vi "CRYO_MASTER_FULL_IP_old.vi"() -> ()   [LabVIEW 2017]
uses:
  USBData.lvclass
  LSI218Data.lvclass
  LSI336Data.lvclass
  <vilib>/DAQmx/create/channels.llb/DAQmx Create Channel (DO-Digital Output).vi
  <vilib>/Analysis/NI_AALBase.lvlib
  6240AData.lvclass
  <vilib>/DAQmx/create/channels.llb/DAQmx Create Channel (AO-Voltage-Basic).vi
  <vilib>/express/express arith-compare/Formula/XNode/ExpressFormulaBlockNode.xnode
  DMMsData.lvclass
panel:
  out "Graph 12":T1(graph) caption="XY Graph"
  out "Graph 11":T1(graph) caption="XY Graph"
  out "Graph 10":T1(graph) caption="XY Graph"
  in  "Automatic \nScreenshots?":bool=TRUE
  in  "Frontpanel screenshots":bool
  in  "Screenshots interval":i64=3605
  in  "Record interval":i64=10
  out "Cycle #":u32=4959
  in  "Measurement Interval (s)":dbl=1.0
  in  "Stop Button":bool
  in  "?":T2(tab)=enum."DIAGRAM"
  out "RUN Identifier":string="20201002_111738_PreCooling"
  in  "Base Path (screenshots)":path=path "C:/LabVIEW/DATA/Google/TUCAN Experiments/KEK_cryotests_2019-2020/data/screenshots"
  out "error out (USB6210/6218 AOUT)":errorcluster
  in  "AOUT 1 Label":string="KIKUSUI_I"
  in  "AOUT 0 Label":string="KIKUSUI_V"
  in  "DOUT Labels":string[](array[string])=["D_V1_NO", "D_V2_NC", "D_CV1"]
  in  "AOUT for Current CTRL":tag="Dev1/ao1"
  in  "AOUT For Voltage CTRL":tag="Dev1/ao0"
  out "AO task out":refnum<k21>="20201002_111738_PreCooling_AO"
  in  "Analog Out ON?":bool=TRUE
  in  "InstName (USB6218)":string="USB6218"
  in  "USB6218 Config":T3(array[cluster])=[{"Label"="F_1", "FileFormat"="%5.5f", "Active?"=TRUE, "Physical CH"="Dev1/ai0", " terminal\n type"=10083, "ConversionType"={"Type"=enum."SimpleProp", "ConversionParameters"=[0.0, 5.0, 0.0, 500.0]}, "VoltageLimits"=[0.0, 5.0]}, {"Label"="F_2", "FileFormat"="%5.5f", "Active?"=TRUE, "Physical CH"="Dev1/ai1", " terminal\n type"=10083, "ConversionType"={"Type"=enum."SimpleProp", "ConversionParameters"=[0.0, 5.0, 0.0, 200.0]}, "VoltageLimits"=[0.0, 5.0]}, {"Label"="F_3", "FileFormat"="%5.5f", "Active?"=TRUE, "Physical CH"="Dev1/ai2", " terminal\n type"=10083, "ConversionType"={"Type"=enum."SimpleProp", "ConversionParameters"=[0.0, 5.0, 0.0, 200.0]}, "VoltageLimits"=[0.0, 5.0]}, {"Label"="F_4", "FileFormat"="%5.5f", "Active?"=TRUE, "Physical CH"="Dev1/ai3", " terminal\n type"=10083, "ConversionType"={"Type"=enum."SimpleProp", "ConversionParameters"=[0.0, 5.0, 0.0, 500.0]}, "VoltageLimits"=[0.0, 5.0]}, {"Label"="F_5", "FileFormat"="%5.5f", "Active?"=TRUE, "Physical CH"="Dev1/ai4", " terminal\n type"=10083, "ConversionType"={"Type"=enum."SimpleProp", "ConversionParameters"=[0.0, 5.0, 0.0, 500.0]}, "VoltageLimits"=[0.0, 5.0]}, {"Label"="I_CV", "FileFormat"="%3.5f", "Active?"=TRUE, "Physical CH"="Dev1/ai5", " terminal\n type"=10083, "ConversionType"={"Type"=enum."Raw", "ConversionParameters"=[0.0, 0.0, 0.0, 0.0]}, "VoltageLimits"=[0.0, 10.0]}, {"Label"="CV1_answer", "FileFormat"="%3.5f", "Active?"=TRUE, "Physical CH"="Dev1/ai6", " terminal\n type"=10083, "ConversionType"={"Type"=enum."SimpleProp", "ConversionParameters"=[1.0, 5.0, 0.0, 100.0]}, "VoltageLimits"=[0.0, 5.0]}] {"terminal\n type" items=["Default"=-1, "RSE"=10083, "NRSE"=10078, "Differential"=10106, "Pseudodifferential"=12529]}
  out "error out (USB6218)":errorcluster
  out "error out (USB6210/6218 DOUT)":errorcluster
  out "DOUT task out":refnum<k21>="20201002_111738_DO"
  in  "DOUT Physical CH":tag[](array[tag])=["Dev1/port1/line0", "Dev1/port1/line1", "Dev1/port1/line2"]
  in  "Digital Out ON?":bool=TRUE
  in  "USB6210 Config":T3(array[cluster])=[{"Label"="P_ins", "FileFormat"="%5.5e", "Active?"=TRUE, "Physical CH"="Dev2/ai0", " terminal\n type"=10083, "ConversionType"={"Type"=enum."CC-10_LOG", "ConversionParameters"=[0.5, 9.0, 0.0, 1.0]}, "VoltageLimits"=[0.0, 10.0]}, {"Label"="P_4Kres", "FileFormat"="%5.5e", "Active?"=TRUE, "Physical CH"="Dev2/ai1", " terminal\n type"=10083, "ConversionType"={"Type"=enum."SimpleProp", "ConversionParameters"=[1.0, 5.0, 0.0, 200000.0]}, "VoltageLimits"=[0.0, 5.0]}, {"Label"="P_3HeIN", "FileFormat"="%5.5e", "Active?"=TRUE, "Physical CH"="Dev2/ai2", " terminal\n type"=10083, "ConversionType"={"Type"=enum."SimpleProp", "ConversionParameters"=[1.0, 5.0, 0.0, 200000.0]}, "VoltageLimits"=[0.0, 5.0]}, {"Label"="P_SldRTN", "FileFormat"="%5.5e", "Active?"=TRUE, "Physical CH"="Dev2/ai3", " terminal\n type"=10083, "ConversionType"={"Type"=enum."SimpleProp", "ConversionParameters"=[1.0, 5.0, 0.0, 200000.0]}, "VoltageLimits"=[0.0, 5.0]}, {"Label"="P_3Hepot", "FileFormat"="%5.5e", "Active?"=TRUE, "Physical CH"="Dev2/ai4", " terminal\n type"=10083, "ConversionType"={"Type"=enum."SimpleProp", "ConversionParameters"=[0.0, 10.0, 0.0, 133320.0]}, "VoltageLimits"=[0.0, 10.0]}, {"Label"="P_1Kpot", "FileFormat"="%5.5e", "Active?"=TRUE, "Physical CH"="Dev2/ai5", " terminal\n type"=10083, "ConversionType"={"Type"=enum."SimpleProp", "ConversionParameters"=[0.0, 10.0, 0.0, 133320.0]}, "VoltageLimits"=[0.0, 10.0]}, {"Label"="P_Dewar", "FileFormat"="%5.5e", "Active?"=TRUE, "Physical CH"="Dev2/ai6", " terminal\n type"=10083, "ConversionType"={"Type"=enum."SimpleProp", "ConversionParameters"=[1.0, 5.0, 0.0, 200000.0]}, "VoltageLimits"=[0.0, 5.0]}, {"Label"="DP_HEX4", "FileFormat"="%5.5e", "Active?"=TRUE, "Physical CH"="Dev2/ai7", " terminal\n type"=10083, "ConversionType"={"Type"=enum."SimpleProp", "ConversionParameters"=[1.0, 5.0, 0.0, 1000.0]}, "VoltageLimits"=[0.0, 5.0]}, {"Label"="DP_HEX5", "FileFormat"="%5.5e", "Active?"=TRUE, "Physical CH"="Dev2/ai8", " terminal\n type"=10083, "ConversionType"={"Type"=enum."SimpleProp", "ConversionParameters"=[1.0, 5.0, 0.0, 20000.0]}, "VoltageLimits"=[0.0, 5.0]}, {"Label"="L1", "FileFormat"="%5.5f", "Active?"=TRUE, "Physical CH"="Dev2/ai9", " terminal\n type"=10083, "ConversionType"={"Type"=enum."SimpleProp", "ConversionParameters"=[0.0, 10.0, 0.0, 100.0]}, "VoltageLimits"=[0.0, 10.0]}, {"Label"="L2-1", "FileFormat"="%5.5f", "Active?"=TRUE, "Physical CH"="Dev2/ai10", " terminal\n type"=10083, "ConversionType"={"Type"=enum."SimpleProp", "ConversionParameters"=[0.0, 10.0, 0.0, 100.0]}, "VoltageLimits"=[0.0, 10.0]}, {"Label"="L2-2", "FileFormat"="%5.5f", "Active?"=TRUE, "Physical CH"="Dev2/ai11", " terminal\n type"=10083, "ConversionType"={"Type"=enum."SimpleProp", "ConversionParameters"=[0.0, 10.0, 0.0, 100.0]}, "VoltageLimits"=[0.0, 10.0]}, {"Label"="L3", "FileFormat"="%5.5f", "Active?"=TRUE, "Physical CH"="Dev2/ai12", " terminal\n type"=10083, "ConversionType"={"Type"=enum."SimpleProp", "ConversionParameters"=[0.0, 10.0, 0.0, 100.0]}, "VoltageLimits"=[0.0, 10.0]}, {"Label"="P_HEX7OUT", "FileFormat"="%5.5e", "Active?"=TRUE, "Physical CH"="Dev2/ai13", " terminal\n type"=10083, "ConversionType"={"Type"=enum."SimpleProp", "ConversionParameters"=[1.0, 5.0, 0.0, 200000.0]}, "VoltageLimits"=[0.0, 5.0]}, {"Label"="P_IPHe", "FileFormat"="%5.5e", "Active?"=TRUE, "Physical CH"="Dev2/ai14", " terminal\n type"=10083, "ConversionType"={"Type"=enum."CC-10_LOG", "ConversionParameters"=[0.5, 9.0, 0.0, 1.0]}, "VoltageLimits"=[0.0, 10.0]}] {"terminal\n type" items=["Default"=-1, "RSE"=10083, "NRSE"=10078, "Differential"=10106, "Pseudodifferential"=12529]}
  in  "RUN label":string="PreCooling"
  in  "Base Path":path=path "C:/LabVIEW/DATA/Precooling/ScreenShot"
  in  "InstName (USB6210)":string="USB6210"
  out "error out (USB6210)":errorcluster
  out "File Refn USB AO":refnum<file>
  out "File Refn USB DO":refnum<file>
  out "error out (LSI336)":errorcluster
  in  "InstName (LSI336)":string="LSI336"
  in  "FileFormat (336)":string="%4.4f"
  in  "LSI336Settings(X,Y)":T4(array[cluster])=[{"LSIName"="LSi336X", "Labels"=["T1K3-1", "T1K3-2", "T3He5", "T3He8"], "SensorLocations"=[enum."T1K3-1", enum."T1K3-2", enum."T3He5", enum."T3He8"], "Active?"=TRUE, "VISA res. name"="GPIB0::6::INSTR"}, {"LSIName"="LSi336Y", "Labels"=["T3He6-1", "T3He6-2", "T3He7-1", "T3He7-2"], "SensorLocations"=[enum."T3He6-1", enum."T3He6-2", enum."T3He7-1", enum."T3He7-2"], "Active?"=TRUE, "VISA res. name"="GPIB0::2::INSTR"}]
  in  "FileFormat (218)":string="%4.4f"
  in  "InstName (LSI218)":string="LSI218"
  in  "LSI218Settings(A-F)":T4(array[cluster])=[{"LSIName"="LSI218A", "Labels"=["T3He10", "T3He1-1", "TTH3", "TTH4", "TTH1", "TTH2", "T4He1", "T1K1"], "SensorLocations"=[enum."T3He10", enum."T3He1-1", enum."TTH3", enum."TTH4", enum."TTH1", enum."TTH2", enum."T4He1", enum."T1K1"], "Active?"=TRUE, "VISA res. name"="GPIB0::7::INSTR"}, {"LSIName"="LSI218B", "Labels"=["N.C.", "N.C.", "N.C.", "N.C.", "T3He2-1", "T3He2-2", "T3He3", "T3He1-4"], "SensorLocations"=[enum."N.C.", enum."N.C.", enum."N.C.", enum."N.C.", enum."T3He2-1", enum."T3He2-2", enum."T3He3", enum."T3He1-4"], "Active?"=TRUE, "VISA res. name"="GPIB0::4::INSTR"}, {"LSIName"="LSI218C", "Labels"=["T4He3-1", "T4He3-2", "T4He3-3", "T4He3-4", "T4He2-1", "T4He2-2", "T4He4", "T4He5"], "SensorLocations"=[enum."T4He3-1", enum."T4He3-2", enum."T4He3-3", enum."T4He3-4", enum."T4He2-1", enum."T4He2-2", enum."T4He4", enum."T4He5"], "Active?"=TRUE, "VISA res. name"="GPIB0::3::INSTR"}, {"LSIName"="LSI218D", "Labels"=["T4He6", "T4He9", "T3He1-2", "T3He1-3", "T4He7", "T4He8", "T4He10", "T1K6"], "SensorLocations"=[enum."T4He6", enum."T4He9", enum."T3He1-2", enum."T3He1-3", enum."T4He7", enum."T4He8", enum."T4He10", enum."T1K6"], "Active?"=TRUE, "VISA res. name"="GPIB0::5::INSTR"}, {"LSIName"="LSI218E", "Labels"=["TIP1", "N.C.", "TIP2", "N.C.", "TIP3", "TIP4", "TIP5", "N.C."], "SensorLocations"=[enum."TIP1", enum."N.C.", enum."TIP2", enum."N.C.", enum."TIP3", enum."TIP4", enum."TIP5", enum."N.C."], "Active?"=TRUE, "VISA res. name"="GPIB0::11::INSTR"}, {"LSIName"="LSI218F", "Labels"=["T1K2", "T1K4", "T1K5", "T3He4", "T3He9", "TIP6", "N.C.", "N.C."], "SensorLocations"=[enum."T1K2", enum."T1K4", enum."T1K5", enum."T3He4", enum."T3He9", enum."TIP6", enum."N.C.", enum."N.C."], "Active?"=TRUE, "VISA res. name"="GPIB0::8::INSTR"}]
  out "error out (LSI218)":errorcluster
  out "RUN Identifier 2":string="20201002_111738_PreCooling" caption="RUN Identifier"
  out "Graph 3":T1(graph) caption="XY Graph"
  out "Graph 1":T1(graph) caption="XY Graph"
  in  "FIle suffix 4":string="Graph4_1KPot_oscillation"
  in  "Take Screenshot! 4":bool
  in  "Take Screenshot! 3":bool
  in  "Take Screenshot! 2":bool
  in  "Take Screenshot! 1":bool
  in  "FIle suffix 3":string="Graph3_1KPot_oscillation"
  in  "FIle suffix 2":string="Graph2_1KPot_oscillation"
  in  "FIle suffix 1":string="Graph1_1KPot_oscillation"
  in  "log/linear 2":bool
  in  "Tab Control 2":T5(tab)
  in  "Plot selecter (USB6210)\n    1      2     3     4":bool[][](array[boolean])=[[TRUE, FALSE, FALSE, FALSE], [TRUE, FALSE, FALSE, FALSE], [TRUE, FALSE, FALSE, FALSE], [TRUE, FALSE, FALSE, FALSE], [TRUE, FALSE, FALSE, FALSE], [TRUE, FALSE, FALSE, FALSE], [TRUE, FALSE, FALSE, FALSE], [FALSE, TRUE, FALSE, FALSE], [FALSE, TRUE, FALSE, FALSE], [FALSE, TRUE, FALSE, FALSE], [FALSE, TRUE, FALSE, FALSE], [FALSE, TRUE, FALSE, FALSE], [FALSE, TRUE, FALSE, FALSE], [TRUE, FALSE, FALSE, FALSE], [FALSE, FALSE, FALSE, FALSE], [FALSE, FALSE, FALSE, FALSE]]
  out "All Labels (USB6210)":string[](array[string])=["P_ins", "P_4Kres", "P_3HeIN", "P_SldRTN", "P_3Hepot", "P_1Kpot", "P_Dewar", "DP_HEX4", "DP_HEX5", "L1", "L2-1", "L2-2", "L3", "P_HEX7OUT"]
  out "Last Data \n(USB6210)":dbl[](array[numeric])=[0.00015623126743967978, 102646.15993978488, 3637.6504873774197, 101891.36809168091, 4295.356268996977, 845.3614360135382, 101097.11052150725, -5.334954304017453, 66.29225516513348, 99.98613335417497, 67.02762914376657, 60.52032349741818, 48.99728244152156, 103856.45826569716] format="%#_6e"
  out "Time of Last Measurement (USB6210)":timestamp=timestamp(3684454864.3849993 s since 1904-01-01)
  out "USB6210 Status":T6(ring)=enum."Ready"
  out "Last Vol\n(USB6210)":dbl[](array[numeric])=[5.596883978015126, 3.0529231987956975, 1.0727530097475484, 3.0378273618336182, 0.32218393856863015, 0.06340844854586995, 3.021942210430145, 0.9786601827839302, 1.0132584510330267, 9.998613335417497, 6.702762914376658, 6.052032349741818, 4.899728244152156, 3.077129165313943] format="%_5f"
  out "Time of Last Measurement (USB6218)":timestamp=timestamp(3684454864.391945 s since 1904-01-01)
  out "USB6218 Status":T6(ring)=enum."Ready"
  out "Last Vol \n(USB6218)":dbl[](array[numeric])=[0.4328486013755781, 0.2856827409675284, 0.008941174623972741, -0.06513496143958923, 0.9306675842076008, -6.309670101250775e-05, -0.00046218726464117564] format="%_5f"
  out "Last Data \n(USB6218)":dbl[](array[numeric])=[43.284860137557814, 11.427309638701136, 0.3576469849589097, -6.513496143958923, 93.06675842076008, -6.309670101250775e-05, -25.011554681616026] format="%#_6e"
  out "All Labels (USB6218)":string[](array[string])=["F_1", "F_2", "F_3", "F_4", "F_5", "I_CV", "CV1_answer"]
  in  "Plot selecter (USB6218)\n    1      2     3     4":bool[][](array[boolean])=[[FALSE, FALSE, TRUE, FALSE], [FALSE, FALSE, TRUE, FALSE], [FALSE, FALSE, TRUE, FALSE], [FALSE, FALSE, TRUE, FALSE], [FALSE, FALSE, TRUE, FALSE], [FALSE, FALSE, TRUE, FALSE], [FALSE, FALSE, FALSE, FALSE], [FALSE, FALSE, TRUE, FALSE], [FALSE, FALSE, TRUE, FALSE], [FALSE, FALSE, FALSE, TRUE], [FALSE, FALSE, FALSE, TRUE], [FALSE, FALSE, FALSE, TRUE], [FALSE, FALSE, FALSE, TRUE], [FALSE, FALSE, FALSE, FALSE], [FALSE, FALSE, FALSE, FALSE], [FALSE, FALSE, FALSE, FALSE]]
  out "Time of Last Measurement (LSI218)":timestamp=timestamp(3684454864.3849993 s since 1904-01-01)
  out "LSI218 Status":T7(ring)=enum."Measuring"
  out "Last Data \nLSI218 (1)":dbl[](array[numeric])=[174.86, 119.03, 131.93, 123.27, 24.68, 25.174, 4.416, 4.607, 30.0, 0.0, 0.0, 0.0, 66.96, 49.172, 4.786, 225.14, 190.27, 196.43, 244.83, 249.59, 17.993, 18.993, 22.964, 24.809]
  out "Labels LSI218 (1)":string[](array[string])=["T3He10", "T3He1-1", "TTH3", "TTH4", "TTH1", "TTH2", "T4He1", "T1K1", "N.C.", "N.C.", "N.C.", "N.C.", "T3He2-1", "T3He2-2", "T3He3", "T3He1-4", "T4He3-1", "T4He3-2", "T4He3-3", "T4He3-4", "T4He2-1", "T4He2-2", "T4He4", "T4He5"]
  in  "Plot selecter LSI218(1)\n    1      2     3     4":bool[][](array[boolean])=[[FALSE, FALSE, FALSE, FALSE], [FALSE, FALSE, FALSE, FALSE], [FALSE, FALSE, FALSE, TRUE], [FALSE, FALSE, FALSE, TRUE], [FALSE, FALSE, FALSE, TRUE], [FALSE, FALSE, FALSE, TRUE], [FALSE, FALSE, FALSE, TRUE], [FALSE, FALSE, FALSE, TRUE], [FALSE, FALSE, FALSE, FALSE], [FALSE, FALSE, FALSE, FALSE], [FALSE, FALSE, FALSE, FALSE], [FALSE, FALSE, FALSE, FALSE], [FALSE, FALSE, FALSE, TRUE], [FALSE, FALSE, FALSE, TRUE], [FALSE, FALSE, FALSE, FALSE], [FALSE, FALSE, FALSE, FALSE], [FALSE, FALSE, FALSE, TRUE], [FALSE, FALSE, FALSE, TRUE], [FALSE, FALSE, FALSE, TRUE], [FALSE, FALSE, FALSE, TRUE], [FALSE, FALSE, FALSE, TRUE], [FALSE, FALSE, FALSE, TRUE], [FALSE, FALSE, FALSE, TRUE], [FALSE, FALSE, FALSE, FALSE]]
  out "Active?\n (1)":bool[](array[boolean])=[TRUE, TRUE, TRUE, TRUE, TRUE, TRUE, TRUE, TRUE, TRUE, TRUE, TRUE, TRUE, TRUE, TRUE, TRUE, TRUE, TRUE, TRUE, TRUE, TRUE, TRUE, TRUE, TRUE, TRUE]
  out "Labels LSI218 (2)":string[](array[string])=["T4He6", "T4He9", "T3He1-2", "T3He1-3", "T4He7", "T4He8", "T4He10", "T1K6", "TIP1", "N.C.", "TIP2", "N.C.", "TIP3", "TIP4", "TIP5", "N.C.", "T1K2", "T1K4", "T1K5", "T3He4", "T3He9", "TIP6", "N.C.", "N.C."]
  out "Active?\n(2)":bool[](array[boolean])=[TRUE, TRUE, TRUE, TRUE, TRUE, TRUE, TRUE, TRUE, TRUE, TRUE, TRUE, TRUE, TRUE, TRUE, TRUE, TRUE, TRUE, TRUE, TRUE, TRUE, TRUE, TRUE, TRUE, TRUE]
  out "Last Data \nLSI218 (2)":dbl[](array[numeric])=[26.249, 111.49, 133.91, 219.75, 133.21, 138.02, 218.7, 58.064, 250.36, 0.0, 110.28, 688.49, 56.993, 6.89, 10.053, 688.58, 1.955, 1.89, 4.175, 2.013, 2.158, 18.589, 0.433, 0.0]
  in  "Plot selecter LSI218(2)\n    1      2     3     4":bool[][](array[boolean])=[[FALSE, FALSE, FALSE, FALSE], [FALSE, FALSE, FALSE, FALSE], [FALSE, FALSE, FALSE, FALSE], [FALSE, FALSE, FALSE, FALSE], [FALSE, FALSE, FALSE, FALSE], [FALSE, FALSE, FALSE, FALSE], [FALSE, FALSE, FALSE, FALSE], [FALSE, FALSE, FALSE, FALSE], [FALSE, FALSE, FALSE, FALSE], [FALSE, FALSE, FALSE, FALSE], [FALSE, FALSE, FALSE, FALSE], [FALSE, FALSE, FALSE, FALSE], [FALSE, FALSE, FALSE, FALSE], [FALSE, FALSE, FALSE, FALSE], [FALSE, FALSE, FALSE, FALSE], [FALSE, FALSE, FALSE, FALSE], [FALSE, FALSE, FALSE, TRUE], [FALSE, FALSE, FALSE, TRUE], [FALSE, FALSE, FALSE, TRUE], [FALSE, FALSE, FALSE, FALSE], [FALSE, FALSE, FALSE, FALSE], [FALSE, FALSE, FALSE, FALSE], [FALSE, FALSE, FALSE, FALSE], [FALSE, FALSE, FALSE, FALSE]]
  in  "Plot selecter LSI336 \n     1      2     3     4":bool[][](array[boolean])=[[FALSE, FALSE, FALSE, TRUE], [FALSE, FALSE, FALSE, TRUE], [FALSE, FALSE, FALSE, TRUE], [FALSE, FALSE, FALSE, TRUE], [FALSE, FALSE, FALSE, TRUE], [FALSE, FALSE, FALSE, TRUE], [FALSE, FALSE, FALSE, TRUE], [FALSE, FALSE, FALSE, TRUE]]
  out "Time of Last Measurement (LSI336)":timestamp=timestamp(3684454864.3849993 s since 1904-01-01)
  out "Last Data \nLSI336":dbl[](array[numeric])=[1.5337, 1.5296, 1.8153, 2.1079, 2.1163, 2.122, 2.1204, 2.1198]
  out "Active?\n(LSI336)":bool[](array[boolean])=[TRUE, TRUE, TRUE, TRUE, TRUE, TRUE, TRUE, TRUE]
  out "Labels LSI336":string[](array[string])=["T1K3-1", "T1K3-2", "T3He5", "T3He8", "T3He6-1", "T3He6-2", "T3He7-1", "T3He7-2"]
  out "LSI336 Status":T7(ring)=enum."Measuring"
  in  "log/linear 1":bool=TRUE
  out "Graph 2":T1(graph) caption="XY Graph"
  out "Graph 4":T1(graph) caption="XY Graph"
  in  "log/linear 4":bool
  in  "log/linear 3":bool
  out "RUN Identifier 3":string="20201002_111738_PreCooling" caption="RUN Identifier"
  out "RUN Identifier 4":string="20201002_111738_PreCooling" caption="RUN Identifier"
  out "Fill (false)":bool=TRUE
  in  "Fill state":bool
  out "state 1 (false)":bool=TRUE
  out "state 1":bool
  out "state 2":bool
  out "state 2 (false)":bool=TRUE
  out "Status V2 CTRL":enum16{"Pressurize", "Release"}(ring)
  out "Status V1 CTRL":enum16{"Pressurize", "Release"}(ring)
  out "Lav (%)":dbl=71.20324134668614 format="%0.2f"
  out "Lstd":dbl=0.006921328322954857 format="%0.2f"
  out "Last N M.A. Levels":dbl[](array[numeric])=[71.21069849829522, 71.21168495646573, 71.21563078793135, 71.20971204069737, 71.19803895584928, 71.19672367846871, 71.19162697956635, 71.19771013641974, 71.20247801612076, 71.19951864246737, 71.19738131717675, 71.2023136066108, 71.20675266705979, 71.20510857047677] format="%_5e"
  out "Lstd history":dbl(graph)=0.007035562623226079
  out "Lav history":dbl(graph)=71.20346447405132
  out "Target Index (L)":i32=12
  in  "Auto Fll\nHe level label":string="L3"
  out "Target Index (P)":i32=6
  in  "Auto Fll\nDewar P. label":string="P_Dewar"
  out "He Level":T8(graph)=[{"TimeArray"=[timestamp(3684373440.273899 s since 1904-01-01), timestamp(3684373441.2730346 s since 1904-01-01), timestamp(3684373442.273437 s since 1904-01-01), timestamp(3684373443.273284 s since 1904-01-01), timestamp(3684373444.272991 s since 1904-01-01), timestamp(3684373445.2752414 s since 1904-01-01), timestamp(3684373446.273977 s since 1904-01-01), timestamp(3684373447.275109 s since 1904-01-01), timestamp(3684373448.275254 s since 1904-01-01), timestamp(3684373449.2756577 s since 1904-01-01), timestamp(3684373450.4052033 s since 1904-01-01), timestamp(3684373451.404408 s since 1904-01-01), timestamp(3684373452.4054728 s since 1904-01-01), timestamp(3684373453.4055552 s since 1904-01-01)], "Filtered X"=[71.22204276382959, 71.21217818635228, 71.21283582343595, 71.19179138917168, 71.17535042443726, 71.20691707682998, 71.19244902782646, 71.21612401658533, 71.1944219432413, 71.1950795822164, 71.18389972666398, 71.2358531743215, 71.21217818503723, 71.18850319588435]}, {"TimeArray"=[timestamp(3684373440.273899 s since 1904-01-01), timestamp(3684373441.2730346 s since 1904-01-01), timestamp(3684373442.273437 s since 1904-01-01), timestamp(3684373443.273284 s since 1904-01-01), timestamp(3684373444.272991 s since 1904-01-01), timestamp(3684373445.2752414 s since 1904-01-01), timestamp(3684373446.273977 s since 1904-01-01), timestamp(3684373447.275109 s since 1904-01-01), timestamp(3684373448.275254 s since 1904-01-01), timestamp(3684373449.2756577 s since 1904-01-01), timestamp(3684373450.4052033 s since 1904-01-01), timestamp(3684373451.404408 s since 1904-01-01), timestamp(3684373452.4054728 s since 1904-01-01), timestamp(3684373453.4055552 s since 1904-01-01)], "Filtered X"=[71.21069849829522, 71.21168495646573, 71.21563078793135, 71.20971204069737, 71.19803895584928, 71.19672367846871, 71.19162697956635, 71.19771013641974, 71.20247801612076, 71.19951864246737, 71.19738131717675, 71.2023136066108, 71.20675266705979, 71.20510857047677]}] caption="XY Graph"
  in  "P_safelimit_high (Pa)":dbl=300000.0 format="%_4e"
  in  "P_safelimit_low (Pa)":dbl=100.0 format="%_4e"
  in  "Auto Fill ON?":bool
  out "Pstd history":dbl(graph)=271.0714505072834
  out "Pav history":dbl(graph)=125228.66056725154
  in  "Mov. Avg Interval":i64=4
  in  "V2 (N.C.)":bool
  in  "V1 (N.O.)":bool=TRUE
  in  "N for sampling":i64=7
  in  "L_low (%)":dbl=60.0 format="%_3f"
  in  "L_high (%)":dbl=80.0 format="%_3g"
  in  "P_2_low (Pa)":dbl=125000.0 format="%_4e"
  in  "P_1_low (Pa)":dbl=135000.0 format="%_4g"
  in  "P_2_high (Pa)":dbl=135000.0 format="%_4e"
  in  "P_1_high (Pa)":dbl=140000.0 format="%_4e"
  out "Dewar Pressure":T8(graph)=[{"TimeArray"=[timestamp(3684373440.273899 s since 1904-01-01), timestamp(3684373441.2730346 s since 1904-01-01), timestamp(3684373442.273437 s since 1904-01-01), timestamp(3684373443.273284 s since 1904-01-01), timestamp(3684373444.272991 s since 1904-01-01), timestamp(3684373445.2752414 s since 1904-01-01), timestamp(3684373446.273977 s since 1904-01-01), timestamp(3684373447.275109 s since 1904-01-01), timestamp(3684373448.275254 s since 1904-01-01), timestamp(3684373449.2756577 s since 1904-01-01), timestamp(3684373450.4052033 s since 1904-01-01), timestamp(3684373451.404408 s since 1904-01-01), timestamp(3684373452.4054728 s since 1904-01-01), timestamp(3684373453.4055552 s since 1904-01-01)], "Filtered X"=[126288.14675345753, 125406.72915551426, 125684.63887820412, 125234.06378922188, 125026.86502899571, 125252.15243360576, 124413.49040192305, 124206.29196931639, 125817.83836590881, 125184.73094394046, 125132.10848420773, 125707.66108196737, 125227.48582278784, 126493.70118827428]}, {"TimeArray"=[timestamp(3684373440.273899 s since 1904-01-01), timestamp(3684373441.2730346 s since 1904-01-01), timestamp(3684373442.273437 s since 1904-01-01), timestamp(3684373443.273284 s since 1904-01-01), timestamp(3684373444.272991 s since 1904-01-01), timestamp(3684373445.2752414 s since 1904-01-01), timestamp(3684373446.273977 s since 1904-01-01), timestamp(3684373447.275109 s since 1904-01-01), timestamp(3684373448.275254 s since 1904-01-01), timestamp(3684373449.2756577 s since 1904-01-01), timestamp(3684373450.4052033 s since 1904-01-01), timestamp(3684373451.404408 s since 1904-01-01), timestamp(3684373452.4054728 s since 1904-01-01), timestamp(3684373453.4055552 s since 1904-01-01)], "Filtered X"=[125428.10696888957, 125511.97316498918, 125422.7625555792, 125653.39464409945, 125338.074212984, 125299.43003250686, 124981.6429134366, 124724.69995846022, 124922.4432926885, 124905.58792027218, 125085.24244084334, 125460.58471900609, 125312.99658322585, 125640.23914430931]}] caption="XY Graph"
  out "Last N M.A. Pressures":dbl[](array[numeric])=[125428.10696888957, 125511.97316498918, 125422.7625555792, 125653.39464409945, 125338.074212984, 125299.43003250686, 124981.6429134366, 124724.69995846022, 124922.4432926885, 124905.58792027218, 125085.24244084334, 125460.58471900609, 125312.99658322585, 125640.23914430931] format="%_5e"
  out "Pav (Pa)":dbl=125263.36989652073 format="%0.4e"
  out "Pstd":dbl=291.18311466125465 format="%0.4e"
  out "File Refn DewarCTRL":refnum<file>
  out "Error Out (Dewar CTRL":errorcluster
  in  "update values":bool
  out "Monitor Current (mA)":dbl=-0.5520142344653531 min=0.0 max=1.9 format="%_4e"
  in  "update current":bool
  out "USB AOUT":dbl[](array[numeric])=[12.0, 4.0, 0.18461538461538463, 0.06969546425555169]
  out "Graph 7":T9(graph) caption="XY Graph"
  in  "upper limit (V)\n (Kikusui)":dbl=12.0 format="%_3f"
  in  "lower limit (V) \n(Kikusui)":dbl format="%_3f"
  in  "lower limit (mA) \n(Kikusui)":dbl=4.0 format="%_3f"
  in  "upper limit (mA)\n (Kikusui)":dbl=40.0 format="%_3f"
  in  "lower limit (mA)":dbl=4.0 format="%_3f"
  in  "SetCurrent 2 (mA)":dbl=4.0 min=4.0 max=500.0 format="%_3f"
  in  "upper limit (mA)":dbl=500.0 format="%_3f"
  out "error out (KIKUSI CTRL)":errorcluster
  out "ActualVoltage (V)":dbl[](array[numeric]) format="%_6g"
  out "ActualCurrent (A)":dbl[](array[numeric])=[0.01, 0.0] format="%_3e"
  in  "SetCurrent 1 (mA)":dbl=4.0 min=4.0 max=500.0 format="%_3g"
  in  "Output\n (ADCMT)":bool[](array[boolean])=[FALSE, FALSE]
  out "error out (ADCMT6420A)":errorcluster
  in  "Voltage limits (V)":dbl[](array[numeric])=[12.0, 12.0] format="%_3f"
  in  "CtrlLabels":string[](array[string])=["CV2", "CV3"]
  in  "VISA":refnum<visa-resource-name>[](array[refnum])=["GPIB0::1::INSTR", "GPIB0::12::INSTR"]
  out "Initialized?":bool
  in  "InstName":string="ADCMT6240"
  out "Graph 6":T8(graph)=[{"TimeArray"=[timestamp(3684448950.65012 s since 1904-01-01), timestamp(3684448954.168732 s since 1904-01-01), timestamp(3684448960.15376 s since 1904-01-01)], "Filtered X"=[0.8, 0.8, 0.01]}, {"TimeArray"=[timestamp(3684448950.65012 s since 1904-01-01), timestamp(3684448954.168732 s since 1904-01-01), timestamp(3684448960.15376 s since 1904-01-01)], "Filtered X"=[0.0, 0.0, 0.0]}, {"TimeArray"=[timestamp(3684448950.65012 s since 1904-01-01), timestamp(3684448954.168732 s since 1904-01-01), timestamp(3684448960.15376 s since 1904-01-01)], "Filtered X"=[0.8, 0.8, 0.01]}, {"TimeArray"=[timestamp(3684448950.65012 s since 1904-01-01), timestamp(3684448954.168732 s since 1904-01-01), timestamp(3684448960.15376 s since 1904-01-01)], "Filtered X"=[0.0, 0.0, 0.0]}] caption="XY Graph"
  in  "Initialize":bool
  in  "CONTROL KIKUSUI?":bool=TRUE
  in  "OUTPUT\n(Kikusui)":bool
  in  "Set Voltage (V)\n (Kikusui)":dbl=12.0 min=0.0 max=12.0 format="%_3g"
  in  "Set Current (mA)\n (Kikusui)":dbl=4.0 min=4.0 max=40.0 format="%_3g"
  out "RUN Identifier 5":string="20201002_111738_PreCooling" caption="RUN Identifier"
  in  "Measure DMMs?":bool
  out "DMMsLabels":string[](array[string])=["V_H2", "V_H4", "I_H2", "I_H4"]
  out "Active?":bool[](array[boolean])=[TRUE, FALSE, TRUE, FALSE]
  out "DMM LastMeasurements":dbl[](array[numeric])=[2.6334599999999997e-05, 0.0, 0.0, 0.0]
  out "Graph DMMs 2":T1(graph) caption="XY Graph"
  out "DMMFileName":string="20201001_162428_PreCooling_DMMs_20201001_162516.csv"
  out "error out (DMMs)":errorcluster
  out "cycle # (DMMs)":i32=10009
  in  "DMMsConfig":T10(array[cluster])=[{"Label"="V_H2", "Active?"=TRUE, "VISA resource name"="GPIB0::22::INSTR", "Device"=enum."Agilent34401A", "Measurement"=enum."DC Volts", "FileFormat"="%4.6e"}, {"Label"="V_H4", "Active?"=FALSE, "VISA resource name"="USB0::0x1334::0x0204::262800451::INSTR", "Device"=enum."ADCMT7351", "Measurement"=enum."DC Volts", "FileFormat"="%4.6e"}, {"Label"="I_H2", "Active?"=TRUE, "VISA resource name"="USB0::0x1334::0x0204::262800066::INSTR", "Device"=enum."ADCMT7351", "Measurement"=enum."DC Currents", "FileFormat"="%4.4e"}, {"Label"="I_H4", "Active?"=FALSE, "VISA resource name"="GPIB0::23::INSTR", "Device"=enum."HP3478A", "Measurement"=enum."DC Currents", "FileFormat"="%4.4e"}]
  in  "Measurement Interval DMMs (ms)":i64=500
  in  "InstName DMMs":string="DMMs"
  in  "Initialize (DMMs)":bool
  out "Graph DMMs 1":T1(graph) caption="XY Graph"
  out "error out (DMM graphs)":errorcluster
  in  "Sample #":i32=5
  in  "IPHe pressure":string="P_IPHe"
  out "P (IPHe)":dbl=102813.89149070326 format="%_4e"
  out "P_IPHe":dbl=102813.89149070326 format="%_4e"
  out "P_HEX7OUT":dbl=102813.89149070326 format="%_4e"
  out "P (HEX7 out)":dbl=102813.89149070326 format="%_4e"
  out "DP HEX5":dbl=83.0651823977413 format="%_4e"
  out "DP_HEX5":dbl=83.0651823977413 format="%_4e"
  in  "Diff pressure HEX5":string="DP_HEX5"
  out "3He pot level":dbl=100.01835834612064 format="%_4f"
  in  "3He pot":string="L1"
  out "He level (3He)":dbl(slide)=100.01835834612064 scale=0.0..100.0
  out "He level (1K) b":dbl(slide)=60.44995659847142 scale=0.0..100.0
  out "He level (1K)":dbl(slide)=66.98422510636897 scale=0.0..100.0
  out "He level (4K)":dbl(slide)=48.990048499529806 scale=0.0..100.0
  out "1K pot(b1)":dbl=60.44995659847142 format="%_4f"
  in  "1K pot (b)":string="L2-2"
  in  "1K pot level":string="L2-1"
  out "L(1K) (a1)":dbl=66.98422510636897 format="%_4f"
  in  "SensorLocation 2":T11(ring)=enum."T3He5"
  out "Temperature 2":dbl=1.7995
  out "DP HEX4":dbl=-5.3760643808830615 format="%_4e"
  in  "Diff pressure HEX4":string="DP_HEX4"
  out "V2":bool
  out "V1":bool=TRUE
  out "F5 (3He pump ex.)":dbl=93.69145685771404 format="%_4f"
  out "F4 (3He in to HEX7)":dbl=-6.1879951345084425 format="%_3f"
  out "F3 (4He rtn flw via HEX7)":dbl=0.443132092574638 format="%_4f"
  out "F1 (1K pump exhaust) flow":dbl=43.19279928269202 format="%_4f"
  out "P (Dewar)":dbl=101207.2871705193 format="%_4e"
  out "P (1K pot)":dbl=854.1288946139209 format="%_4e"
  out "P (3He pot)":dbl=4268.177149245784 format="%_4e"
  out "P (shield return)":dbl=102073.89943522238 format="%_4e"
  out "P (3He IN)":dbl=3879.377992445654 format="%_4e"
  out "P (4K reservoir)":dbl=102544.20548859666 format="%_4e"
  out "P (insulation)":dbl=0.00015646802075869302 format="%_4e"
  in  "3He pump exhaust flow":string="F_5"
  out "F_5":dbl=93.69145685771404 format="%_4f"
  in  "3He incoming flow into HEX7":string="F_4"
  out "F_4":dbl=-6.1879951345084425 format="%_4f"
  out "F_3":dbl=0.443132092574638 format="%_4f"
  in  "4He return flow from HEX7":string="F_3"
  out "F_2":dbl=11.32341237657438 format="%_4f"
  in  "Shield flow":string="F_2"
  out "P_SldRTN":dbl=102073.89943522238 format="%_4e"
  in  "3He pot pressure":string="P_3Hepot"
  out "P_3Hepot":dbl=4268.177149245784 format="%_4e"
  in  "Shield return press.":string="P_SldRTN"
  out "F_1":dbl=43.19279928269202 format="%_4f"
  in  "1K pump exhaust flow":string="F_1"
  out "P_Dewar":dbl=101207.2871705193 format="%_4e"
  in  "Dewar pressure":string="P_Dewar"
  out "P_1Kpot":dbl=854.1288946139209 format="%_4e"
  in  "1Kpot pressure":string="P_1Kpot"
  out "P_3HeIN":dbl=3879.377992445654 format="%_4e"
  in  "3He inlet pressure":string="P_3HeIN"
  in  "4K reservoir pressure":string="P_4Kres"
  out "P_4Kres":dbl=102544.20548859666 format="%_4e"
  out "P_ins":dbl=0.00015646802075869302 format="%_4e"
  in  "Insulation vacuum":string="P_ins"
  out "T3He7-1/6-2 (3He pot) 2":dbl=2.1199 format="%_4f"
  out "T3He7-1/7-2 (HEX1)":dbl=2.1206 format="%_4f"
  out "T3He6-1/6-2 (3He pot) 2":dbl=2.1224 format="%_4f"
  out "T3He6-1/6-2 (HEX1)":dbl=2.1167 format="%_4f"
  out "T1K3-1/3-2 (1K pot) 2":dbl=1.53 format="%_4f"
  out "T1K3-1/3-2 (1K pot)":dbl=1.5341 format="%_4f"
  out "T4He1 (4K reservoir )":dbl=4.418 format="%_4f"
  out "Temperature 1":dbl=25.175
  in  "SensorLocation 1":T11(ring)=enum."TTH2"
  out "TIP7":dbl format="%_4g"
  out "T3He6-2":dbl=2.1224 format="%_4g"
  out "T3He7-2":dbl=2.1199 format="%_4g"
  out "T3He6-1":dbl=2.1167 format="%_4g"
  out "T3He4":dbl=2.021 format="%_4g"
  out "T3He7-1":dbl=2.1206 format="%_4g"
  out "T3He8":dbl=2.1078 format="%_4g"
  out "T3He5":dbl=1.7995 format="%_4g"
  out "T1K3-2":dbl=1.53 format="%_4g"
  out "T1K3-1":dbl=1.5341 format="%_4g"
  out "TIP6":dbl=18.591 format="%_4g"
  out "T3He9":dbl=2.146 format="%_4g"
  out "T1K5":dbl=4.181 format="%_4g"
  out "T1K4":dbl=1.897 format="%_4g"
  out "T1K2":dbl=1.952 format="%_4g"
  out "TIP5":dbl=10.064 format="%_4g"
  out "TIP4":dbl=6.894 format="%_4g"
  out "TIP3":dbl=56.992 format="%_4g"
  out "TIP2":dbl=110.28 format="%_4g"
  out "TIP1":dbl=250.37 format="%_4g"
  out "T1K6":dbl=58.037 format="%_4g"
  out "T4He10":dbl=218.68 format="%_4g"
  out "T4He8":dbl=138.02 format="%_4g"
  out "T4He7":dbl=133.22 format="%_4g"
  out "T3He1-3":dbl=219.72 format="%_4g"
  out "T3He1-2":dbl=133.83 format="%_4g"
  out "T4He9":dbl=111.48 format="%_4g"
  out "T4He6":dbl=26.241 format="%_4g"
  out "T4He5":dbl=24.814 format="%_4g"
  out "T4He4":dbl=22.962 format="%_4g"
  out "T4He2-2":dbl=19.013 format="%_4g"
  out "T4He2-1":dbl=17.972 format="%_4g"
  out "T4He3-4":dbl=249.58 format="%_4g"
  out "T4He3-3":dbl=244.82 format="%_4g"
  out "T4He3-2":dbl=196.4 format="%_4g"
  out "T4He3-1":dbl=190.21 format="%_4g"
  out "T3He1-4":dbl=225.11 format="%_4g"
  out "T3He3":dbl=4.771 format="%_4g"
  out "T3He2-2":dbl=49.183 format="%_4g"
  out "T3He2-1":dbl=66.962 format="%_4g"
  out "T1K1":dbl=4.591 format="%_4g"
  out "T4He1":dbl=4.418 format="%_4g"
  out "TTH1":dbl=24.68 format="%_4g"
  out "TTH2":dbl=25.175 format="%_4g"
  out "TTH4":dbl=123.27 format="%_4g"
  out "TTH3":dbl=131.91 format="%_4g"
  out "T3He1-1":dbl=118.93 format="%_4g"
  out "T3He10":dbl=174.85 format="%_4g"
  out "F2 (shield flow)":dbl=11.32341237657438 format="%_4f"
  out "DP_HEX4":dbl=-5.3760643808830615 format="%_4e"
  in  "4K reservoir level":string="L3"
  out "L3":dbl=48.990048499529806 format="%_4f"
  out "RUN Identifier 6":string="20201002_111738_PreCooling" caption="RUN Identifier"
  in  "HEX7 out pressure":string="P_HEX7OUT"
  out "Series 1":string[](array[string])=["P_ins", "P_4Kres", "P_3HeIN", "P_SldRTN", "P_3Hepot", "P_1Kpot", "P_Dewar", "P_HEX7OUT"]
  out "Series 2":string[](array[string])=["DP_HEX4", "DP_HEX5", "L1", "L2-1", "L2-2", "L3"]
  out "Series 3":string[](array[string])=["F_1", "F_2", "F_3", "F_4", "F_5", "I_CV"]
  out "Series 4":string[](array[string])=["TTH3", "TTH4", "TTH1", "TTH2", "T4He1", "T1K1", "T3He2-1", "T3He2-2", "T4He3-1", "T4He3-2", "T4He3-3", "T4He3-4", "T4He2-1", "T4He2-2", "T4He4", "T1K2", "T1K4", "T1K5", "T1K3-1", "T1K3-2", "T3He5", "T3He8", "T3He6-1", "T3He6-2", "T3He7-1", "T3He7-2"]
  out "Plot errors":errorcluster
  out "LastMeasurementConfig (218)":T12(array[cluster])=[{"LSIName"="LSI218A", "Active?"=TRUE, "LastData"=[174.86, 119.03, 131.93, 123.27, 24.68, 25.174, 4.416, 4.607], "Labels"=["T3He10", "T3He1-1", "TTH3", "TTH4", "TTH1", "TTH2", "T4He1", "T1K1"]}, {"LSIName"="LSI218B", "Active?"=TRUE, "LastData"=[30.0, 0.0, 0.0, 0.0, 66.96, 49.172, 4.786, 225.14], "Labels"=["N.C.", "N.C.", "N.C.", "N.C.", "T3He2-1", "T3He2-2", "T3He3", "T3He1-4"]}, {"LSIName"="LSI218C", "Active?"=TRUE, "LastData"=[190.27, 196.43, 244.83, 249.59, 17.993, 18.993, 22.964, 24.809], "Labels"=["T4He3-1", "T4He3-2", "T4He3-3", "T4He3-4", "T4He2-1", "T4He2-2", "T4He4", "T4He5"]}, {"LSIName"="LSI218D", "Active?"=TRUE, "LastData"=[26.249, 111.49, 133.91, 219.75, 133.21, 138.02, 218.7, 58.064], "Labels"=["T4He6", "T4He9", "T3He1-2", "T3He1-3", "T4He7", "T4He8", "T4He10", "T1K6"]}, {"LSIName"="LSI218E", "Active?"=TRUE, "LastData"=[250.36, 0.0, 110.28, 688.49, 56.993, 6.89, 10.053, 688.58], "Labels"=["TIP1", "N.C.", "TIP2", "N.C.", "TIP3", "TIP4", "TIP5", "N.C."]}, {"LSIName"="LSI218F", "Active?"=TRUE, "LastData"=[1.955, 1.89, 4.175, 2.013, 2.158, 18.589, 0.433, 0.0], "Labels"=["T1K2", "T1K4", "T1K5", "T3He4", "T3He9", "TIP6", "N.C.", "N.C."]}]
  out "DataArrayConv (USB6210)":dbl[][](array[numeric])
  out "LastMeasurementConfig (336)":T12(array[cluster])=[{"LSIName"="LSi336X", "Active?"=TRUE, "LastData"=[1.5337, 1.5296, 1.8153, 2.1079], "Labels"=["T1K3-1", "T1K3-2", "T3He5", "T3He8"]}, {"LSIName"="LSi336Y", "Active?"=TRUE, "LastData"=[2.1163, 2.122, 2.1204, 2.1198], "Labels"=["T3He6-1", "T3He6-2", "T3He7-1", "T3He7-2"]}]
  out "DataArrayConv (USB6218)":dbl[][](array[numeric])
  out "TimeArray (USB6218)":timestamp[](array[timestamp])
  out "Data Array sizes (6210)":i32[](array[numeric])=[4959, 14]
  out "DataArraySize (6218)":i32[](array[numeric])=[4959, 7]
  out "TimeArray size (6218)":i32=4959
  out "TimeArray (LSI336)":timestamp[](array[timestamp])
  out "TimeArray Size (336)":i32=4959
  out "DataArray (336)":dbl[][](array[numeric])
  out "DataArray size (336)":i32[](array[numeric])=[4959, 8]
  out "LastData (LSI218)":dbl[](array[numeric])=[174.86, 119.03, 131.93, 123.27, 24.68, 25.174, 4.416, 4.607, 30.0, 0.0, 0.0, 0.0, 66.96, 49.172, 4.786, 225.14, 190.27, 196.43, 244.83, 249.59, 17.993, 18.993, 22.964, 24.809, 26.249, 111.49, 133.91, 219.75, 133.21, 138.02, 218.7, 58.064, 250.36, 0.0, 110.28, 688.49, 56.993, 6.89, 10.053, 688.58, 1.955, 1.89, 4.175, 2.013, 2.158, 18.589, 0.433, 0.0]
  out "TempSensorsLocations":T13(array[ring])=[enum."T3He10", enum."T3He1-1", enum."TTH3", enum."TTH4", enum."TTH1", enum."TTH2", enum."T4He1", enum."T1K1", enum."N.C.", enum."N.C.", enum."N.C.", enum."N.C.", enum."T3He2-1", enum."T3He2-2", enum."T3He3", enum."T3He1-4", enum."T4He3-1", enum."T4He3-2", enum."T4He3-3", enum."T4He3-4", enum."T4He2-1", enum."T4He2-2", enum."T4He4", enum."T4He5", enum."T4He6", enum."T4He9", enum."T3He1-2", enum."T3He1-3", enum."T4He7", enum."T4He8", enum."T4He10", enum."T1K6", enum."TIP1", enum."N.C.", enum."TIP2", enum."N.C.", enum."TIP3", enum."TIP4", enum."TIP5", enum."N.C.", enum."T1K2", enum."T1K4", enum."T1K5", enum."T3He4", enum."T3He9", enum."TIP6", enum."N.C.", enum."N.C.", enum."T1K3-1", enum."T1K3-2", enum."T3He5", enum."T3He8", enum."T3He6-1", enum."T3He6-2", enum."T3He7-1", enum."T3He7-2"]
  out "AllTemperatures":dbl[](array[numeric])=[174.85, 118.93, 131.91, 123.27, 24.68, 25.175, 4.418, 4.591, 30.0, 0.0, 0.0, 0.0, 66.962, 49.183, 4.771, 225.11, 190.21, 196.4, 244.82, 249.58, 17.972, 19.013, 22.962, 24.814, 26.241, 111.48, 133.83, 219.72, 133.22, 138.02, 218.68, 58.037, 250.37, 0.0, 110.28, 688.49, 56.992, 6.894, 10.064, 688.58, 1.952, 1.897, 4.181, 2.021, 2.146, 18.591, 0.433, 0.0, 1.5341, 1.53, 1.7995, 2.1078, 2.1167, 2.1224, 2.1206, 2.1199]
  out "error out (frontpanel screenshots)":errorcluster
  out "error out (graph operations)":errorcluster
  out "error out (monthly folder creation)":errorcluster={"status"=TRUE, "code"=10, "source"="Create Folder in CRYO_MASTER_FULL.vi<APPEND>\nC:\\LabVIEW\\DATA\\Google\\TUCAN Experiments\\KEK_cryotests_2019-2020\\data\\screenshots\\202010"}
  out "RUN Identifier 7":string="20201002_111738_PreCooling" caption="RUN Identifier"
  out "error out (notifier)":errorcluster
  # "GLOBAL STATUS/CONTROL"
  # "Global Settings"
  # "USB6210 Analog inputs Settings"
  # "USB6218 Analog inputs Settings"
  # "USB6218 Digital Output Settings"
  # "USB6218 Analog Output Settings"
  # "LSI218 Settings"
  # "LSI336 Settings"
  # "Graph screenshots"
  # "Configuration"
  # "Activated only when *FIll state* = TRUE"
  # "Activated only when *FIll state* = TRUE"
  # "Vavle Status"
  # "OPEN"
  # "CLOSED"
  # "ADCMT6240A Control/Status"
  # "ADCMT6240A Initialization"
  # "Set Currents (mA)"
  # "KIKUSUI PWR400H CTRL via USB6218"
  # "DMM configurations"
  # "DMM measurements"
  # "CAUTION: ADCMT 7351 does not have 4-wire resistance measurement function. \n 4-Wire Resistance --> 2-Wire Resistance wih Low Power for this device"
  # "Representative temperatures"
  # "Pressures / Flows"
  # "Labels"
  # "Values"
  # "Helium Levels"
types:
  T1 = cluster{"TimeArray":timestamp[], "DataArray":dbl[]}[]
  T2 = enum32{"NI USB CONFIG", "LSI CONFIG", "MEASUREMENT", "HE AUTO FILL", "VALVE/HEATER CTRL", "DMMs", "DIAGRAM", "(Plc. hld.)"}
  T3 = cluster{"Label":string, "FileFormat":string, "Active?":bool, "Physical CH":tag, " terminal\n type":i32, "ConversionType":cluster{"Type":enum16{"Raw", "SimpleProp", "CC-10_COMBINED", "CC-10_LOG", "LeakDet_EXP", "LeakDet_Mantissa", "Baratron"}, "ConversionParameters":dbl[]}, "VoltageLimits":dbl[]}[]
  T4 = cluster{"LSIName":string, "Labels":string[], "SensorLocations":enum16{"N.C.", "T3He1-1", "T3He1-2", "T3He1-3", "T3He1-4", "T3He2-1", "T3He2-2", "T3He3", "T3He4", "T3He5", "T3He6-1", "T3He6-2", "T3He7-1", "T3He7-2", "T3He8", "T3He9", "T3He10", "T4He1", "T4He2-1", "T4He2-2", "T4He3-1", "T4He3-2", "T4He3-3", "T4He3-4", "T4He4", "T4He5", "T4He6", "T4He7", "T4He8", "T4He9", "T4He10", "T1K1", "T1K2", "T1K3-1", "T1K3-2", "T1K4", "T1K5", "T1K6", "TIP1", "TIP2", "TIP3", "TIP4", "TIP5", "TIP6", "TIP7", "TTH1", "TTH2", "TTH3", "TTH4"}[], "Active?":bool, "VISA res. name":refnum<visa-resource-name>}[]
  T5 = enum32{"USB6210", "USB6218", "Temeprature (1)", "Temperature (2)", "Temperature (3)"}
  T6 = enum16{"Intialized", "Ready", "Measuring", "Terminated"}
  T7 = enum16{"Initialized", "Ready", "Measuring", "Terminated"}
  T8 = cluster{"TimeArray":timestamp[], "Filtered X":dbl[]}[]
  T9 = cluster{"TimeArray (USB6218)":timestamp[], "DataArrayConv (USB6218)":dbl[]}[]
  T10 = cluster{"Label":string, "Active?":bool, "VISA resource name":refnum<visa-resource-name>, "Device":enum16{"Agilent34401A", "ADCMT7351", "HP3478A"}, "Measurement":enum16{"DC Volts", "DC Currents", "2-Wire Resistance", "4-Wire Resistance"}, "FileFormat":string}[]
  T11 = enum16{"N.C.", "T3He1-1", "T3He1-2", "T3He1-3", "T3He1-4", "T3He2-1", "T3He2-2", "T3He3", "T3He4", "T3He5", "T3He6-1", "T3He6-2", "T3He7-1", "T3He7-2", "T3He8", "T3He9", "T3He10", "T4He1", "T4He2-1", "T4He2-2", "T4He3-1", "T4He3-2", "T4He3-3", "T4He3-4", "T4He4", "T4He5", "T4He6", "T4He7", "T4He8", "T4He9", "T4He10", "T1K1", "T1K2", "T1K3-1", "T1K3-2", "T1K4", "T1K5", "T1K6", "TIP1", "TIP2", "TIP3", "TIP4", "TIP5", "TIP6", "TIP7", "TTH1", "TTH2", "TTH3", "TTH4"}
  T12 = cluster{"LSIName":string, "Active?":bool, "LastData":dbl[], "Labels":string[]}[]
  T13 = enum16{"N.C.", "T3He1-1", "T3He1-2", "T3He1-3", "T3He1-4", "T3He2-1", "T3He2-2", "T3He3", "T3He4", "T3He5", "T3He6-1", "T3He6-2", "T3He7-1", "T3He7-2", "T3He8", "T3He9", "T3He10", "T4He1", "T4He2-1", "T4He2-2", "T4He3-1", "T4He3-2", "T4He3-3", "T4He3-4", "T4He4", "T4He5", "T4He6", "T4He7", "T4He8", "T4He9", "T4He10", "T1K1", "T1K2", "T1K3-1", "T1K3-2", "T1K4", "T1K5", "T1K6", "TIP1", "TIP2", "TIP3", "TIP4", "TIP5", "TIP6", "TIP7", "TTH1", "TTH2", "TTH3", "TTH4"}[]
  T14 = typedef "imagedata.ctl" = cluster{"image type":i32, "image depth":i32, "image":u8[], "mask":u8[], "colors":u32[], "Rectangle":cluster{"left":i16, "top":i16, "right":i16, "bottom":i16}}
  T15 = cluster{"appended array":timestamp[], "ActualCurrentArray":dbl[]}
  T16 = cluster{"appended array":timestamp[], "SetCurrentArray":dbl[]}
  T17 = cluster{"appended array":timestamp[], "SetCurrentArray":dbl[]}[]
  T18 = cluster{"TimeArray (USB6218)":timestamp[], "DataArrayConv (USB6218)":dbl[]}
  T19 = enum16{"open", "replace", "create", "open or create", "replace or create", "replace or create with confirmation"}
  T20 = cluster{"TimeArray":timestamp[], "DataArrayConv":dbl[]}[]
  T21 = cluster{"IndexArray":i64[], "TimeArray":timestamp[], "DataArrayRaw":dbl[][], "DataArrayConv":dbl[][], "LDArray":dbl[]}
  T22 = cluster{"InstName":string, "Active?":bool, "Status":enum16{"Intialized", "Ready", "Measuring", "Terminated"}, "Labels":string[], "LabelLD":string, "FileFormat":string[], "FileFormatLD":string, "ReadLeakDet?":bool}
  T23 = cluster{"TimeArray":timestamp[], "DataArrayConv":dbl[]}
  T24 = cluster{"TimeArray":timestamp[], "M.A. Array":dbl[]}
  T25 = cluster{"TimeArray":timestamp[], "M.A. Array":dbl[]}[]
  T26 = cluster{"TimeArray":timestamp[], "DataArray":dbl[]}
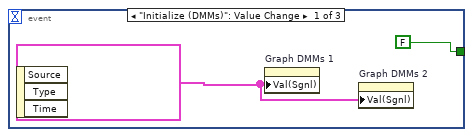
[diagram p2: hidden frame]
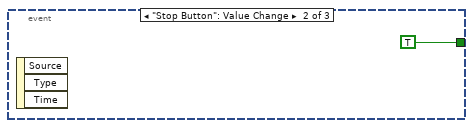
[diagram p3: hidden frame]
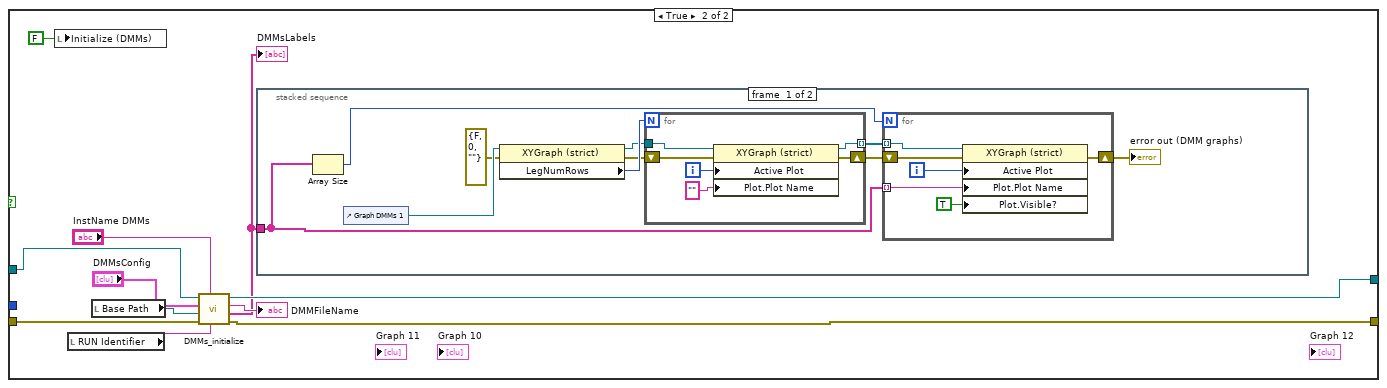
[diagram p5: hidden frame]
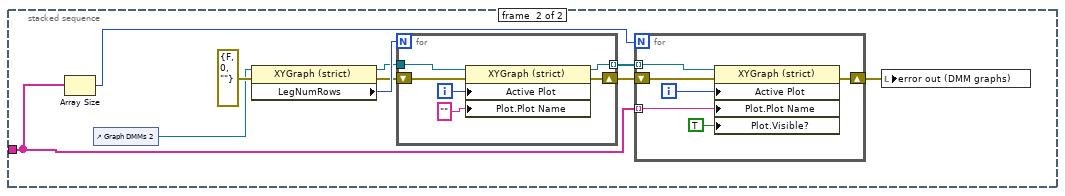
[diagram p6: hidden frame]
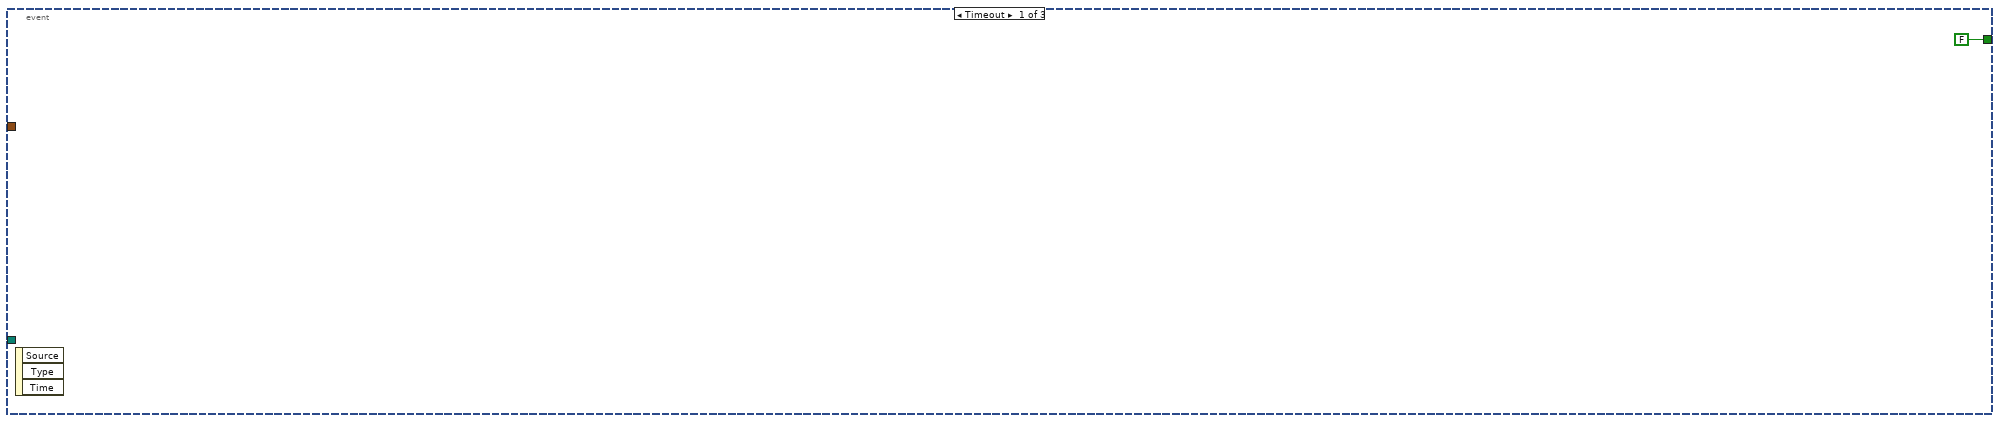
[diagram p7: hidden frame]
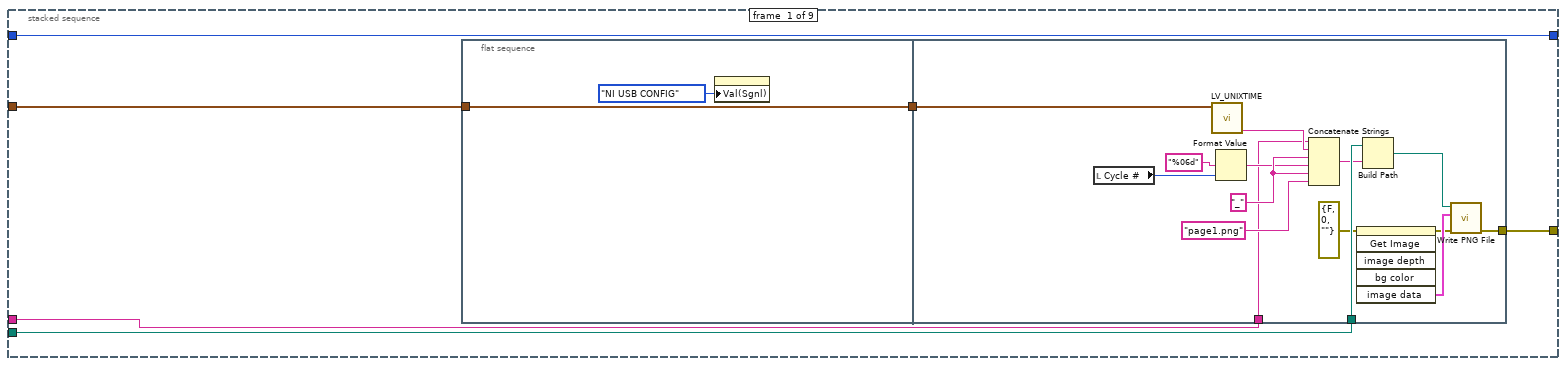
[diagram p8: hidden frame]
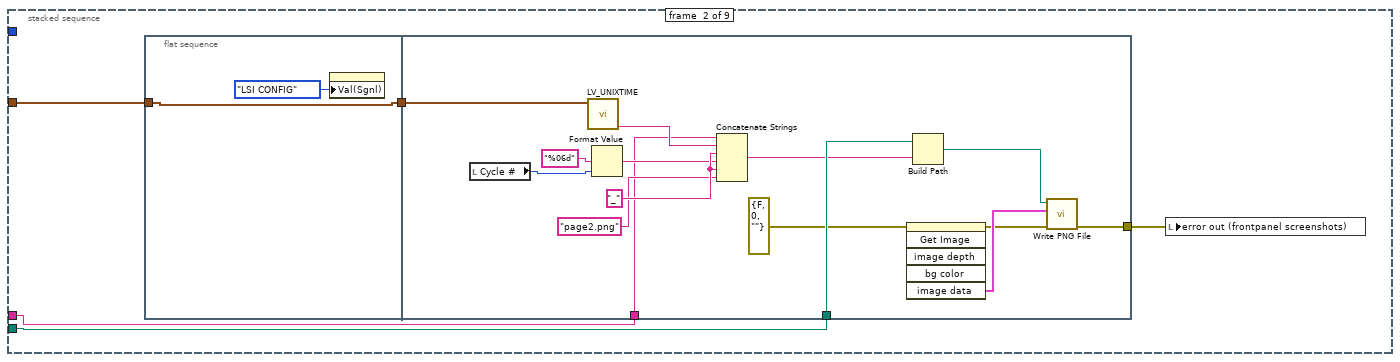
[diagram p9: hidden frame]
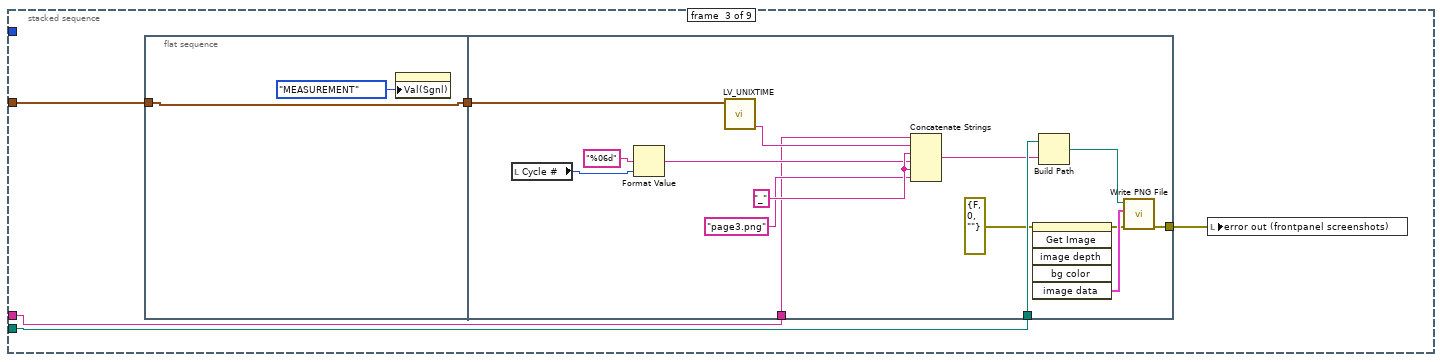
[diagram p10: hidden frame]
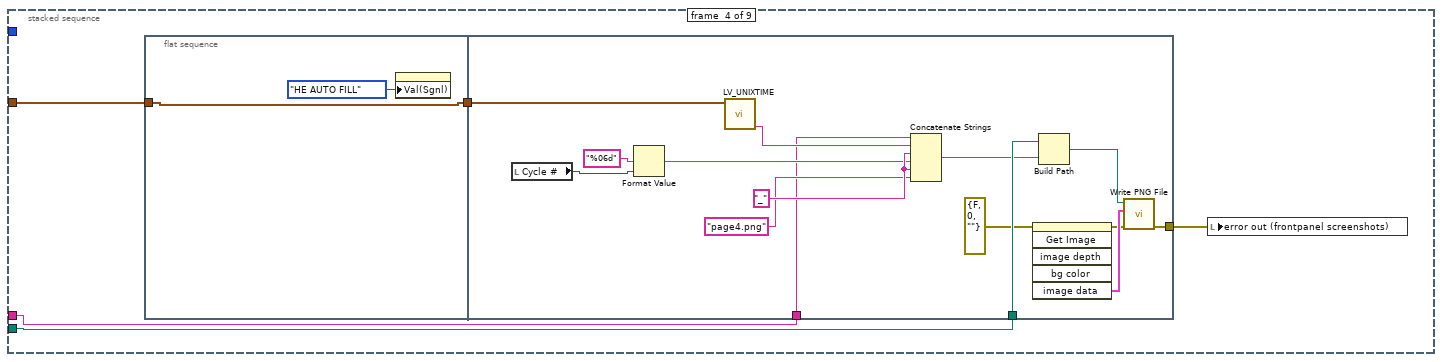
[diagram p11: hidden frame]
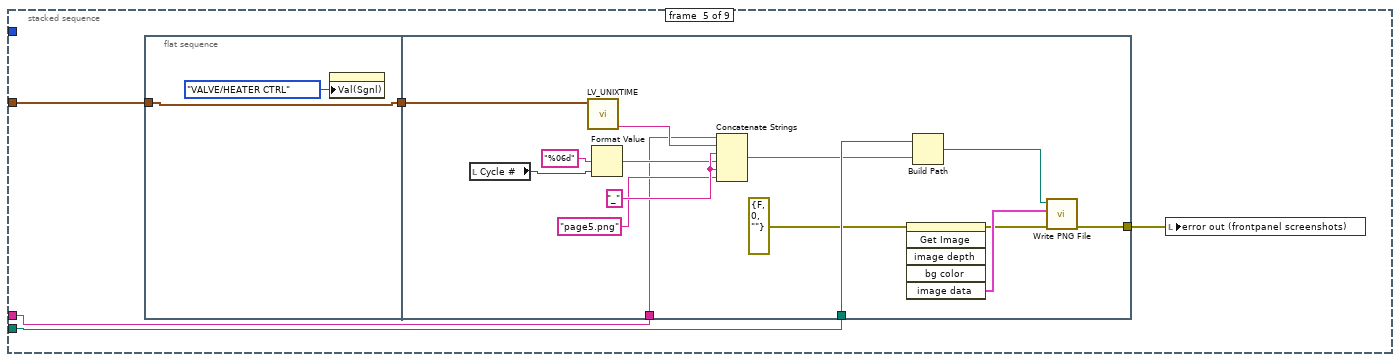
[diagram p12: hidden frame]
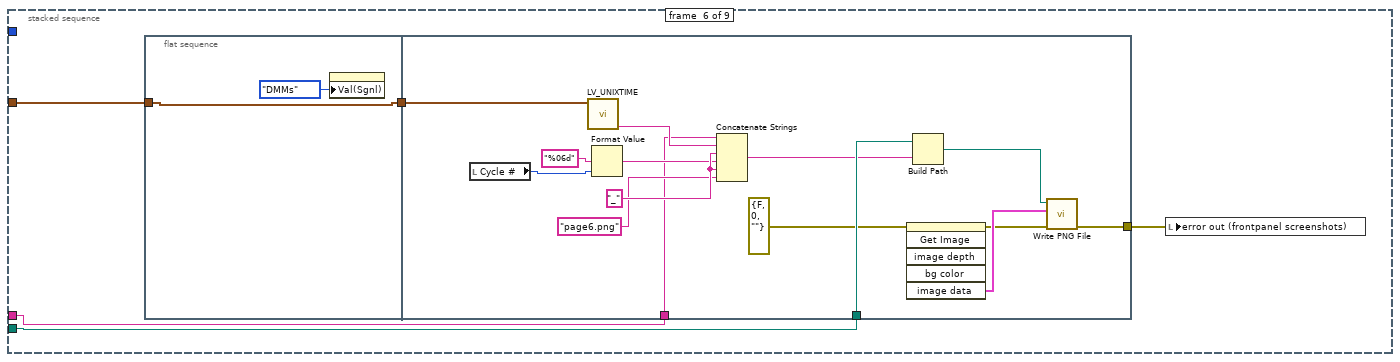
[diagram p13: hidden frame]
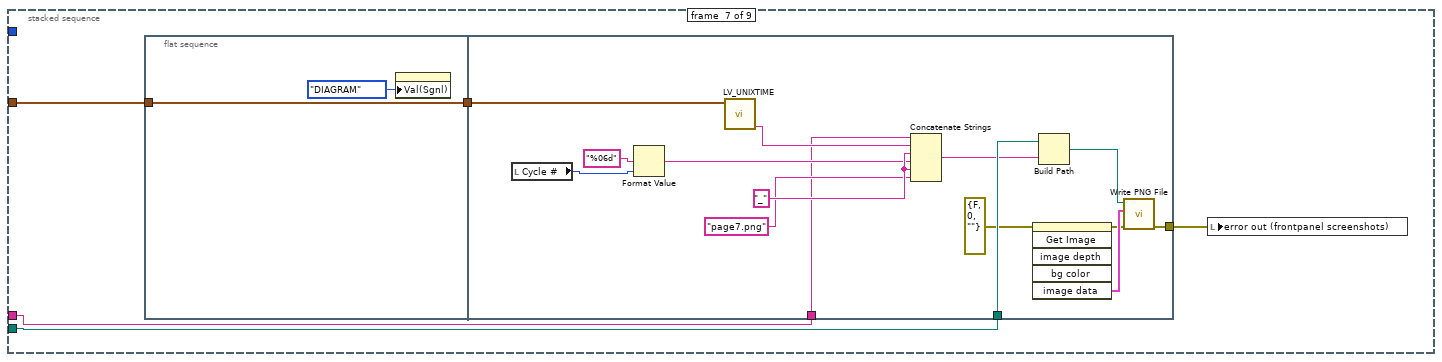
[diagram p14: hidden frame]
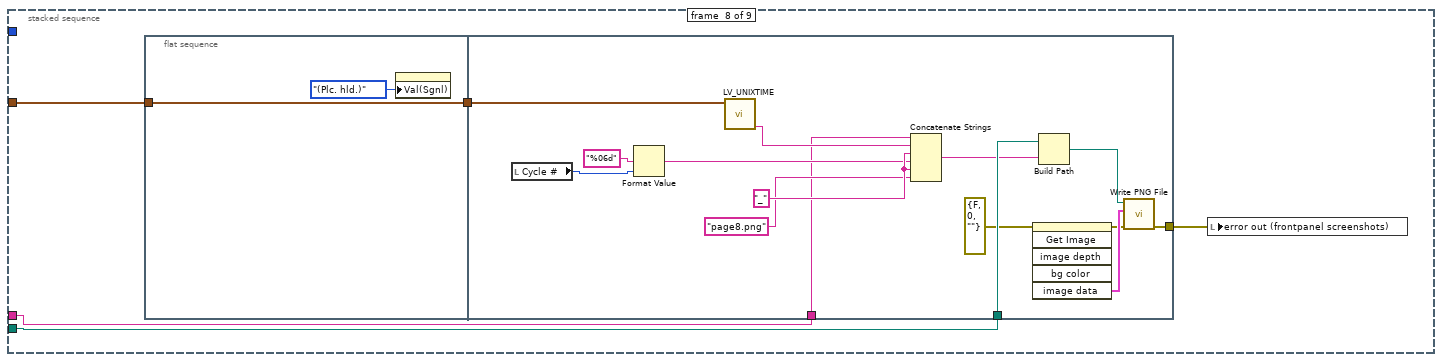
[diagram p15: hidden frame]
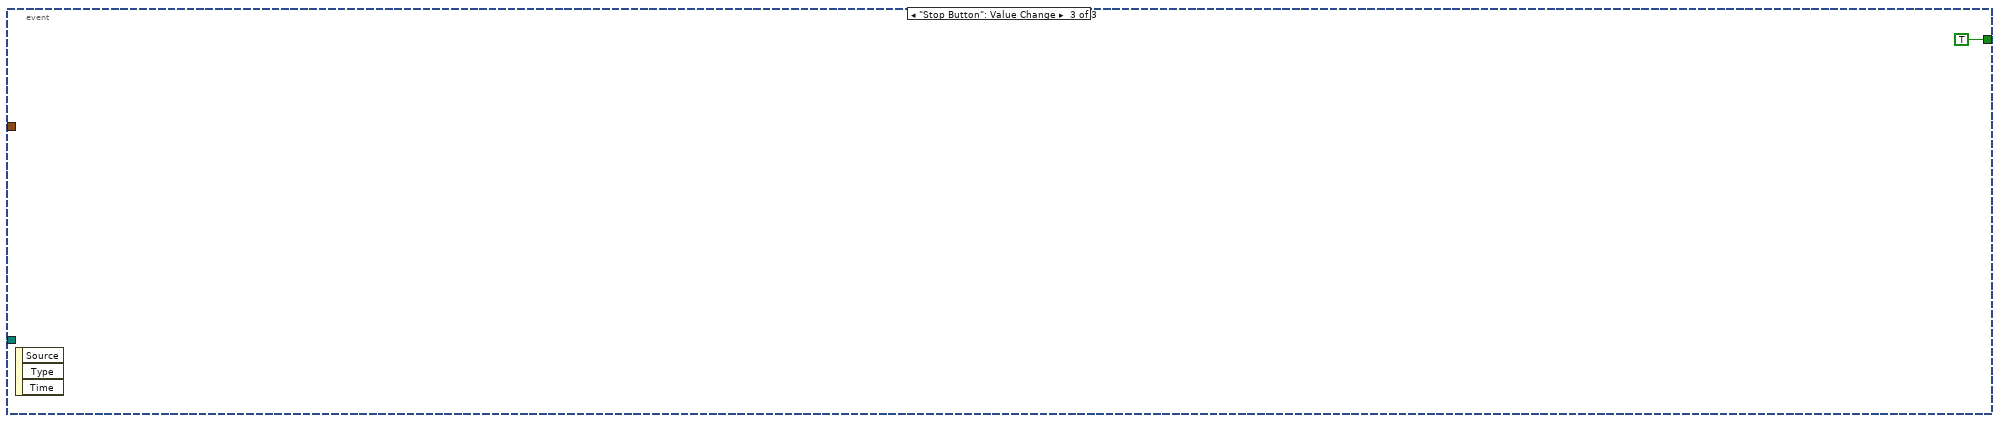
[diagram p16: hidden frame]
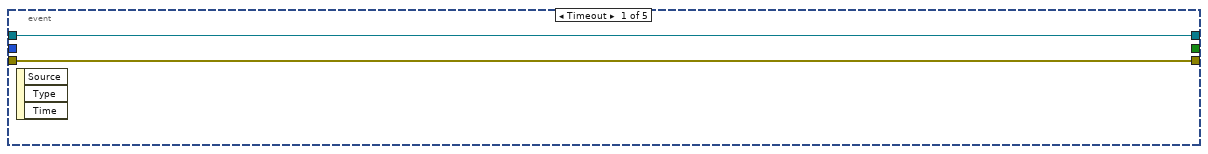
[diagram p18: hidden frame]
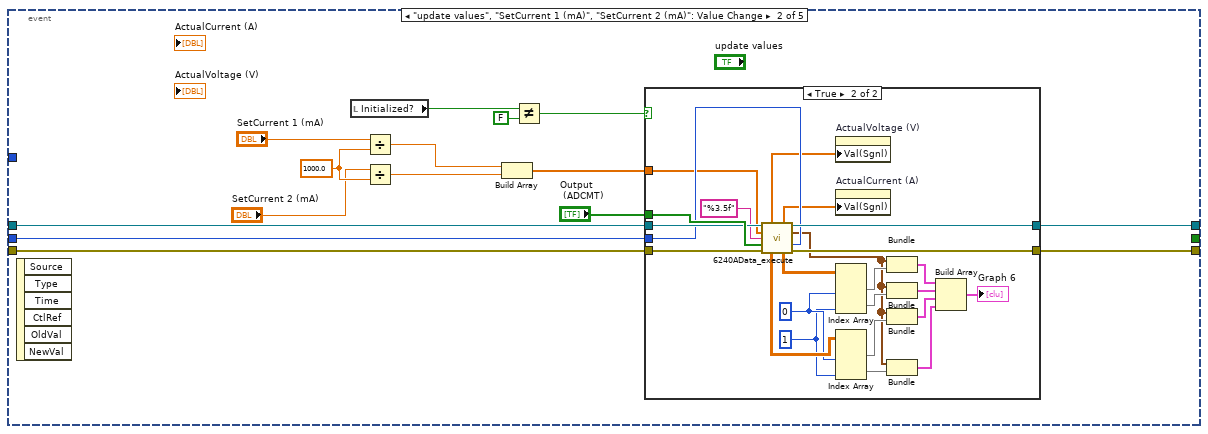
[diagram p19: hidden frame]
diagram:
  w9 = TRUE ("create if not found? (T)")
  w15 = errorcluster {"status"=FALSE, "code"=0, "source"=""} ("error in (no error)")
  n1 = while {
    stop <- w44 stop-if-true
    n2 = event shown="[5] \"Plot selecter LSI218(1)     1      2     3     4\", \"Plot selecter LSI218(2)     1      2     3     4\", \"Plot selecter (USB6210)     1      2     3     4\", \"Plot selecter LSI336       1      2     3     4\", \"Plot selecter (USB6218)     1      2     3     4\": Value Change" {
      selector: _ -> [_ _ _ _ _ _ _ _ _ _ _]
      dyn-events: _ -> [_ _ _ _ _ _ _ _ _ _ _]
      timeout: _ -> [_ _ _ _ _ _ _ _ _ _ _]
      tunnel: [_ _ _ _ _ _ _ _ _ _ TRUE] -> w44
      tunnel: [errorcluster {"status"=FALSE, "code"=0, "source"=""} ("error out") w48 _ _ _ _ w178 w195 w212 w229 errorcluster {"status"=FALSE, "code"=0, "source"=""} ("error out")] -> w40
      event Timeout {
        n3 = event-data() -> ()  [unwired: 1 in, 3 out]
      }
      event "log/linear 1": Value Change {
        n4 = event-data() -> ()  [unwired: 1 in, 6 out]
        n5 = flat-sequence {
          tunnel: [w49] -> w48
          frame #0 {
            n6 = control-ref of="Graph 1"() -> (w50:refnum<vi>)
            n7 = Boolean To (0,1)(Boolean="log/linear 1") -> (0, 1=w54:i16)
            n8 = property class="XYGraph (strict)"(reference=w50, error in=errorcluster {"status"=FALSE, "code"=0, "source"=""} ("error in (no error)"), "YScale.Mapping Mode"=w54) -> (error out=w52:errorcluster)  [unwired: 1 out]
            n9 = control-ref of="error out (USB6210)"() -> (w53:refnum<vi>)
            n10 = property class="Clust (strict)"(reference=w53, "Val(Sgnl)"=w52) -> (error out=w49:errorcluster)  [unwired: 1 in, 1 out]
          }
        }
      }
      event "log/linear 2": Value Change {
        n11 = event-data() -> ()  [unwired: 1 in, 6 out]
        n12 = flat-sequence {
          frame #0 {
            n13 = control-ref of="Graph 2"() -> (w58:refnum<vi>)
            n14 = Boolean To (0,1)(Boolean="log/linear 2") -> (0, 1=w60:i16)
            n15 = property class="XYGraph (strict)"(reference=w58, error in=errorcluster {"status"=FALSE, "code"=0, "source"=""} ("error in (no error)"), "YScale.Mapping Mode"=w60) -> (error out=w59:errorcluster)  [unwired: 1 out]
            n16 = control-ref of="error out (USB6210)"() -> (w57:refnum<vi>)
            n17 = property class="Clust (strict)"(reference=w57, "Value"=w59) -> ()  [unwired: 1 in, 2 out]
          }
        }
      }
      event "log/linear 3": Value Change {
        n18 = event-data() -> ()  [unwired: 1 in, 6 out]
        n19 = flat-sequence {
          frame #0 {
            n20 = control-ref of="Graph 3"() -> (w62:refnum<vi>)
            n21 = Boolean To (0,1)(Boolean="log/linear 3") -> (0, 1=w66:i16)
            n22 = property class="XYGraph (strict)"(reference=w62, error in=errorcluster {"status"=FALSE, "code"=0, "source"=""} ("error in (no error)"), "YScale.Mapping Mode"=w66) -> (error out=w65:errorcluster)  [unwired: 1 out]
            n23 = control-ref of="error out (USB6210)"() -> (w64:refnum<vi>)
            n24 = property class="Clust (strict)"(reference=w64, "Value"=w65) -> ()  [unwired: 1 in, 2 out]
          }
        }
      }
      event "log/linear 4": Value Change {
        n25 = event-data() -> ()  [unwired: 1 in, 6 out]
        n26 = flat-sequence {
          frame #0 {
            n27 = control-ref of="Graph 4"() -> (w68:refnum<vi>)
            n28 = Boolean To (0,1)(Boolean="log/linear 4") -> (0, 1=w72:i16)
            n29 = property class="XYGraph (strict)"(reference=w68, error in=errorcluster {"status"=FALSE, "code"=0, "source"=""} ("error in (no error)"), "YScale.Mapping Mode"=w72) -> (error out=w71:errorcluster)  [unwired: 1 out]
            n30 = control-ref of="error out (USB6210)"() -> (w70:refnum<vi>)
            n31 = property class="Clust (strict)"(reference=w70, "Value"=w71) -> ()  [unwired: 1 in, 2 out]
          }
        }
      }
      event "Plot selecter LSI218(1)\n    1      2     3     4", "Plot selecter LSI218(2)\n    1      2     3     4", "Plot selecter (USB6210)\n    1      2     3     4", "Plot selecter LSI336 \n     1      2     3     4", "Plot selecter (USB6218)\n    1      2     3     4": Value Change {
        n32 = event-data() -> ()  [unwired: 1 in, 6 out]
        n33 = local read "All Labels (USB6210)"() -> (w90:string[])
        n34 = local read "All Labels (USB6218)"() -> (w79:string[])
        n35 = local read "Labels LSI218 (1)"() -> (w92:string[])
        n36 = local read "Labels LSI218 (2)"() -> (w93:string[])
        n37 = local read "Labels LSI336"() -> (w85:string[])
        n38 = call "BuildPlotLegends.vi"("Plot selecter \n    1      2     3     4"="Plot selecter (USB6210)\n    1      2     3     4", "AllLabels"=w90) -> ("Series 4"=w102:string[], "Series 3"=w100:string[], "Series 2"=w98:string[], "Series 1"=w96:string[])  [unwired: 6 in]
        n39 = call "BuildPlotLegends_LSI218.vi"("Plot selecter (2)\n    1      2     3     5"="Plot selecter LSI218(2)\n    1      2     3     4", "Plot selecter (1)\n    1      2     3     4"="Plot selecter LSI218(1)\n    1      2     3     4", "Labels (2)"=w93, "Labels (1)"=w92) -> ("Series 4"=w103:string[], "Series 3"=w101:string[], "Series 2"=w99:string[], "Series 1"=w97:string[])  [unwired: 4 in]
        n40 = call "BuildPlotLegends.vi"("Plot selecter \n    1      2     3     4"="Plot selecter LSI336 \n     1      2     3     4", "AllLabels"=w85) -> ("Series 4"=w80:string[], "Series 3"=w81:string[], "Series 2"=w82:string[], "Series 1"=w83:string[])  [unwired: 6 in]
        n41 = call "BuildPlotLegends.vi"("Plot selecter \n    1      2     3     4"="Plot selecter (USB6218)\n    1      2     3     4", "AllLabels"=w79) -> ("Series 4"=w75:string[], "Series 3"=w74:string[], "Series 2"=w76:string[], "Series 1"=w77:string[])  [unwired: 6 in]
        n42 = Build Array (concatenate)(w98, w99, w82, w76) -> (w87:string[])
        "Series 2" <- w87
        n43 = Build Array (concatenate)(w100, w101, w81, w74) -> (w88:string[])
        "Series 3" <- w88
        n44 = Build Array (concatenate)(w102, w103, w80, w75) -> (w89:string[])
        "Series 4" <- w89
        n45 = Build Array (concatenate)(w96, w97, w83, w77) -> (w86:string[])
        "Series 1" <- w86
        n46 = stacked-sequence {
          tunnel: [w113 _ _ _] -> w107
          tunnel: [_ w131 _ _] -> w108
          tunnel: [_ _ w148 _] -> w106
          tunnel: [_ _ _ w165] -> w105
          tunnel: w86 -> [w111 _ _ _]
          tunnel: w87 -> [_ w129 _ _]
          tunnel: w88 -> [_ _ w146 _]
          tunnel: w89 -> [_ _ _ w163]
          frame #0 {
            n47 = Array Size(array=w111) -> (size(s)=w115:i32)
            n48 = control-ref of="Graph 1"() -> (w109:refnum<vi>)
            n49 = property class="XYGraph (strict)"(reference=w109) -> ("LegNumRows"=w110:u32)  [unwired: 1 in, 2 out]
            n50 = for {
              N: w110 -> [_]
              tunnel: w109 -> [w124]
              shift-right: [w122] -> w114
              shift-left: errorcluster {"status"=FALSE, "code"=0, "source"=""} ("error in (no error)") -> [w123]
              i -> [w126]
              n51 = property class="XYGraph (strict)"(reference=w124, error in=w123, "Active Plot"=w126, "Plot.Plot Name"="") -> (error out=w122:errorcluster)  [unwired: 1 out]
            }
            n52 = for {
              N: w115 -> [_]
              tunnel: w109 -> [w120]
              shift-right: [w118] -> w113
              shift-left: w114 -> [w119]
              tunnel: w111 -> [w117] mode=indexing
              i -> [w121]
              n53 = property class="XYGraph (strict)"(reference=w120, error in=w119, "Active Plot"=w121, "Plot.Plot Name"=w117, "Plot.Visible?"=TRUE ("Plot.Visible")) -> (error out=w118:errorcluster)  [unwired: 1 out]
            }
          }
          frame #1 {
            n54 = Array Size(array=w129) -> (size(s)=w133:i32)
            n55 = control-ref of="Graph 2"() -> (w128:refnum<vi>)
            n56 = property class="XYGraph (strict)"(reference=w128) -> ("LegNumRows"=w127:u32)  [unwired: 1 in, 2 out]
            n57 = for {
              N: w127 -> [_]
              shift-right: [w140] -> w132
              shift-left: errorcluster {"status"=FALSE, "code"=0, "source"=""} ("error in (no error)") -> [w141]
              tunnel: w128 -> [w139]
              i -> [w143]
              n58 = property class="XYGraph (strict)"(reference=w139, error in=w141, "Active Plot"=w143, "Plot.Plot Name"="") -> (error out=w140:errorcluster)  [unwired: 1 out]
            }
            n59 = for {
              N: w133 -> [_]
              shift-right: [w136] -> w131
              shift-left: w132 -> [w137]
              tunnel: w129 -> [w135] mode=indexing
              tunnel: w128 -> [w134]
              i -> [w138]
              n60 = property class="XYGraph (strict)"(reference=w134, error in=w137, "Active Plot"=w138, "Plot.Plot Name"=w135) -> (error out=w136:errorcluster)  [unwired: 1 out]
            }
          }
          frame #2 {
            n61 = Array Size(array=w146) -> (size(s)=w150:i32)
            n62 = control-ref of="Graph 3"() -> (w144:refnum<vi>)
            n63 = property class="XYGraph (strict)"(reference=w144) -> ("LegNumRows"=w145:u32)  [unwired: 1 in, 2 out]
            n64 = for {
              N: w145 -> [_]
              tunnel: w144 -> [w158]
              shift-right: [w156] -> w149
              shift-left: errorcluster {"status"=FALSE, "code"=0, "source"=""} ("error in (no error)") -> [w157]
              i -> [w160]
              n65 = property class="XYGraph (strict)"(reference=w158, error in=w157, "Active Plot"=w160, "Plot.Plot Name"="") -> (error out=w156:errorcluster)  [unwired: 1 out]
            }
            n66 = for {
              N: w150 -> [_]
              tunnel: w144 -> [w154]
              shift-right: [w152] -> w148
              shift-left: w149 -> [w153]
              tunnel: w146 -> [w151] mode=indexing
              i -> [w155]
              n67 = property class="XYGraph (strict)"(reference=w154, error in=w153, "Active Plot"=w155, "Plot.Plot Name"=w151) -> (error out=w152:errorcluster)  [unwired: 1 out]
            }
          }
          frame #3 {
            n68 = Array Size(array=w163) -> (size(s)=w167:i32)
            n69 = control-ref of="Graph 4"() -> (w161:refnum<vi>)
            n70 = property class="XYGraph (strict)"(reference=w161) -> ("LegNumRows"=w162:u32)  [unwired: 1 in, 2 out]
            n71 = for {
              N: w162 -> [_]
              tunnel: w161 -> [w175]
              shift-right: [w173] -> w166
              shift-left: errorcluster {"status"=FALSE, "code"=0, "source"=""} ("error in (no error)") -> [w174]
              i -> [w177]
              n72 = property class="XYGraph (strict)"(reference=w175, error in=w174, "Active Plot"=w177, "Plot.Plot Name"="") -> (error out=w173:errorcluster)  [unwired: 1 out]
            }
            n73 = for {
              N: w167 -> [_]
              tunnel: w161 -> [w171]
              shift-right: [w169] -> w165
              shift-left: w166 -> [w170]
              tunnel: w163 -> [w168] mode=indexing
              i -> [w172]
              n74 = property class="XYGraph (strict)"(reference=w171, error in=w170, "Active Plot"=w172, "Plot.Plot Name"=w168) -> (error out=w169:errorcluster)  [unwired: 1 out]
            }
          }
        }
        n75 = Merge Errors(w107, w108, w106, w105) -> (→"Plot errors":errorcluster)
      }
      event "Take Screenshot! 1": Value Change {
        n76 = event-data() -> ()  [unwired: 1 in, 6 out]
        n77 = flat-sequence {
          tunnel: [w179] -> w178
          frame #0 {
            n78 = flat-sequence {
              tunnel: [w180] -> w179
              frame #0 {
                w189 = "_" ("string")
                n79 = local read "RUN Identifier"() -> (w191:string)
                n80 = Get Date/Time In Seconds() -> (seconds since 1Jan1904=w186:timestamp)
                n81 = call "LV_UNIXTIME.vi"("current time"=w186) -> ("date/time string"=w190:string)  [unwired: 9 in, 1 out]
                n82 = control-ref of="Graph 1"() -> (w185:refnum<vi>)
                n83 = Concatenate Strings(w191, w189, w190, w189, "FIle suffix 1", ".png" ("string")) -> (w193:string)
                n84 = local read "Base Path"() -> (w192:path)
                n85 = invoke class="XYGraph (strict)" method="Get Image"(reference=w185, error in=errorcluster {"status"=FALSE, "code"=0, "source"=""} ("error in (no error)")) -> (error out=w181:errorcluster, "image data"=w184:T14)  [unwired: 4 in, 4 out]
                n86 = Build Path(base path=w192, name or relative path=w193) -> (appended path=w183:path)
                n87 = call <vilib>:"Write PNG File.vi"("error in (no error)"=w181, "image data"=w184, "path to PNG file"=w183) -> ("error out"=w180:errorcluster)  [unwired: 7 in, 1 out]
              }
              frame #1 {
                n88 = local write "Take Screenshot! 1"(FALSE ("Take Screenshot! 1")) -> ()
              }
            }
          }
        }
      }
      event "Take Screenshot! 2": Value Change {
        n89 = event-data() -> ()  [unwired: 1 in, 6 out]
        n90 = flat-sequence {
          tunnel: [w196] -> w195
          frame #0 {
            n91 = flat-sequence {
              tunnel: [w202] -> w196
              frame #0 {
                w206 = "_" ("string")
                n92 = local read "RUN Identifier"() -> (w208:string)
                n93 = Get Date/Time In Seconds() -> (seconds since 1Jan1904=w203:timestamp)
                n94 = call "LV_UNIXTIME.vi"("current time"=w203) -> ("date/time string"=w207:string)  [unwired: 9 in, 1 out]
                n95 = control-ref of="Graph 2"() -> (w197:refnum<vi>)
                n96 = Concatenate Strings(w208, w206, w207, w206, "FIle suffix 2", ".png" ("string")) -> (w210:string)
                n97 = local read "Base Path"() -> (w209:path)
                n98 = invoke class="XYGraph (strict)" method="Get Image"(reference=w197, error in=errorcluster {"status"=FALSE, "code"=0, "source"=""} ("error in (no error)")) -> (error out=w201:errorcluster, "image data"=w199:T14)  [unwired: 4 in, 4 out]
                n99 = Build Path(base path=w209, name or relative path=w210) -> (appended path=w198:path)
                n100 = call <vilib>:"Write PNG File.vi"("error in (no error)"=w201, "image data"=w199, "path to PNG file"=w198) -> ("error out"=w202:errorcluster)  [unwired: 7 in, 1 out]
              }
              frame #1 {
                n101 = local write "Take Screenshot! 2"(FALSE ("Take Screenshot! 1")) -> ()
              }
            }
          }
        }
      }
      event "Take Screenshot! 3": Value Change {
        n102 = event-data() -> ()  [unwired: 1 in, 6 out]
        n103 = flat-sequence {
          tunnel: [w213] -> w212
          frame #0 {
            n104 = flat-sequence {
              tunnel: [w215] -> w213
              frame #0 {
                w223 = "_" ("string")
                n105 = local read "RUN Identifier"() -> (w225:string)
                n106 = Get Date/Time In Seconds() -> (seconds since 1Jan1904=w221:timestamp)
                n107 = call "LV_UNIXTIME.vi"("current time"=w221) -> ("date/time string"=w224:string)  [unwired: 9 in, 1 out]
                n108 = control-ref of="Graph 3"() -> (w218:refnum<vi>)
                n109 = Concatenate Strings(w225, w223, w224, w223, "FIle suffix 3", ".png" ("string")) -> (w227:string)
                n110 = local read "Base Path"() -> (w226:path)
                n111 = invoke class="XYGraph (strict)" method="Get Image"(reference=w218, error in=errorcluster {"status"=FALSE, "code"=0, "source"=""} ("error in (no error)")) -> (error out=w216:errorcluster, "image data"=w214:T14)  [unwired: 4 in, 4 out]
                n112 = Build Path(base path=w226, name or relative path=w227) -> (appended path=w219:path)
                n113 = call <vilib>:"Write PNG File.vi"("error in (no error)"=w216, "image data"=w214, "path to PNG file"=w219) -> ("error out"=w215:errorcluster)  [unwired: 7 in, 1 out]
              }
              frame #1 {
                n114 = local write "Take Screenshot! 3"(FALSE ("Take Screenshot! 1")) -> ()
              }
            }
          }
        }
      }
      event "Take Screenshot! 4": Value Change {
        n115 = event-data() -> ()  [unwired: 1 in, 6 out]
        n116 = flat-sequence {
          tunnel: [w230] -> w229
          frame #0 {
            n117 = flat-sequence {
              tunnel: [w233] -> w230
              frame #0 {
                w240 = "_" ("string")
                n118 = local read "RUN Identifier"() -> (w242:string)
                n119 = Get Date/Time In Seconds() -> (seconds since 1Jan1904=w238:timestamp)
                n120 = call "LV_UNIXTIME.vi"("current time"=w238) -> ("date/time string"=w241:string)  [unwired: 9 in, 1 out]
                n121 = control-ref of="Graph 4"() -> (w234:refnum<vi>)
                n122 = Concatenate Strings(w242, w240, w241, w240, "FIle suffix 4", ".png" ("string")) -> (w244:string)
                n123 = local read "Base Path"() -> (w243:path)
                n124 = invoke class="XYGraph (strict)" method="Get Image"(reference=w234, error in=errorcluster {"status"=FALSE, "code"=0, "source"=""} ("error in (no error)")) -> (error out=w231:errorcluster, "image data"=w235:T14)  [unwired: 4 in, 4 out]
                n125 = Build Path(base path=w243, name or relative path=w244) -> (appended path=w236:path)
                n126 = call <vilib>:"Write PNG File.vi"("error in (no error)"=w231, "image data"=w235, "path to PNG file"=w236) -> ("error out"=w233:errorcluster)  [unwired: 7 in, 1 out]
              }
              frame #1 {
                n127 = local write "Take Screenshot! 4"(FALSE ("Take Screenshot! 1")) -> ()
              }
            }
          }
        }
      }
      event "Stop Button": Value Change {
        n128 = event-data() -> ()  [unwired: 1 in, 6 out]
      }
    }
    "error out (graph operations)" <- w40
    n129 = local write "Take Screenshot! 4"(FALSE ("Take Screenshot! 1")) -> ()
    n130 = local write "Take Screenshot! 1"(FALSE ("Take Screenshot! 1")) -> ()
    n131 = local write "Take Screenshot! 2"(FALSE ("Take Screenshot! 1")) -> ()
    n132 = local write "Take Screenshot! 3"(FALSE ("Take Screenshot! 1")) -> ()
    n133 = Wait (ms)(milliseconds to wait=u32 1000) -> ()  [unwired: 1 out]
  }
  n134 = while {
    shift-right: [w256] -> _
    shift-left: refnum<class "6240AData.lvclass"> refnum ("6240AData.lvclass") -> [w254]
    shift-right: [w252] -> _
    shift-left: errorcluster {"status"=FALSE, "code"=0, "source"=""} ("error in (no error)") -> [w253]
    i -> [w248]
    stop <- w255 stop-if-true
    n135 = Wait (ms)(milliseconds to wait=u32 231) -> ()  [unwired: 1 out]
    n136 = Equal?(x=w248, y=0) -> (x = y?=w250:bool)
    n137 = case shown="True" w250 {
      frame False {
      }
      frame True {
        n138 = property on="Initialized?" class="Bool (strict)"("Val(Sgnl)"=FALSE ("Value (Signaling)")) -> ()  [unwired: 2 in, 2 out]
      }
    }
    n139 = event shown="[3] \"Initialize\": Value Change" {
      selector: _ -> [_ _ _ _ _]
      dyn-events: _ -> [_ _ _ _ _]
      timeout: _ -> [_ _ _ _ _]
      tunnel: [w259 w274 _ w323 w344] -> w256
      tunnel: [_ _ _ _ TRUE ("Value (Signaling)")] -> w255
      tunnel: w254 -> [w259 w273 _ w307 w342]
      tunnel: w253 -> [w258 w272 _ w306 w340]
      tunnel: [w258 w271 _ w321 w343] -> w252
      tunnel: w248 -> [_ w270 _ _ _]
      tunnel: w248 -> [_ _ _ w315 _]
      event Timeout {
        n140 = event-data() -> ()  [unwired: 1 in, 3 out]
      }
      event "update values", "SetCurrent 1 (mA)", "SetCurrent 2 (mA)": Value Change {
        w263 = 1000.0 ("y")
        n141 = event-data() -> ()  [unwired: 1 in, 6 out]
        n142 = local read "Initialized?"() -> (w269:bool)
        n143 = Divide(x="SetCurrent 1 (mA)", y=w263) -> (x/y=w264:dbl)
        n144 = Divide(x="SetCurrent 2 (mA)", y=w263) -> (x/y=w265:dbl)
        n145 = Build Array(w264, w265) -> (w262:dbl[])
        n146 = Not Equal?(x=w269, y=FALSE) -> (x != y?=w267:bool)
        n147 = case shown="True" w267 {
          tunnel: [w276 w300] -> w274
          tunnel: "Output\n (ADCMT)" -> [_ w299]
          tunnel: w273 -> [w276 w298]
          tunnel: w272 -> [w275 w297]
          tunnel: [w275 w296] -> w271
          tunnel: w270 -> [_ w292]
          tunnel: w262 -> [_ w278]
          frame False {
          }
          frame True {
            w285 = 1 ("index (col)")
            w286 = 0 ("disabled index (col)")
            n148 = call-dynamic "6240AData_execute.vi"("6240AData in"=w298, "SetCurrent (A)"=w278, "FileFormat"="%3.5f", "Output status"=w299, "ExecutionIndex"=w292, "error in (no error)"=w297) -> ("ActualVoltage (V)"=w277:dbl[], "ActualCurrent (A)"=w291:dbl[], "6240AData out"=w300:refnum<class "6240AData.lvclass">, "appended array"=w281:timestamp[], "SetCurrentArray"=w287:dbl[][], "ActualCurrentArray"=w294:dbl[][], "error out"=w296:errorcluster)  [unwired: 3 in]
            n149 = property on="ActualVoltage (V)" class="Arr (strict)"("Val(Sgnl)"=w277) -> ()  [unwired: 2 in, 2 out]
            n150 = property on="ActualCurrent (A)" class="Arr (strict)"("Val(Sgnl)"=w291) -> ()  [unwired: 2 in, 2 out]
            n151 = Index Array(array=w294, index (col) #1=w286, index (col) #2=w285) -> (element #1=w295:dbl[], element #2=w289:dbl[])  [unwired: 2 in]
            n152 = Index Array(array=w287, index (col) #1=w286, index (col) #2=w285) -> (element #1=w283:dbl[], element #2=w280:dbl[])  [unwired: 2 in]
            n153 = Bundle("appended array"=w281, "ActualCurrentArray"=w295) -> (w290:T15)  [unwired: 1 in]
            n154 = Bundle("appended array"=w281, "ActualCurrentArray"=w289) -> (w284:T15)  [unwired: 1 in]
            n155 = Bundle("appended array"=w281, "SetCurrentArray"=w283) -> (w282:T16)  [unwired: 1 in]
            n156 = Bundle("appended array"=w281, "SetCurrentArray"=w280) -> (w279:T16)  [unwired: 1 in]
            n157 = Build Array(w290, w284, w282, w279) -> (→"Graph 6":T17)
          }
        }
      }
      event "upper limit (mA)", "lower limit (mA)": Value Change {
        n158 = event-data() -> ()  [unwired: 1 in, 6 out]
        n159 = property on="SetCurrent 1 (mA)" class="DigNum (strict)"("Maximum"="upper limit (mA)", "Minimum"="lower limit (mA)") -> ()  [unwired: 2 in, 2 out]
        n160 = property on="SetCurrent 2 (mA)" class="DigNum (strict)"("Maximum"="upper limit (mA)", "Minimum"="lower limit (mA)") -> ()  [unwired: 2 in, 2 out]
      }
      event "Initialize": Value Change {
        w317 = FALSE
        n161 = event-data() -> ()  [unwired: 1 in, 6 out]
        n162 = local read "Initialized?"() -> (w305:bool)
        n163 = case shown="True" w305 {
          tunnel: w307 -> [w333 w337]
          tunnel: w306 -> [w332 w336]
          tunnel: [w333 w335] -> w304
          tunnel: [w332 w334] -> w303
          frame False {
          }
          frame True {
            n164 = call-dynamic "6240AData_terrminate.vi"("error in (no error)"=w336, "6240AData in"=w337) -> ("error out"=w334:errorcluster, "6240AData out"=w335:refnum<class "6240AData.lvclass">)  [unwired: 8 in]
          }
        }
        n165 = property on="Initialized?" class="Bool (strict)"("Val(Sgnl)"=TRUE ("Value (Signaling)")) -> ()  [unwired: 2 in, 2 out]
        n166 = local read "SetCurrent 2 (mA)"() -> (w310:dbl)
        n167 = local read "SetCurrent 1 (mA)"() -> (w313:dbl)
        n168 = local read "RUN Identifier"() -> (w325:string)
        n169 = local read "Base Path"() -> (w326:path)
        n170 = Divide(x=w313, y=1000.0) -> (x/y=w312:dbl)
        n171 = Divide(x=w310, y=1000.0) -> (x/y=w309:dbl)
        n172 = Get Date/Time In Seconds() -> ()  [unwired: 1 out]
        n173 = call-dynamic "6240AData_initialize.vi"("6240AData in"=w304, "RunIdentifier"=w325, "InstName"="InstName", "base path"=w326, "VISA"="VISA", "error in (no error)"=w303, "CtrlLabels"="CtrlLabels", "Voltage limits (V)"="Voltage limits (V)") -> ("6240AData out"=w324:refnum<class "6240AData.lvclass">, "error out"=w322:errorcluster)  [unwired: 6 in]
        n174 = Build Array(w312, w309) -> (w308:dbl[])
        n175 = Build Array(w317, w317) -> (w316:bool[])
        n176 = call-dynamic "6240AData_execute.vi"("6240AData in"=w324, "SetCurrent (A)"=w308, "FileFormat"="%3.5f", "Output status"=w316, "ExecutionIndex"=w315, "error in (no error)"=w322) -> ("ActualVoltage (V)"=w319:dbl[], "ActualCurrent (A)"=w318:dbl[], "6240AData out"=w323:refnum<class "6240AData.lvclass">, "error out"=w321:errorcluster)  [unwired: 3 in, 3 out]
        n177 = property on="ActualVoltage (V)" class="Arr (strict)"("Val(Sgnl)"=w319) -> ()  [unwired: 2 in, 2 out]
        n178 = property on="ActualCurrent (A)" class="Arr (strict)"("Val(Sgnl)"=w318) -> ()  [unwired: 2 in, 2 out]
      }
      event "Stop Button": Value Change {
        n179 = event-data() -> ()  [unwired: 1 in, 6 out]
        n180 = local read "Initialized?"() -> (w338:bool)
        n181 = case shown="False" w338 {
          tunnel: w342 -> [w347 w359]
          tunnel: [w347 w358] -> w341
          tunnel: w340 -> [w346 w357]
          tunnel: [w346 w356] -> w339
          frame False {
          }
          frame True {
            w363 = FALSE
            n182 = local read "SetCurrent 2 (mA)"() -> (w349:dbl)
            n183 = local read "SetCurrent 1 (mA)"() -> (w353:dbl)
            n184 = Divide(x=w353, y=1000.0) -> (x/y=w351:dbl)
            n185 = Divide(x=w349, y=1000.0) -> (x/y=w348:dbl)
            n186 = Build Array(w351, w348) -> (w355:dbl[])
            n187 = Build Array(w363, w363) -> (w354:bool[])
            n188 = property on="Output\n (ADCMT)" class="Arr (strict)"("Val(Sgnl)"=w354) -> ()  [unwired: 2 in, 2 out]
            n189 = call-dynamic "6240AData_execute.vi"("6240AData in"=w359, "SetCurrent (A)"=w355, "FileFormat"="%3.5f", "Output status"=w354, "error in (no error)"=w357) -> ("ActualVoltage (V)"=w360:dbl[], "ActualCurrent (A)"=w361:dbl[], "6240AData out"=w358:refnum<class "6240AData.lvclass">, "error out"=w356:errorcluster)  [unwired: 4 in, 3 out]
            n190 = property on="ActualVoltage (V)" class="Arr (strict)"("Val(Sgnl)"=w360) -> ()  [unwired: 2 in, 2 out]
            n191 = property on="ActualCurrent (A)" class="Arr (strict)"("Val(Sgnl)"=w361) -> ()  [unwired: 2 in, 2 out]
          }
        }
        n192 = call-dynamic "6240AData_terrminate.vi"("error in (no error)"=w339, "6240AData in"=w341) -> ("error out"=w343:errorcluster, "6240AData out"=w344:refnum<class "6240AData.lvclass">)  [unwired: 8 in]
      }
    }
    "error out (ADCMT6420A)" <- w252
  }
  n193 = while {
    shift-right: [w365] -> _
    shift-left: dbl[] [] -> [w371]
    shift-right: [w368] -> _
    shift-left: timestamp[] [] -> [w370]
    i -> [w369]
    stop <- w372 stop-if-true
    n194 = Wait (ms)(milliseconds to wait=u32 225) -> ()  [unwired: 1 out]
    n195 = event shown="[4] \"update current\", \"Set Voltage (V)  (Kikusui)\", \"Set Current (mA)  (Kikusui)\": Value Change" {
      selector: _ -> [_ _ _ _ _ _ _]
      dyn-events: _ -> [_ _ _ _ _ _ _]
      timeout: _ -> [_ _ _ _ _ _ _]
      tunnel: [_ TRUE _ _ _ _ _] -> w372
      tunnel: w369 -> [_ _ _ _ w451 _ _]
      tunnel: [_ _ _ _ w450 w523 _] -> w365
      tunnel: w371 -> [_ _ _ _ w447 w523 _]
      tunnel: [w374 w384 _ _ w449 w522 w528] -> w368
      tunnel: w370 -> [w374 w384 _ _ w448 w522 w528]
      tunnel: w369 -> [_ _ w390 w413 _ _ w529]
      tunnel: [_ _ _ _ w437 _ _] -> w364
      event Timeout {
        n196 = event-data() -> ()  [unwired: 1 in, 3 out]
      }
      event "Stop Button": Value Change {
        w375 = FALSE
        n197 = event-data() -> ()  [unwired: 1 in, 3 out]
        n198 = local read "error out (USB6210/6218 DOUT)"() -> (w383:errorcluster)
        n199 = local read "error out (USB6210/6218 AOUT)"() -> (w380:errorcluster)
        n200 = property on="OUTPUT\n(Kikusui)" class="Bool (strict)"("Value"=w375) -> ()  [unwired: 2 in, 2 out]
        n201 = property on="V2 (N.C.)" class="Bool (strict)"("Val(Sgnl)"=w375) -> ()  [unwired: 2 in, 2 out]
        n202 = local read "DOUT task out"() -> (w379:refnum<k21>)
        n203 = local read "AO task out"() -> (w386:refnum<k21>)
        n204 = Build Array(w375, w375, w375) -> (w382:bool[])
        n205 = Not(x=w375) -> (.not. x?=w376:bool)
        n206 = property on="V1 (N.O.)" class="Bool (strict)"("Val(Sgnl)"=w376) -> ()  [unwired: 2 in, 2 out]
        n207 = call <vilib>:"DAQmx Clear Task.vi"("task in"=w386, "error in"=w380) -> ("error out"=w385:errorcluster)  [unwired: 13 in]
        n208 = local write "error out (USB6210/6218 AOUT)"(w385) -> ()
        n209 = call <vilib>:"DAQmx Write (Digital 1D Bool NChan 1Samp 1Line).vi"("task/channels in"=w379, "data"=w382, "timeout"=10.0, "error in"=w383) -> ("task out"=w378:refnum<k21>, "error out"=w377:errorcluster)  [unwired: 9 in, 1 out]
        n210 = call <vilib>:"DAQmx Clear Task.vi"("task in"=w378, "error in"=w377) -> ("error out"=w387:errorcluster)  [unwired: 13 in]
        n211 = local write "error out (USB6210/6218 DOUT)"(w387) -> ()
      }
      event "V1 (N.O.)": Value Change {
        n212 = event-data() -> ()  [unwired: 1 in, 3 out]
        n213 = local read "Cycle #"() -> (w393:u32)
        n214 = Greater?(x=w393, y=u32 0) -> (0:w391:bool)
        n215 = case shown="True" w391 {
          tunnel: "V1 (N.O.)" -> [_ w406]
          tunnel: w390 -> [_ w401]
          frame False {
          }
          frame True {
            n216 = Not(x=w406) -> (.not. x?=w408:bool)
            n217 = local read "error out (USB6210/6218 DOUT)"() -> (w407:errorcluster)
            n218 = property on="V2 (N.C.)" class="Bool (strict)"() -> ("Value"=w405:bool)  [unwired: 2 in, 2 out]
            n219 = property on="OUTPUT\n(Kikusui)" class="Bool (strict)"() -> ("Value"=w404:bool)  [unwired: 2 in, 2 out]
            n220 = local read "DOUT task out"() -> (w411:refnum<k21>)
            n221 = Build Array(w408, w405, w404) -> (w397:bool[])
            n222 = local read "File Refn USB DO"() -> (w402:refnum<file>)
            n223 = Boolean To (0,1)(Boolean=w397) -> (0, 1=w396:i16[])
            n224 = Initialize Array("%d" ("element"), 3 ("dimension size")) -> (w400:string[])
            n225 = call <vilib>:"DAQmx Write (Digital 1D Bool NChan 1Samp 1Line).vi"("task/channels in"=w411, "data"=w397, "timeout"=10.0, "error in"=w407) -> ("task out"=w409:refnum<k21>, "error out"=w395:errorcluster)  [unwired: 9 in, 1 out]
            n226 = local write "DOUT task out"(w409) -> ()
            n227 = Get Date/Time In Seconds() -> (seconds since 1Jan1904=w403:timestamp)
            n228 = call "FileWrite.vi"("DataArray"=w396, "Time Stamp"=w403, "Error In"=w395, "FileFormat"=w400, "Index"=w401, "refnum in"=w402) -> ("Error Out"=w394:errorcluster)  [unwired: 4 in, 1 out]
            n229 = local write "error out (USB6210/6218 DOUT)"(w394) -> ()
          }
        }
        "V1" <- "V1 (N.O.)"
      }
      event "V2 (N.C.)": Value Change {
        n230 = event-data() -> ()  [unwired: 1 in, 3 out]
        n231 = local read "Cycle #"() -> (w416:u32)
        n232 = Greater?(x=w416, y=u32 0) -> (0:w414:bool)
        n233 = case shown="True" w414 {
          tunnel: "V2 (N.C.)" -> [_ w430]
          tunnel: w413 -> [_ w422]
          frame False {
          }
          frame True {
            n234 = property on="V1 (N.O.)" class="Bool (strict)"() -> ("Value"=w429:bool)  [unwired: 2 in, 2 out]
            n235 = Not(x=w429) -> (.not. x?=w428:bool)
            n236 = local read "error out (USB6210/6218 DOUT)"() -> (w433:errorcluster)
            n237 = property on="OUTPUT\n(Kikusui)" class="Bool (strict)"() -> ("Value"=w427:bool)  [unwired: 2 in, 2 out]
            n238 = local read "DOUT task out"() -> (w434:refnum<k21>)
            n239 = Build Array(w428, w430, w427) -> (w425:bool[])
            n240 = local read "File Refn USB DO"() -> (w426:refnum<file>)
            n241 = Boolean To (0,1)(Boolean=w425) -> (0, 1=w424:i16[])
            n242 = Initialize Array("%d" ("element"), 3 ("dimension size")) -> (w419:string[])
            n243 = call <vilib>:"DAQmx Write (Digital 1D Bool NChan 1Samp 1Line).vi"("task/channels in"=w434, "data"=w425, "timeout"=10.0, "error in"=w433) -> ("task out"=w431:refnum<k21>, "error out"=w418:errorcluster)  [unwired: 9 in, 1 out]
            n244 = local write "DOUT task out"(w431) -> ()
            n245 = Get Date/Time In Seconds() -> (seconds since 1Jan1904=w423:timestamp)
            n246 = call "FileWrite.vi"("DataArray"=w424, "Time Stamp"=w423, "Error In"=w418, "FileFormat"=w419, "Index"=w422, "refnum in"=w426) -> ("Error Out"=w417:errorcluster)  [unwired: 4 in, 1 out]
            n247 = local write "error out (USB6210/6218 DOUT)"(w417) -> ()
          }
        }
        "V2" <- "V2 (N.C.)"
      }
      event "update current", "Set Voltage (V)\n (Kikusui)", "Set Current (mA)\n (Kikusui)": Value Change {
        n248 = event-data() -> ()  [unwired: 1 in, 3 out]
        n249 = case shown="True" "CONTROL KIKUSUI?" {
          tunnel: w451 -> [_ w492]
          tunnel: [w461 w485] -> w450
          tunnel: [w464 w484] -> w449
          tunnel: w448 -> [w466 w487]
          tunnel: w447 -> [w462 w486]
          tunnel: "Set Voltage (V)\n (Kikusui)" -> [_ w477]
          tunnel: "Set Current (mA)\n (Kikusui)" -> [_ w476]
          frame False {
            w463 = 0.0 ("element")
            n250 = Get Date/Time In Seconds() -> (seconds since 1Jan1904=w465:timestamp)
            n251 = local read "AO task out"() -> (w471:refnum<k21>)
            n252 = Build Array (concatenate)(w462, w463) -> (w461:dbl[])
            n253 = Build Array (concatenate)(w466, w465) -> (w464:timestamp[])
            n254 = Build Array(w463, w463) -> (w469:dbl[])
            n255 = call <vilib>:"DAQmx Write (Analog 1D DBL NChan 1Samp).vi"("task/channels in"=w471, "data"=w469, "timeout"=100.0, "error in"=errorcluster {"status"=FALSE, "code"=0, "source"=""}) -> ("task out"=w472:refnum<k21>, "error out"=w467:errorcluster)  [unwired: 9 in, 1 out]
            n256 = local write "AO task out"(w472) -> ()
            n257 = local write "error out (KIKUSI CTRL)"(w467) -> ()
          }
          frame True {
            w474 = 2 ("index")
            (unwired) 2.0 ("y")
            n258 = xnode "Formula"("X1"=w476) -> ("Result"=w481:dbl)  [unwired: 1 in, 1 out]
            n259 = Divide(x=w477, y=650.0) -> (x/y=w499:dbl)
            n260 = Multiply(x=10.0 ("y"), y=w499) -> (x*y=w479:dbl)
            n261 = In Range and Coerce(upper limit=0.4, x=w481, lower limit=0.0 ("y")) -> (coerced(x)=w478:dbl, In Range?=w480:bool)
            n262 = case shown="False" w480 {
              tunnel: w479 -> [w508 w513]
              tunnel: w478 -> [_ w512]
              tunnel: [w506 w511] -> w475
              tunnel: w477 -> [_ w510]
              tunnel: w476 -> [_ w509]
              tunnel: w477 -> [w505 _]
              tunnel: w476 -> [w504 _]
              frame False {
                n263 = Build Array(w505, w504, w508, 0.0 ("element")) -> (w506:dbl[])
              }
              frame True {
                n264 = Build Array(w510, w509, w513, w512) -> (w511:dbl[])
              }
            }
            "USB AOUT" <- w475
            n265 = local read "File Refn USB AO"() -> (w493:refnum<file>)
            n266 = Get Date/Time In Seconds() -> (seconds since 1Jan1904=w488:timestamp)
            n267 = Initialize Array("%.3f", 4 ("dimension size")) -> (w494:string[])
            n268 = local read "AO task out"() -> (w501:refnum<k21>)
            n269 = call "FileWrite.vi"("DataArray"=w475, "Time Stamp"=w488, "Error In"=errorcluster {"status"=FALSE, "code"=0, "source"=""} ("error in"), "FileFormat"=w494, "Index"=w492, "refnum in"=w493) -> ("Error Out"=w490:errorcluster, "Byte Stream File Refnum"=w489:refnum<file>)  [unwired: 4 in]
            n270 = Build Array (concatenate)(w487, w488) -> (w484:timestamp[])
            n271 = local write "File Refn USB AO"(w489) -> ()
            n272 = Array Subset(array=w475, index=w474, length=w474) -> (w473:dbl[])
            n273 = call <vilib>:"DAQmx Write (Analog 1D DBL NChan 1Samp).vi"("task/channels in"=w501, "data"=w473, "timeout"=100.0, "error in"=w490) -> ("task out"=w502:refnum<k21>, "error out"=→"error out (KIKUSI CTRL)":errorcluster)  [unwired: 9 in, 1 out]
            n274 = local write "AO task out"(w502) -> ()
            n275 = Build Array (concatenate)(w486, w476) -> (w485:dbl[])
          }
        }
        n276 = local read "All Labels (USB6218)"() -> (w443:string[])
        n277 = local read "DataArrayConv (USB6218)"() -> (w442:dbl[][])
        n278 = local read "Last Data \n(USB6218)"() -> (w439:dbl[])
        n279 = local read "TimeArray (USB6218)"() -> (w440:timestamp[])
        n280 = Search 1D Array(1D array=w443, element="I_CV") -> (index of element=w444:i32)  [unwired: 1 in]
        n281 = Index Array(array=w442, index (row)=w444) -> (element=w441:dbl[])  [unwired: 1 in]
        n282 = Index Array(array=w439, index=w444) -> (element=w436:dbl)
        n283 = Bundle("TimeArray (USB6218)"=w440, "DataArrayConv (USB6218)"=w441) -> (w437:T18)  [unwired: 1 in]
        n284 = xnode "Formula"("X1"=w436) -> ("Result"=→"Monitor Current (mA)":dbl)  [unwired: 1 in, 1 out]
      }
      event "upper limit (mA)\n (Kikusui)", "upper limit (V)\n (Kikusui)", "lower limit (mA) \n(Kikusui)", "lower limit (V) \n(Kikusui)": Value Change {
        n285 = event-data() -> ()  [unwired: 1 in, 6 out]
        n286 = property on="Set Current (mA)\n (Kikusui)" class="DigNum (strict)"("Maximum"="upper limit (mA)\n (Kikusui)", "Minimum"="lower limit (mA) \n(Kikusui)") -> ()  [unwired: 2 in, 2 out]
        n287 = property on="Set Voltage (V)\n (Kikusui)" class="DigNum (strict)"("Maximum"="upper limit (V)\n (Kikusui)", "Minimum"="lower limit (V) \n(Kikusui)") -> ()  [unwired: 2 in, 2 out]
      }
      event "OUTPUT\n(Kikusui)": Value Change {
        n288 = event-data() -> ()  [unwired: 1 in, 6 out]
        n289 = local read "Cycle #"() -> (w532:u32)
        n290 = Greater?(x=w532, y=u32 0) -> (0:w530:bool)
        n291 = case shown="True" w530 {
          tunnel: w529 -> [_ w536]
          frame False {
          }
          frame True {
            n292 = property on="V1 (N.O.)" class="Bool (strict)"() -> ("Value"=w547:bool)  [unwired: 2 in, 2 out]
            n293 = Not(x=w547) -> (.not. x?=w546:bool)
            n294 = local read "error out (USB6210/6218 DOUT)"() -> (w550:errorcluster)
            n295 = property on="V2 (N.C.)" class="Bool (strict)"() -> ("Value"=w545:bool)  [unwired: 2 in, 2 out]
            n296 = local read "DOUT task out"() -> (w551:refnum<k21>)
            n297 = Build Array(w546, w545, "OUTPUT\n(Kikusui)") -> (w534:bool[])
            n298 = local read "File Refn USB DO"() -> (w537:refnum<file>)
            n299 = Boolean To (0,1)(Boolean=w534) -> (0, 1=w533:i16[])
            n300 = Initialize Array("%d" ("element"), 3 ("dimension size")) -> (w539:string[])
            n301 = call <vilib>:"DAQmx Write (Digital 1D Bool NChan 1Samp 1Line).vi"("task/channels in"=w551, "data"=w534, "timeout"=10.0, "error in"=w550) -> ("task out"=w548:refnum<k21>, "error out"=w541:errorcluster)  [unwired: 9 in, 1 out]
            n302 = local write "DOUT task out"(w548) -> ()
            n303 = Get Date/Time In Seconds() -> (seconds since 1Jan1904=w538:timestamp)
            n304 = call "FileWrite.vi"("DataArray"=w533, "Time Stamp"=w538, "Error In"=w541, "FileFormat"=w539, "Index"=w536, "refnum in"=w537) -> ("Error Out"=w540:errorcluster, "Byte Stream File Refnum"=w535:refnum<file>)  [unwired: 4 in]
            n305 = local write "File Refn USB DO"(w535) -> ()
            n306 = local write "error out (USB6210/6218 DOUT)"(w540) -> ()
          }
        }
      }
    }
    n307 = Bundle(w368, w365) -> (w367:cluster{timestamp[], dbl[]})  [unwired: 1 in]
    n308 = Build Array(w367, w364) -> (→"Graph 7":T9)
  }
  n309 = while {
    stop <- w560 stop-if-true
    n310 = Get Date/Time In Seconds() -> (seconds since 1Jan1904=w559:timestamp)
    n311 = Format Date/Time String(time format string (%c)="%Y%m", seconds (now)=w559) -> (date/time string=w556:string)  [unwired: 1 in]
    n312 = Build Path(base path="Base Path (screenshots)", name or relative path=w556) -> (appended path=w555:path)
    n313 = Create Folder(path (use dialog)=w555, error in=errorcluster {"status"=FALSE, "code"=0, "source"=""}) -> (created path=w552:path, error out=→"error out (monthly folder creation)":errorcluster)  [unwired: 1 in, 1 out]
    n314 = event shown="[1] \"Frontpanel screenshots\": Value Change" {
      selector: _ -> [_ _ _]
      dyn-events: _ -> [_ _ _]
      timeout: _ -> [_ _ _]
      tunnel: [FALSE _ TRUE] -> w560
      tunnel: w552 -> [_ w568 _]
      tunnel: w559 -> [_ w567 _]
      event Timeout {
        n315 = event-data() -> ()  [unwired: 1 in, 3 out]
      }
      event "Frontpanel screenshots": Value Change {
        n316 = event-data() -> ()  [unwired: 1 in, 3 out]
        n317 = property class="TabCtl (strict)"() -> ("Value"=w565:T2)  [unwired: 2 in, 2 out]
        n318 = stacked-sequence {
          tunnel: w568 -> [w574 w596 w618 w640 w662 w684 w706 w728 _]
          tunnel: w567 -> [w573 w595 w617 w639 w661 w683 w705 w727 _]
          tunnel: [w571 _ _ _ _ _ _ _ _] -> w566
          tunnel: w565 -> [w570 _ _ _ _ _ _ _ _]
          tunnel: [w570 _ _ _ _ _ _ _ _] -> w564
          tunnel: "cryostatus_" ("string") -> [w569 w592 w614 w636 w658 w680 w702 w724 _]
          frame #0 {
            n319 = flat-sequence {
              tunnel: w573 -> [w576]
              tunnel: [w576] -> w572
              tunnel: w574 -> [w591]
              tunnel: w572 -> [w579]
              tunnel: [w578] -> w571
              tunnel: w569 -> [w577]
              frame #0 {
                n320 = property class="TabCtl (strict)"("Val(Sgnl)"=T2."NI USB CONFIG" ("Value (Signaling)")) -> ()  [unwired: 2 in, 2 out]
              }
              frame #1 {
                w589 = "_" ("string")
                n321 = local read "Cycle #"() -> (w587:u32)
                n322 = call "LV_UNIXTIME.vi"("current time"=w579) -> ("date/time string"=w590:string)  [unwired: 9 in, 1 out]
                n323 = Format Value(format string="%06d", value (0)=w587) -> (output string=w586:string)  [unwired: 1 in]
                n324 = Concatenate Strings(w577, w590, w589, w586, w589, "page1.png" ("string")) -> (w584:string)
                n325 = invoke class="TabCtl (strict)" method="Get Image"(error in=errorcluster {"status"=FALSE, "code"=0, "source"=""} ("error in (no error)")) -> (error out=w580:errorcluster, "image data"=w582:T14)  [unwired: 5 in, 4 out]
                n326 = Build Path(base path=w591, name or relative path=w584) -> (appended path=w583:path)
                n327 = call <vilib>:"Write PNG File.vi"("error in (no error)"=w580, "image data"=w582, "path to PNG file"=w583) -> ("error out"=w578:errorcluster)  [unwired: 7 in, 1 out]
              }
            }
          }
          frame #1 {
            n328 = flat-sequence {
              tunnel: w595 -> [w598]
              tunnel: [w598] -> w594
              tunnel: w596 -> [w613]
              tunnel: w594 -> [w601]
              tunnel: [w600] -> w593
              tunnel: w592 -> [w599]
              frame #0 {
                n329 = property class="TabCtl (strict)"("Val(Sgnl)"=T2."LSI CONFIG" ("Value (Signaling)")) -> ()  [unwired: 2 in, 2 out]
              }
              frame #1 {
                w611 = "_" ("string")
                n330 = local read "Cycle #"() -> (w609:u32)
                n331 = call "LV_UNIXTIME.vi"("current time"=w601) -> ("date/time string"=w612:string)  [unwired: 9 in, 1 out]
                n332 = Format Value(format string="%06d", value (0)=w609) -> (output string=w608:string)  [unwired: 1 in]
                n333 = Concatenate Strings(w599, w612, w611, w608, w611, "page2.png" ("string")) -> (w606:string)
                n334 = invoke class="TabCtl (strict)" method="Get Image"(error in=errorcluster {"status"=FALSE, "code"=0, "source"=""} ("error in (no error)")) -> (error out=w602:errorcluster, "image data"=w604:T14)  [unwired: 5 in, 4 out]
                n335 = Build Path(base path=w613, name or relative path=w606) -> (appended path=w605:path)
                n336 = call <vilib>:"Write PNG File.vi"("error in (no error)"=w602, "image data"=w604, "path to PNG file"=w605) -> ("error out"=w600:errorcluster)  [unwired: 7 in, 1 out]
              }
            }
            n337 = local write "error out (frontpanel screenshots)"(w593) -> ()
          }
          frame #2 {
            n338 = flat-sequence {
              tunnel: w617 -> [w620]
              tunnel: [w620] -> w616
              tunnel: w618 -> [w635]
              tunnel: w616 -> [w623]
              tunnel: [w622] -> w615
              tunnel: w614 -> [w621]
              frame #0 {
                n339 = property class="TabCtl (strict)"("Val(Sgnl)"=T2."MEASUREMENT" ("Value (Signaling)")) -> ()  [unwired: 2 in, 2 out]
              }
              frame #1 {
                w633 = "_" ("string")
                n340 = local read "Cycle #"() -> (w631:u32)
                n341 = Format Value(format string="%06d", value (0)=w631) -> (output string=w630:string)  [unwired: 1 in]
                n342 = call "LV_UNIXTIME.vi"("current time"=w623) -> ("date/time string"=w634:string)  [unwired: 9 in, 1 out]
                n343 = Concatenate Strings(w621, w634, w633, w630, w633, "page3.png" ("string")) -> (w628:string)
                n344 = invoke class="TabCtl (strict)" method="Get Image"(error in=errorcluster {"status"=FALSE, "code"=0, "source"=""} ("error in (no error)")) -> (error out=w624:errorcluster, "image data"=w626:T14)  [unwired: 5 in, 4 out]
                n345 = Build Path(base path=w635, name or relative path=w628) -> (appended path=w627:path)
                n346 = call <vilib>:"Write PNG File.vi"("error in (no error)"=w624, "image data"=w626, "path to PNG file"=w627) -> ("error out"=w622:errorcluster)  [unwired: 7 in, 1 out]
              }
            }
            n347 = local write "error out (frontpanel screenshots)"(w615) -> ()
          }
          frame #3 {
            n348 = flat-sequence {
              tunnel: w639 -> [w642]
              tunnel: [w642] -> w638
              tunnel: w640 -> [w657]
              tunnel: w638 -> [w645]
              tunnel: [w644] -> w637
              tunnel: w636 -> [w643]
              frame #0 {
                n349 = property class="TabCtl (strict)"("Val(Sgnl)"=T2."HE AUTO FILL" ("Value (Signaling)")) -> ()  [unwired: 2 in, 2 out]
              }
              frame #1 {
                w655 = "_" ("string")
                n350 = local read "Cycle #"() -> (w653:u32)
                n351 = Format Value(format string="%06d", value (0)=w653) -> (output string=w652:string)  [unwired: 1 in]
                n352 = call "LV_UNIXTIME.vi"("current time"=w645) -> ("date/time string"=w656:string)  [unwired: 9 in, 1 out]
                n353 = Concatenate Strings(w643, w656, w655, w652, w655, "page4.png" ("string")) -> (w650:string)
                n354 = invoke class="TabCtl (strict)" method="Get Image"(error in=errorcluster {"status"=FALSE, "code"=0, "source"=""} ("error in (no error)")) -> (error out=w646:errorcluster, "image data"=w648:T14)  [unwired: 5 in, 4 out]
                n355 = Build Path(base path=w657, name or relative path=w650) -> (appended path=w649:path)
                n356 = call <vilib>:"Write PNG File.vi"("error in (no error)"=w646, "image data"=w648, "path to PNG file"=w649) -> ("error out"=w644:errorcluster)  [unwired: 7 in, 1 out]
              }
            }
            n357 = local write "error out (frontpanel screenshots)"(w637) -> ()
          }
          frame #4 {
            n358 = flat-sequence {
              tunnel: w661 -> [w664]
              tunnel: [w664] -> w660
              tunnel: w662 -> [w679]
              tunnel: w660 -> [w667]
              tunnel: [w666] -> w659
              tunnel: w658 -> [w665]
              frame #0 {
                n359 = property class="TabCtl (strict)"("Val(Sgnl)"=T2."VALVE/HEATER CTRL" ("Value (Signaling)")) -> ()  [unwired: 2 in, 2 out]
              }
              frame #1 {
                w677 = "_" ("string")
                n360 = local read "Cycle #"() -> (w675:u32)
                n361 = call "LV_UNIXTIME.vi"("current time"=w667) -> ("date/time string"=w678:string)  [unwired: 9 in, 1 out]
                n362 = Format Value(format string="%06d", value (0)=w675) -> (output string=w674:string)  [unwired: 1 in]
                n363 = Concatenate Strings(w665, w678, w677, w674, w677, "page5.png" ("string")) -> (w672:string)
                n364 = invoke class="TabCtl (strict)" method="Get Image"(error in=errorcluster {"status"=FALSE, "code"=0, "source"=""} ("error in (no error)")) -> (error out=w668:errorcluster, "image data"=w670:T14)  [unwired: 5 in, 4 out]
                n365 = Build Path(base path=w679, name or relative path=w672) -> (appended path=w671:path)
                n366 = call <vilib>:"Write PNG File.vi"("error in (no error)"=w668, "image data"=w670, "path to PNG file"=w671) -> ("error out"=w666:errorcluster)  [unwired: 7 in, 1 out]
              }
            }
            n367 = local write "error out (frontpanel screenshots)"(w659) -> ()
          }
          frame #5 {
            n368 = flat-sequence {
              tunnel: w683 -> [w686]
              tunnel: [w686] -> w682
              tunnel: w684 -> [w701]
              tunnel: w682 -> [w689]
              tunnel: [w688] -> w681
              tunnel: w680 -> [w687]
              frame #0 {
                n369 = property class="TabCtl (strict)"("Val(Sgnl)"=T2."DMMs" ("Value (Signaling)")) -> ()  [unwired: 2 in, 2 out]
              }
              frame #1 {
                w699 = "_" ("string")
                n370 = local read "Cycle #"() -> (w697:u32)
                n371 = call "LV_UNIXTIME.vi"("current time"=w689) -> ("date/time string"=w700:string)  [unwired: 9 in, 1 out]
                n372 = Format Value(format string="%06d", value (0)=w697) -> (output string=w696:string)  [unwired: 1 in]
                n373 = Concatenate Strings(w687, w700, w699, w696, w699, "page6.png" ("string")) -> (w694:string)
                n374 = invoke class="TabCtl (strict)" method="Get Image"(error in=errorcluster {"status"=FALSE, "code"=0, "source"=""} ("error in (no error)")) -> (error out=w690:errorcluster, "image data"=w692:T14)  [unwired: 5 in, 4 out]
                n375 = Build Path(base path=w701, name or relative path=w694) -> (appended path=w693:path)
                n376 = call <vilib>:"Write PNG File.vi"("error in (no error)"=w690, "image data"=w692, "path to PNG file"=w693) -> ("error out"=w688:errorcluster)  [unwired: 7 in, 1 out]
              }
            }
            n377 = local write "error out (frontpanel screenshots)"(w681) -> ()
          }
          frame #6 {
            n378 = flat-sequence {
              tunnel: w705 -> [w708]
              tunnel: [w708] -> w704
              tunnel: w706 -> [w723]
              tunnel: w704 -> [w711]
              tunnel: [w710] -> w703
              tunnel: w702 -> [w709]
              frame #0 {
                n379 = property class="TabCtl (strict)"("Val(Sgnl)"=T2."DIAGRAM" ("Value (Signaling)")) -> ()  [unwired: 2 in, 2 out]
              }
              frame #1 {
                w721 = "_" ("string")
                n380 = local read "Cycle #"() -> (w719:u32)
                n381 = Format Value(format string="%06d", value (0)=w719) -> (output string=w718:string)  [unwired: 1 in]
                n382 = call "LV_UNIXTIME.vi"("current time"=w711) -> ("date/time string"=w722:string)  [unwired: 9 in, 1 out]
                n383 = Concatenate Strings(w709, w722, w721, w718, w721, "page7.png" ("string")) -> (w716:string)
                n384 = invoke class="TabCtl (strict)" method="Get Image"(error in=errorcluster {"status"=FALSE, "code"=0, "source"=""} ("error in (no error)")) -> (error out=w712:errorcluster, "image data"=w714:T14)  [unwired: 5 in, 4 out]
                n385 = Build Path(base path=w723, name or relative path=w716) -> (appended path=w715:path)
                n386 = call <vilib>:"Write PNG File.vi"("error in (no error)"=w712, "image data"=w714, "path to PNG file"=w715) -> ("error out"=w710:errorcluster)  [unwired: 7 in, 1 out]
              }
            }
            n387 = local write "error out (frontpanel screenshots)"(w703) -> ()
          }
          frame #7 {
            n388 = flat-sequence {
              tunnel: w727 -> [w730]
              tunnel: [w730] -> w726
              tunnel: w728 -> [w745]
              tunnel: w726 -> [w733]
              tunnel: [w732] -> w725
              tunnel: w724 -> [w731]
              frame #0 {
                n389 = property class="TabCtl (strict)"("Val(Sgnl)"=T2."(Plc. hld.)" ("Value (Signaling)")) -> ()  [unwired: 2 in, 2 out]
              }
              frame #1 {
                w743 = "_" ("string")
                n390 = local read "Cycle #"() -> (w741:u32)
                n391 = Format Value(format string="%06d", value (0)=w741) -> (output string=w740:string)  [unwired: 1 in]
                n392 = call "LV_UNIXTIME.vi"("current time"=w733) -> ("date/time string"=w744:string)  [unwired: 9 in, 1 out]
                n393 = Concatenate Strings(w731, w744, w743, w740, w743, "page8.png" ("string")) -> (w738:string)
                n394 = invoke class="TabCtl (strict)" method="Get Image"(error in=errorcluster {"status"=FALSE, "code"=0, "source"=""} ("error in (no error)")) -> (error out=w734:errorcluster, "image data"=w736:T14)  [unwired: 5 in, 4 out]
                n395 = Build Path(base path=w745, name or relative path=w738) -> (appended path=w737:path)
                n396 = call <vilib>:"Write PNG File.vi"("error in (no error)"=w734, "image data"=w736, "path to PNG file"=w737) -> ("error out"=w732:errorcluster)  [unwired: 7 in, 1 out]
              }
            }
            n397 = local write "error out (frontpanel screenshots)"(w725) -> ()
          }
          frame #8 {
            n398 = local write "Frontpanel screenshots"(FALSE ("Frontpanel screenshots")) -> ()
          }
        }
        "error out (frontpanel screenshots)" <- w566
        n399 = property class="TabCtl (strict)"("Val(Sgnl)"=w564) -> ()  [unwired: 2 in, 2 out]
      }
      event "Stop Button": Value Change {
        n400 = event-data() -> ()  [unwired: 1 in, 3 out]
      }
    }
    n401 = Wait (ms)(milliseconds to wait=u32 123) -> ()  [unwired: 1 out]
  }
  n402 = while {
    stop <- w748 stop-if-true
    n403 = Wait (ms)(milliseconds to wait=u32 101) -> ()  [unwired: 1 out]
    n404 = event shown="[2] Timeout" {
      selector: _ -> [_ _ _]
      dyn-events: _ -> [_ _ _]
      timeout: _ -> [_ _ _]
      tunnel: [FALSE TRUE FALSE] -> w748
      event "Initialize (DMMs)": Value Change {
        w751 = T1 [] ("Value (Signaling)")
        n405 = event-data() -> ()  [unwired: 1 in, 3 out]
        n406 = property on="Graph DMMs 1" class="XYGraph (strict)"("Val(Sgnl)"=w751) -> ()  [unwired: 2 in, 2 out]
        n407 = property on="Graph DMMs 2" class="XYGraph (strict)"("Val(Sgnl)"=w751) -> ()  [unwired: 2 in, 2 out]
      }
      event "Stop Button": Value Change {
        n408 = event-data() -> ()  [unwired: 1 in, 3 out]
      }
      event Timeout {
        n409 = event-data() -> ()  [unwired: 1 in, 3 out]
      }
    }
  }
  n410 = Obtain Notifier(name (unnamed)="stop notifier", notification data type=w9, create if not found? (T)=w9, error in (no error)=errorcluster {"status"=FALSE, "code"=0, "source"=""}) -> (notifier out=w3:refnum<notifier>, error out=w2:errorcluster)  [unwired: 1 out]
  n411 = while {
    shift-right: [w852] -> w36
    shift-left: refnum<class "USBData.lvclass"> refnum ("USBData.lvclass") -> [w855]
    shift-right: [w848] -> w35
    shift-left: errorcluster {"status"=FALSE, "code"=0, "source"=""} ("error in (no error)") -> [w854]
    tunnel: "RUN label" -> [w760]
    tunnel: "Base Path" -> [w792]
    shift-right: [w830] -> w29
    shift-left: errorcluster {"status"=FALSE, "code"=0, "source"=""} ("error in (no error)") -> [w846]
    shift-right: [w831] -> w30
    shift-left: refnum<class "LSI218Data.lvclass"> refnum ("LSI218Data.lvclass") -> [w845]
    shift-right: [w818] -> w26
    shift-left: refnum<class "LSI336Data.lvclass"> refnum ("LSI336Data.lvclass") -> [w827]
    shift-right: [w817] -> w25
    shift-left: w15 -> [w826]
    shift-right: [w806] -> _
    shift-left: errorcluster {"status"=FALSE, "code"=0, "source"=""} ("error in") -> [w807]
    shift-right: [w796] -> w19
    shift-left: refnum<class "USBData.lvclass"> refnum ("USBData.lvclass") -> [w804]
    shift-right: [w795] -> w18
    shift-left: errorcluster {"status"=FALSE, "code"=0, "source"=""} ("error in (no error)") -> [w803]
    shift-right: [w791] -> _
    shift-left: w15 -> [w790]
    tunnel: w3 -> [w758]
    tunnel: w2 -> [w757]
    tunnel: [w755] -> w5
    tunnel: [w754] -> w4
    i -> [w767]
    stop <- "Stop Button" stop-if-true
    w813 = u32 24 ("Number of Rows")
    w823 = T20 [] ("appended array")
    w840 = T20 [] ("appended array")
    n412 = local read "LSI218Settings(A-F)"() -> (w782:T4)
    n413 = control-ref of="Plot selecter LSI218(2)\n    1      2     3     4"() -> (w811:refnum<vi>)
    n414 = control-ref of="Plot selecter LSI218(1)\n    1      2     3     4"() -> (w812:refnum<vi>)
    n415 = control-ref of="Plot selecter LSI336 \n     1      2     3     4"() -> (w810:refnum<vi>)
    n416 = property on="Property Node" class="Arr (strict)"(reference=w811, "Number of Rows"=w813) -> ()  [unwired: 1 in, 2 out]
    n417 = property on="Property Node" class="Arr (strict)"(reference=w812, "Number of Rows"=w813) -> ()  [unwired: 1 in, 2 out]
    n418 = local read "LSI336Settings(X,Y)"() -> (w780:T4)
    n419 = Array Size(array=w782) -> (size(s)=w781:i32)
    n420 = property on="Property Node" class="Arr (strict)"(reference=w810, "Number of Rows"=u32 8) -> ()  [unwired: 1 in, 2 out]
    n421 = Multiply(x="Measurement Interval (s)", y=u32 1000) -> (x*y=w849:dbl)
    n422 = Wait (ms)(milliseconds to wait=w849) -> ()  [unwired: 1 out]
    n423 = for {
      N: w781 -> [_]
      tunnel: w782 -> [w866] mode=indexing
      tunnel: [w865] -> w778 mode=concatenating
      n424 = Unbundle By Name(w866) -> ("SensorLocations"=w865:T13)
    }
    n425 = for {
      tunnel: w780 -> [w864] mode=indexing
      tunnel: [w863] -> w779 mode=concatenating
      n426 = Unbundle By Name(w864) -> ("SensorLocations"=w863:T13)
    }
    n427 = Quotient & Remainder(x=w767, y="Screenshots interval") -> (x-y*floor(x/y)=w765:i64)  [unwired: 1 out]
    n428 = Equal?(x=w767, y=0) -> (x = y?=w759:bool)
    n429 = case shown="True" w759 {
      tunnel: w855 -> [w1904 w1927]
      tunnel: w854 -> [w1898 w1925]
      tunnel: w767 -> [w1889 _]
      tunnel: [w1896 w1922] -> w848
      tunnel: [w1893 w1921] -> w805
      tunnel: [w1894 w1920] -> w852
      tunnel: [w1884 w1915] -> w853
      tunnel: w792 -> [_ w1914]
      tunnel: [w1883 w1911] -> w787
      frame False {
        n430 = call-dynamic "USBData_measure.vi"("USBData in"=w1904, "DAQ sample #"=i64 5, "DAQ timeout"=100.0 ("DAQ timeout (def: 100)"), "MeasurementIndex"=w1889, "error in (no error)"=w1898, "save every ... measurements"="Record interval") -> ("USBData out"=w1903:refnum<class "USBData.lvclass">, "TimeMeasuremeent"=w1900:timestamp, "Status"=→"USB6210 Status":T6, "LastDataAcquired"=w1885:dbl[], "error out"=w1899:errorcluster)  [unwired: 3 in, 2 out]
        "Time of Last Measurement (USB6210)" <- w1900
        "Last Vol\n(USB6210)" <- w1885
        n431 = call-dynamic "USBData_convert.vi"("Save every ... measurements"="Record interval", "MeasurementIndex"=w1889, "error in (no error)"=w1899, "LastDataAcquired"=w1885, "TimeMeasuremeent"=w1900, "USBData in"=w1903) -> ("error out"=w1897:errorcluster, "LeakDet_FULL"=w1892:dbl, "LastDataConverted"=w1886:dbl[], "USBData out"=w1895:refnum<class "USBData.lvclass">)  [unwired: 2 in]
        n432 = call "USBData_read.vi"("USBData in"=w1895, "error in (no error)"=w1897) -> ("Status"=w1887:T6, "USBData out"=w1894:refnum<class "USBData.lvclass">, "Data"=w1893:T21, "Basic"=w1884:T22, "error out"=w1896:errorcluster)  [unwired: 2 in, 2 out]
        n433 = local write "USB6210 Status"(w1887) -> ()
        n434 = Unbundle By Name(w1884) -> ("ReadLeakDet?"=w1891:bool)
        n435 = Unbundle By Name(w1884) -> ("Labels"=w1883:string[])
        n436 = case shown="False" w1891 {
          tunnel: w1886 -> [w1905 w1908]
          tunnel: w1892 -> [_ w1907]
          tunnel: [w1905 w1906] -> w1890
          frame False {
          }
          frame True {
            n437 = Build Array (concatenate)(w1908, w1907) -> (w1906:dbl[])
          }
        }
        "Last Data \n(USB6210)" <- w1890
      }
      frame True {
        n438 = local read "RUN Identifier"() -> (w1909:string)
        n439 = call-dynamic "USBData_initialize.vi"("USBData in"=w1927, "SeriesSetting"="USB6210 Config", "BasePath"=w1914, "RunIdentifier"=w1909, "FileName"="InstName (USB6210)", "error in (no error)"=w1925) -> ("Status"=w1910:T6, "USBData out"=w1923:refnum<class "USBData.lvclass">, "error out"=w1924:errorcluster)  [unwired: 5 in, 2 out]
        n440 = local write "USB6210 Status"(w1910) -> ()
        n441 = call "USBData_read.vi"("USBData in"=w1923, "error in (no error)"=w1924) -> ("Status"=w1913:T6, "USBData out"=w1920:refnum<class "USBData.lvclass">, "Data"=w1921:T21, "Basic"=w1915:T22, "error out"=w1922:errorcluster)  [unwired: 2 in, 2 out]
        n442 = local write "USB6210 Status"(w1913) -> ()
        n443 = Unbundle By Name(w1915) -> ("ReadLeakDet?"=w1919:bool, "Labels"=w1911:string[])
        n444 = Array Size(array=w1911) -> (size(s)=w1918:i32)
        n445 = case shown="True" w1919 {
          tunnel: w1918 -> [w1928 w1930]
          tunnel: [w1928 w1929] -> w1916
          frame False {
          }
          frame True {
            n446 = Add(x=w1930, y=1) -> (x+y=w1929:i32)
          }
        }
        n447 = Initialize Array(TRUE ("Activate 2"), w1916) -> ()  [unwired: 1 out]
      }
    }
    "error out (USB6210)" <- w848
    n448 = case shown="False" w759 {
      tunnel: [w1437 w1464] -> w795
      tunnel: [w1434 w1463] -> w802
      tunnel: [w1435 w1462] -> w796
      tunnel: [w1426 w1457] -> w801
      tunnel: [w1425 w1455] -> _
      tunnel: w804 -> [w1424 w1453]
      tunnel: w792 -> [_ w1452]
      tunnel: w803 -> [w1423 w1451]
      tunnel: w767 -> [w1422 _]
      frame False {
        n449 = local read "Record interval"() -> (w1421:i64)
        n450 = call-dynamic "USBData_measure.vi"("USBData in"=w1424, "DAQ sample #"=i64 5, "DAQ timeout"=100.0 ("DAQ timeout (def: 100)"), "MeasurementIndex"=w1422, "error in (no error)"=w1423, "save every ... measurements"=w1421) -> ("USBData out"=w1443:refnum<class "USBData.lvclass">, "TimeMeasuremeent"=w1440:timestamp, "Status"=→"USB6218 Status":T6, "LastDataAcquired"=w1427:dbl[], "error out"=w1439:errorcluster)  [unwired: 3 in, 2 out]
        "Time of Last Measurement (USB6218)" <- w1440
        "Last Vol \n(USB6218)" <- w1427
        n451 = call-dynamic "USBData_convert.vi"("Save every ... measurements"=w1421, "MeasurementIndex"=w1422, "error in (no error)"=w1439, "LastDataAcquired"=w1427, "TimeMeasuremeent"=w1440, "USBData in"=w1443) -> ("error out"=w1438:errorcluster, "LeakDet_FULL"=w1433:dbl, "LastDataConverted"=w1428:dbl[], "USBData out"=w1436:refnum<class "USBData.lvclass">)  [unwired: 2 in]
        n452 = call "USBData_read.vi"("USBData in"=w1436, "error in (no error)"=w1438) -> ("Status"=w1429:T6, "USBData out"=w1435:refnum<class "USBData.lvclass">, "Data"=w1434:T21, "Basic"=w1426:T22, "error out"=w1437:errorcluster)  [unwired: 2 in, 2 out]
        n453 = local write "USB6218 Status"(w1429) -> ()
        n454 = Unbundle By Name(w1426) -> ("ReadLeakDet?"=w1432:bool)
        n455 = Unbundle By Name(w1426) -> ("Labels"=w1425:string[])
        n456 = case shown="True" w1432 {
          tunnel: w1428 -> [w1444 w1447]
          tunnel: w1433 -> [_ w1446]
          tunnel: [w1444 w1445] -> w1431
          frame False {
          }
          frame True {
            n457 = Build Array (concatenate)(w1447, w1446) -> (w1445:dbl[])
          }
        }
        "Last Data \n(USB6218)" <- w1431
      }
      frame True {
        n458 = local read "RUN Identifier"() -> (w1448:string)
        n459 = call-dynamic "USBData_initialize.vi"("USBData in"=w1453, "SeriesSetting"="USB6218 Config", "BasePath"=w1452, "RunIdentifier"=w1448, "FileName"="InstName (USB6218)", "error in (no error)"=w1451) -> ("Status"=w1449:T6, "USBData out"=w1465:refnum<class "USBData.lvclass">, "error out"=w1466:errorcluster)  [unwired: 5 in, 2 out]
        n460 = local write "USB6218 Status"(w1449) -> ()
        n461 = call "USBData_read.vi"("USBData in"=w1465, "error in (no error)"=w1466) -> ("Status"=w1456:T6, "USBData out"=w1462:refnum<class "USBData.lvclass">, "Data"=w1463:T21, "Basic"=w1457:T22, "error out"=w1464:errorcluster)  [unwired: 2 in, 2 out]
        n462 = local write "USB6218 Status"(w1456) -> ()
        n463 = Unbundle By Name(w1457) -> ("ReadLeakDet?"=w1461:bool, "Labels"=w1455:string[])
        n464 = Array Size(array=w1455) -> (size(s)=w1460:i32)
        n465 = case shown="True" w1461 {
          tunnel: w1460 -> [w1467 w1469]
          tunnel: [w1467 w1468] -> w1458
          frame False {
          }
          frame True {
            n466 = Add(x=w1469, y=1) -> (x+y=w1468:i32)
          }
        }
        n467 = Initialize Array(TRUE ("Activate 2"), w1458) -> ()  [unwired: 1 out]
      }
    }
    "error out (USB6218)" <- w795
    n468 = case shown="True" w759 {
      tunnel: w760 -> [_ w858]
      frame False {
      }
      frame True {
        n469 = Get Date/Time In Seconds() -> (seconds since 1Jan1904=w861:timestamp)
        n470 = call "LV_UNIXTIME.vi"("current time"=w861) -> ("date/time string"=w860:string)  [unwired: 9 in, 1 out]
        n471 = Concatenate Strings(w860, "_" ("string"), w858) -> (→"RUN Identifier" →"RUN Identifier 2" →"RUN Identifier 3" →"RUN Identifier 4" →"RUN Identifier 5" →"RUN Identifier 6" →"RUN Identifier 7":string)
      }
    }
    n472 = Equal?(x=w765, y=i64 0) -> (x = y?=w762:bool)
    n473 = local read "LastData (LSI218)"() -> (w776:dbl[])
    n474 = local read "Last Data \nLSI336"() -> (w775:dbl[])
    n475 = And(x="Analog Out ON?", y=w759) -> (x .and. y?=w793:bool)
    n476 = case shown="True" w793 {
      tunnel: w792 -> [_ w1238]
      tunnel: [w1221 w1229] -> w791
      tunnel: w790 -> [w1221 w1228]
      frame False {
      }
      frame True {
        w1224 = "_raw" ("string")
        w1245 = 10.0 ("V_lim_max")
        w1244 = 0.0 ("V_lim_min")
        w1243 = -1 items=["Default"=-1, "RSE"=10083, "Differential"=10106, "Pseudodifferential"=12529] ("output terminal configuration")
        w1242 = 10348 items=["Volts"=10348, "From Custom Scale"=10065] ("units")
        n477 = local read "RUN Identifier"() -> (w1222:string)
        n478 = Concatenate Strings(w1222, "_AO" ("string")) -> (w1247:string)
        n479 = Concatenate Strings(w1222, "_", "USB_AOUT.csv" ("string")) -> (w1239:string)
        n480 = Build Path(base path=w1238, name or relative path=w1239) -> (appended path=w1235:path)
        n481 = Concatenate Strings("AOUT 0 Label", w1224) -> (w1226:string)
        n482 = Concatenate Strings("AOUT 1 Label", w1224) -> (w1223:string)
        n483 = Open/Create/Replace File(file path (use dialog)=w1235, operation (0:open)=T19."open or create") -> (refnum out=w1233:refnum<file>)  [unwired: 4 in, 2 out]
        n484 = Build Array("AOUT 0 Label", "AOUT 1 Label", w1226, w1223) -> (w1231:string[])
        n485 = call "FileIntialize.vi"("Error In"=w1228, "Labels"=w1231, "refnum in"=w1233) -> ("Error Out"=w1230:errorcluster, "File Refnum"=→"File Refn USB AO":refnum<file>)  [unwired: 7 in]
        n486 = call <vilib>:"DAQmx Create Task.vi"("new task name"=w1247, "auto cleanup"=FALSE, "error in"=w1230) -> ("task out"=w1246:refnum<k21>, "error out"=w1248:errorcluster)  [unwired: 11 in]
        n487 = call-poly <vilib>:"DAQmx Create Virtual Channel.vi"("task in"=w1246, "maximum value"=w1245, "minimum value"=w1244, "output terminal configuration"=w1243, "physical channels"="AOUT For Voltage CTRL", "units"=w1242, "error in"=w1248) -> ("task out"=w1250:refnum<k21>, "error out"=w1251:errorcluster)  [unwired: 7 in]
        n488 = call-poly <vilib>:"DAQmx Create Virtual Channel.vi"("task in"=w1250, "maximum value"=w1245, "minimum value"=w1244, "physical channels"="AOUT for Current CTRL", "error in"=w1251) -> ("task out"=w1253:refnum<k21>, "error out"=w1252:errorcluster)  [unwired: 9 in]
        n489 = call <vilib>:"DAQmx Start Task.vi"("task/channels in"=w1253, "error in"=w1252) -> ("task out"=→"AO task out":refnum<k21>, "error out"=w1229:errorcluster)  [unwired: 12 in]
      }
    }
    "error out (USB6210/6218 AOUT)" <- w791
    n490 = And(x=w762, y="Automatic \nScreenshots?") -> (x .and. y?=w761:bool)
    n491 = Build Array (concatenate)(w776, w775) -> (w774:dbl[])
    "AllTemperatures" <- w774
    n492 = Build Array (concatenate)(w778, w779) -> (w777:T13)
    "TempSensorsLocations" <- w777
    n493 = case shown="True" w761 {
      frame False {
      }
      frame True {
        n494 = flat-sequence {
          frame #0 {
            n495 = property on="Frontpanel screenshots" class="Bool (strict)"("Val(Sgnl)"=TRUE ("Value (Signaling)")) -> ()  [unwired: 2 in, 2 out]
          }
        }
      }
    }
    n496 = flat-sequence {
      tunnel: w774 -> [w867]
      tunnel: w777 -> [w868]
      tunnel: w769 -> [w1120]
      tunnel: w768 -> [w1119]
      frame #0 {
        n497 = stacked-sequence {
          tunnel: w868 -> [w873 w878 w883 w888 w893 w898 w903 w908 w913 w918 w923 w928 w933 w938 w943 w948 w953 w958 w963 w968 w973 w978 w983 w988 w993 w998 w1003 w1008 w1013 w1018 w1023 w1028 w1033 w1038 w1043 w1048 w1053 w1058 w1063 w1068 w1073 w1078 w1083 w1088 w1093 w1098 w1103 w1108 w1113 w1118]
          tunnel: w867 -> [w871 w876 w881 w886 w891 w896 w901 w906 w911 w916 w921 w926 w931 w936 w941 w946 w951 w956 w961 w966 w971 w976 w981 w986 w991 w996 w1001 w1006 w1011 w1016 w1021 w1026 w1031 w1036 w1041 w1046 w1051 w1056 w1061 w1066 w1071 w1076 w1081 w1086 w1091 w1096 w1101 w1106 w1111 w1116]
          frame #0 {
            n498 = Search 1D Array(1D array=w873, element=T11."T3He1-1" ("SensorLocations")) -> (index of element=w870:i32)  [unwired: 1 in]
            n499 = Index Array(array=w871, index=w870) -> (element=→"T3He1-1":dbl)
          }
          frame #1 {
            n500 = Search 1D Array(1D array=w878, element=T11."T3He1-2" ("SensorLocations")) -> (index of element=w875:i32)  [unwired: 1 in]
            n501 = Index Array(array=w876, index=w875) -> (element=→"T3He1-2":dbl)
          }
          frame #2 {
            n502 = Search 1D Array(1D array=w883, element=T11."T3He1-3" ("SensorLocations")) -> (index of element=w880:i32)  [unwired: 1 in]
            n503 = Index Array(array=w881, index=w880) -> (element=→"T3He1-3":dbl)
          }
          frame #3 {
            n504 = Search 1D Array(1D array=w888, element=T11."T3He1-4" ("SensorLocations")) -> (index of element=w885:i32)  [unwired: 1 in]
            n505 = Index Array(array=w886, index=w885) -> (element=→"T3He1-4":dbl)
          }
          frame #4 {
            n506 = Search 1D Array(1D array=w893, element=T11."T3He2-1" ("SensorLocations")) -> (index of element=w890:i32)  [unwired: 1 in]
            n507 = Index Array(array=w891, index=w890) -> (element=→"T3He2-1":dbl)
          }
          frame #5 {
            n508 = Search 1D Array(1D array=w898, element=T11."T3He2-2" ("SensorLocations")) -> (index of element=w895:i32)  [unwired: 1 in]
            n509 = Index Array(array=w896, index=w895) -> (element=→"T3He2-2":dbl)
          }
          frame #6 {
            n510 = Search 1D Array(1D array=w903, element=T11."T3He3" ("SensorLocations")) -> (index of element=w900:i32)  [unwired: 1 in]
            n511 = Index Array(array=w901, index=w900) -> (element=→"T3He3":dbl)
          }
          frame #7 {
            n512 = Search 1D Array(1D array=w908, element=T11."T3He4" ("SensorLocations")) -> (index of element=w905:i32)  [unwired: 1 in]
            n513 = Index Array(array=w906, index=w905) -> (element=→"T3He4":dbl)
          }
          frame #8 {
            n514 = Search 1D Array(1D array=w913, element=T11."T3He5" ("SensorLocations")) -> (index of element=w910:i32)  [unwired: 1 in]
            n515 = Index Array(array=w911, index=w910) -> (element=→"T3He5":dbl)
          }
          frame #9 {
            n516 = Search 1D Array(1D array=w918, element=T11."T3He6-1" ("SensorLocations")) -> (index of element=w915:i32)  [unwired: 1 in]
            n517 = Index Array(array=w916, index=w915) -> (element=→"T3He6-1" →"T3He6-1/6-2 (HEX1)":dbl)
          }
          frame #10 {
            n518 = Search 1D Array(1D array=w923, element=T11."T3He6-2" ("SensorLocations")) -> (index of element=w920:i32)  [unwired: 1 in]
            n519 = Index Array(array=w921, index=w920) -> (element=→"T3He6-2" →"T3He6-1/6-2 (3He pot) 2":dbl)
          }
          frame #11 {
            n520 = Search 1D Array(1D array=w928, element=T11."T3He7-1" ("SensorLocations")) -> (index of element=w925:i32)  [unwired: 1 in]
            n521 = Index Array(array=w926, index=w925) -> (element=→"T3He7-1" →"T3He7-1/7-2 (HEX1)":dbl)
          }
          frame #12 {
            n522 = Search 1D Array(1D array=w933, element=T11."T3He7-2" ("SensorLocations")) -> (index of element=w930:i32)  [unwired: 1 in]
            n523 = Index Array(array=w931, index=w930) -> (element=→"T3He7-2" →"T3He7-1/6-2 (3He pot) 2":dbl)
          }
          frame #13 {
            n524 = Search 1D Array(1D array=w938, element=T11."T3He8" ("SensorLocations")) -> (index of element=w935:i32)  [unwired: 1 in]
            n525 = Index Array(array=w936, index=w935) -> (element=→"T3He8":dbl)
          }
          frame #14 {
            n526 = Search 1D Array(1D array=w943, element=T11."T3He9" ("SensorLocations")) -> (index of element=w940:i32)  [unwired: 1 in]
            n527 = Index Array(array=w941, index=w940) -> (element=→"T3He9":dbl)
          }
          frame #15 {
            n528 = Search 1D Array(1D array=w948, element=T11."T3He10" ("SensorLocations")) -> (index of element=w945:i32)  [unwired: 1 in]
            n529 = Index Array(array=w946, index=w945) -> (element=→"T3He10":dbl)
          }
          frame #16 {
            n530 = Search 1D Array(1D array=w953, element=T11."T4He1" ("SensorLocations")) -> (index of element=w950:i32)  [unwired: 1 in]
            n531 = Index Array(array=w951, index=w950) -> (element=→"T4He1" →"T4He1 (4K reservoir )":dbl)
          }
          frame #17 {
            n532 = Search 1D Array(1D array=w958, element=T11."T4He2-1" ("SensorLocations")) -> (index of element=w955:i32)  [unwired: 1 in]
            n533 = Index Array(array=w956, index=w955) -> (element=→"T4He2-1":dbl)
          }
          frame #18 {
            n534 = Search 1D Array(1D array=w963, element=T11."T4He2-2" ("SensorLocations")) -> (index of element=w960:i32)  [unwired: 1 in]
            n535 = Index Array(array=w961, index=w960) -> (element=→"T4He2-2":dbl)
          }
          frame #19 {
            n536 = Search 1D Array(1D array=w968, element=T11."T4He3-1" ("SensorLocations")) -> (index of element=w965:i32)  [unwired: 1 in]
            n537 = Index Array(array=w966, index=w965) -> (element=→"T4He3-1":dbl)
          }
          frame #20 {
            n538 = Search 1D Array(1D array=w973, element=T11."T4He3-2" ("SensorLocations")) -> (index of element=w970:i32)  [unwired: 1 in]
            n539 = Index Array(array=w971, index=w970) -> (element=→"T4He3-2":dbl)
          }
          frame #21 {
            n540 = Search 1D Array(1D array=w978, element=T11."T4He3-3" ("SensorLocations")) -> (index of element=w975:i32)  [unwired: 1 in]
            n541 = Index Array(array=w976, index=w975) -> (element=→"T4He3-3":dbl)
          }
          frame #22 {
            n542 = Search 1D Array(1D array=w983, element=T11."T4He3-4" ("SensorLocations")) -> (index of element=w980:i32)  [unwired: 1 in]
            n543 = Index Array(array=w981, index=w980) -> (element=→"T4He3-4":dbl)
          }
          frame #23 {
            n544 = Search 1D Array(1D array=w988, element=T11."T4He4" ("SensorLocations")) -> (index of element=w985:i32)  [unwired: 1 in]
            n545 = Index Array(array=w986, index=w985) -> (element=→"T4He4":dbl)
          }
          frame #24 {
            n546 = Search 1D Array(1D array=w993, element=T11."T4He5" ("SensorLocations")) -> (index of element=w990:i32)  [unwired: 1 in]
            n547 = Index Array(array=w991, index=w990) -> (element=→"T4He5":dbl)
          }
          frame #25 {
            n548 = Search 1D Array(1D array=w998, element=T11."T4He6" ("SensorLocations")) -> (index of element=w995:i32)  [unwired: 1 in]
            n549 = Index Array(array=w996, index=w995) -> (element=→"T4He6":dbl)
          }
          frame #26 {
            n550 = Search 1D Array(1D array=w1003, element=T11."T4He7" ("SensorLocations")) -> (index of element=w1000:i32)  [unwired: 1 in]
            n551 = Index Array(array=w1001, index=w1000) -> (element=→"T4He7":dbl)
          }
          frame #27 {
            n552 = Search 1D Array(1D array=w1008, element=T11."T4He8" ("SensorLocations")) -> (index of element=w1005:i32)  [unwired: 1 in]
            n553 = Index Array(array=w1006, index=w1005) -> (element=→"T4He8":dbl)
          }
          frame #28 {
            n554 = Search 1D Array(1D array=w1013, element=T11."T4He9" ("SensorLocations")) -> (index of element=w1010:i32)  [unwired: 1 in]
            n555 = Index Array(array=w1011, index=w1010) -> (element=→"T4He9":dbl)
          }
          frame #29 {
            n556 = Search 1D Array(1D array=w1018, element=T11."T4He10" ("SensorLocations")) -> (index of element=w1015:i32)  [unwired: 1 in]
            n557 = Index Array(array=w1016, index=w1015) -> (element=→"T4He10":dbl)
          }
          frame #30 {
            n558 = Search 1D Array(1D array=w1023, element=T11."T1K1" ("SensorLocations")) -> (index of element=w1020:i32)  [unwired: 1 in]
            n559 = Index Array(array=w1021, index=w1020) -> (element=→"T1K1":dbl)
          }
          frame #31 {
            n560 = Search 1D Array(1D array=w1028, element=T11."T1K2" ("SensorLocations")) -> (index of element=w1025:i32)  [unwired: 1 in]
            n561 = Index Array(array=w1026, index=w1025) -> (element=→"T1K2":dbl)
          }
          frame #32 {
            n562 = Search 1D Array(1D array=w1033, element=T11."T1K3-1" ("SensorLocations")) -> (index of element=w1030:i32)  [unwired: 1 in]
            n563 = Index Array(array=w1031, index=w1030) -> (element=→"T1K3-1" →"T1K3-1/3-2 (1K pot)":dbl)
          }
          frame #33 {
            n564 = Search 1D Array(1D array=w1038, element=T11."T1K3-2" ("SensorLocations")) -> (index of element=w1035:i32)  [unwired: 1 in]
            n565 = Index Array(array=w1036, index=w1035) -> (element=→"T1K3-2" →"T1K3-1/3-2 (1K pot) 2":dbl)
          }
          frame #34 {
            n566 = Search 1D Array(1D array=w1043, element=T11."T1K4" ("SensorLocations")) -> (index of element=w1040:i32)  [unwired: 1 in]
            n567 = Index Array(array=w1041, index=w1040) -> (element=→"T1K4":dbl)
          }
          frame #35 {
            n568 = Search 1D Array(1D array=w1048, element=T11."T1K5" ("SensorLocations")) -> (index of element=w1045:i32)  [unwired: 1 in]
            n569 = Index Array(array=w1046, index=w1045) -> (element=→"T1K5":dbl)
          }
          frame #36 {
            n570 = Search 1D Array(1D array=w1053, element=T11."T1K6" ("SensorLocations")) -> (index of element=w1050:i32)  [unwired: 1 in]
            n571 = Index Array(array=w1051, index=w1050) -> (element=→"T1K6":dbl)
          }
          frame #37 {
            n572 = Search 1D Array(1D array=w1058, element=T11."TIP1" ("SensorLocations")) -> (index of element=w1055:i32)  [unwired: 1 in]
            n573 = Index Array(array=w1056, index=w1055) -> (element=→"TIP1":dbl)
          }
          frame #38 {
            n574 = Search 1D Array(1D array=w1063, element=T11."TIP2" ("SensorLocations")) -> (index of element=w1060:i32)  [unwired: 1 in]
            n575 = Index Array(array=w1061, index=w1060) -> (element=→"TIP2":dbl)
          }
          frame #39 {
            n576 = Search 1D Array(1D array=w1068, element=T11."TIP3" ("SensorLocations")) -> (index of element=w1065:i32)  [unwired: 1 in]
            n577 = Index Array(array=w1066, index=w1065) -> (element=→"TIP3":dbl)
          }
          frame #40 {
            n578 = Search 1D Array(1D array=w1073, element=T11."TIP4" ("SensorLocations")) -> (index of element=w1070:i32)  [unwired: 1 in]
            n579 = Index Array(array=w1071, index=w1070) -> (element=→"TIP4":dbl)
          }
          frame #41 {
            n580 = Search 1D Array(1D array=w1078, element=T11."TIP5" ("SensorLocations")) -> (index of element=w1075:i32)  [unwired: 1 in]
            n581 = Index Array(array=w1076, index=w1075) -> (element=→"TIP5":dbl)
          }
          frame #42 {
            n582 = Search 1D Array(1D array=w1083, element=T11."TIP6" ("SensorLocations")) -> (index of element=w1080:i32)  [unwired: 1 in]
            n583 = Index Array(array=w1081, index=w1080) -> (element=→"TIP6":dbl)
          }
          frame #43 {
            n584 = Search 1D Array(1D array=w1088, element=T11."TIP7" ("SensorLocations")) -> (index of element=w1085:i32)  [unwired: 1 in]
            n585 = Index Array(array=w1086, index=w1085) -> (element=→"TIP7":dbl)
          }
          frame #44 {
            n586 = Search 1D Array(1D array=w1093, element=T11."TTH1" ("SensorLocations")) -> (index of element=w1090:i32)  [unwired: 1 in]
            n587 = Index Array(array=w1091, index=w1090) -> (element=→"TTH1":dbl)
          }
          frame #45 {
            n588 = Search 1D Array(1D array=w1098, element=T11."TTH2" ("SensorLocations")) -> (index of element=w1095:i32)  [unwired: 1 in]
            n589 = Index Array(array=w1096, index=w1095) -> (element=→"TTH2":dbl)
          }
          frame #46 {
            n590 = Search 1D Array(1D array=w1103, element=T11."TTH3" ("SensorLocations")) -> (index of element=w1100:i32)  [unwired: 1 in]
            n591 = Index Array(array=w1101, index=w1100) -> (element=→"TTH3":dbl)
          }
          frame #47 {
            n592 = Search 1D Array(1D array=w1108, element=T11."TTH4" ("SensorLocations")) -> (index of element=w1105:i32)  [unwired: 1 in]
            n593 = Index Array(array=w1106, index=w1105) -> (element=→"TTH4":dbl)
          }
          frame #48 {
            n594 = Search 1D Array(1D array=w1113, element="SensorLocation 1") -> (index of element=w1110:i32)  [unwired: 1 in]
            n595 = Index Array(array=w1111, index=w1110) -> (element=→"Temperature 1":dbl)
          }
          frame #49 {
            n596 = Search 1D Array(1D array=w1118, element="SensorLocation 2") -> (index of element=w1115:i32)  [unwired: 1 in]
            n597 = Index Array(array=w1116, index=w1115) -> (element=→"Temperature 2":dbl)
          }
        }
      }
      frame #1 {
        n598 = stacked-sequence {
          tunnel: w1120 -> [w1125 w1130 w1135 w1140 w1145 w1150 w1155 w1160 w1165 w1170 w1175 w1180 w1185 w1190 w1195 w1200 w1205 w1210 w1215 w1220]
          tunnel: w1119 -> [w1122 w1128 w1134 w1139 w1144 w1148 w1153 w1158 w1163 w1168 w1173 w1178 w1183 w1187 w1192 w1197 w1202 w1207 w1212 w1217]
          frame #0 {
            n599 = Search 1D Array(1D array=w1125, element="Insulation vacuum") -> (index of element=w1123:i32)  [unwired: 1 in]
            n600 = Index Array(array=w1122, index=w1123) -> (element=→"P_ins" →"P (insulation)":dbl)
          }
          frame #1 {
            n601 = Search 1D Array(1D array=w1130, element="4K reservoir pressure") -> (index of element=w1127:i32)  [unwired: 1 in]
            n602 = Index Array(array=w1128, index=w1127) -> (element=→"P_4Kres" →"P (4K reservoir)":dbl)
          }
          frame #2 {
            n603 = Search 1D Array(1D array=w1135, element="3He inlet pressure") -> (index of element=w1133:i32)  [unwired: 1 in]
            n604 = Index Array(array=w1134, index=w1133) -> (element=→"P_3HeIN" →"P (3He IN)":dbl)
          }
          frame #3 {
            n605 = Search 1D Array(1D array=w1140, element="Shield return press.") -> (index of element=w1138:i32)  [unwired: 1 in]
            n606 = Index Array(array=w1139, index=w1138) -> (element=→"P_SldRTN" →"P (shield return)":dbl)
          }
          frame #4 {
            n607 = Search 1D Array(1D array=w1145, element="3He pot pressure") -> (index of element=w1143:i32)  [unwired: 1 in]
            n608 = Index Array(array=w1144, index=w1143) -> (element=→"P_3Hepot" →"P (3He pot)":dbl)
          }
          frame #5 {
            n609 = Search 1D Array(1D array=w1150, element="1Kpot pressure") -> (index of element=w1147:i32)  [unwired: 1 in]
            n610 = Index Array(array=w1148, index=w1147) -> (element=→"P_1Kpot" →"P (1K pot)":dbl)
          }
          frame #6 {
            n611 = Search 1D Array(1D array=w1155, element="Dewar pressure") -> (index of element=w1152:i32)  [unwired: 1 in]
            n612 = Index Array(array=w1153, index=w1152) -> (element=→"P_Dewar" →"P (Dewar)":dbl)
          }
          frame #7 {
            n613 = Search 1D Array(1D array=w1160, element="HEX7 out pressure") -> (index of element=w1157:i32)  [unwired: 1 in]
            n614 = Index Array(array=w1158, index=w1157) -> (element=→"P_HEX7OUT" →"P (HEX7 out)":dbl)
          }
          frame #8 {
            n615 = Search 1D Array(1D array=w1165, element="IPHe pressure") -> (index of element=w1162:i32)  [unwired: 1 in]
            n616 = Index Array(array=w1163, index=w1162) -> (element=→"P_IPHe" →"P (IPHe)":dbl)
          }
          frame #9 {
            n617 = Search 1D Array(1D array=w1170, element="Diff pressure HEX4") -> (index of element=w1167:i32)  [unwired: 1 in]
            n618 = Index Array(array=w1168, index=w1167) -> (element=→"DP_HEX4" →"DP HEX4":dbl)
          }
          frame #10 {
            n619 = Search 1D Array(1D array=w1175, element="Diff pressure HEX5") -> (index of element=w1172:i32)  [unwired: 1 in]
            n620 = Index Array(array=w1173, index=w1172) -> (element=→"DP_HEX5" →"DP HEX5":dbl)
          }
          frame #11 {
            n621 = Search 1D Array(1D array=w1180, element="1K pump exhaust flow") -> (index of element=w1177:i32)  [unwired: 1 in]
            n622 = Index Array(array=w1178, index=w1177) -> (element=→"F_1" →"F1 (1K pump exhaust) flow":dbl)
          }
          frame #12 {
            n623 = Search 1D Array(1D array=w1185, element="Shield flow") -> (index of element=w1182:i32)  [unwired: 1 in]
            n624 = Index Array(array=w1183, index=w1182) -> (element=→"F_2" →"F2 (shield flow)":dbl)
          }
          frame #13 {
            n625 = Search 1D Array(1D array=w1190, element="4He return flow from HEX7") -> (index of element=w1188:i32)  [unwired: 1 in]
            n626 = Index Array(array=w1187, index=w1188) -> (element=→"F_3" →"F3 (4He rtn flw via HEX7)":dbl)
          }
          frame #14 {
            n627 = Search 1D Array(1D array=w1195, element="3He incoming flow into HEX7") -> (index of element=w1193:i32)  [unwired: 1 in]
            n628 = Index Array(array=w1192, index=w1193) -> (element=→"F_4" →"F4 (3He in to HEX7)":dbl)
          }
          frame #15 {
            n629 = Search 1D Array(1D array=w1200, element="3He pump exhaust flow") -> (index of element=w1198:i32)  [unwired: 1 in]
            n630 = Index Array(array=w1197, index=w1198) -> (element=→"F_5" →"F5 (3He pump ex.)":dbl)
          }
          frame #16 {
            n631 = Search 1D Array(1D array=w1205, element="4K reservoir level") -> (index of element=w1203:i32)  [unwired: 1 in]
            n632 = Index Array(array=w1202, index=w1203) -> (element=→"L3" →"He level (4K)":dbl)
          }
          frame #17 {
            n633 = Search 1D Array(1D array=w1210, element="1K pot level") -> (index of element=w1208:i32)  [unwired: 1 in]
            n634 = Index Array(array=w1207, index=w1208) -> (element=→"L(1K) (a1)" →"He level (1K)":dbl)
          }
          frame #18 {
            n635 = Search 1D Array(1D array=w1215, element="1K pot (b)") -> (index of element=w1213:i32)  [unwired: 1 in]
            n636 = Index Array(array=w1212, index=w1213) -> (element=→"1K pot(b1)" →"He level (1K) b":dbl)
          }
          frame #19 {
            n637 = Search 1D Array(1D array=w1220, element="3He pot") -> (index of element=w1218:i32)  [unwired: 1 in]
            n638 = Index Array(array=w1217, index=w1218) -> (element=→"3He pot level" →"He level (3He)":dbl)
          }
        }
      }
    }
    n639 = case shown="True" w759 {
      tunnel: [w1864 w1879] -> w830
      tunnel: [w1859 w1878] -> w847
      tunnel: [w1862 w1877] -> w831
      tunnel: w767 -> [w1863 _]
      tunnel: w846 -> [w1853 w1872]
      tunnel: w845 -> [w1854 w1871]
      tunnel: w792 -> [_ w1870]
      tunnel: [w1851 timestamp[] [] ("TimeArray")] -> w844
      tunnel: [w1850 dbl[][] [] ("DataArray")] -> w843
      frame False {
        w1857 = 24 ("index")
        n640 = local read "Record interval"() -> (w1848:i64)
        n641 = call-dynamic "LSI218Data_measure.vi"("LSI218Data in"=w1854, "MeasurementIndex"=w1863, "error in (no error)"=w1853, "save every ... measurements"=w1848) -> ("TimeMeasuremeent"=→"Time of Last Measurement (LSI218)":timestamp, "Active?"=w1858:bool[], "LSI218Data out"=w1862:refnum<class "LSI218Data.lvclass">, "LastMeasurementConfig"=→"LastMeasurementConfig (218)":T12, "LastData"=w1852:dbl[], "Status"=w1859:u16, "TimeArray"=w1851:timestamp[], "DataArray"=w1850:dbl[][], "error out"=w1864:errorcluster)  [unwired: 3 in]
        "LastData (LSI218)" <- w1852
        n642 = Split 1D Array(array=w1858, index=w1857) -> (first subarray=→"Active?\n (1)":bool[], second subarray=→"Active?\n(2)":bool[])
        n643 = Split 1D Array(array=w1852, index=w1857) -> (first subarray=→"Last Data \nLSI218 (1)":dbl[], second subarray=→"Last Data \nLSI218 (2)":dbl[])
      }
      frame True {
        n644 = local read "RUN Identifier"() -> (w1866:string)
        n645 = call-dynamic "LSI218Data_initialize.vi"("LSI218Settings(A-F)"="LSI218Settings(A-F)", "FileFormat"="FileFormat (218)", "base path"=w1870, "error in (no error)"=w1872, "InstName"="InstName (LSI218)", "RunIdentifier"=w1866, "LSI218Data in"=w1871) -> ("error out"=w1879:errorcluster, "Status"=w1878:T7, "AllLabels"=w1869:string[], "LSI218Data out"=w1877:refnum<class "LSI218Data.lvclass">)  [unwired: 1 in]
        n646 = Split 1D Array(array=w1869, index=24) -> (first subarray=→"Labels LSI218 (1)":string[], second subarray=→"Labels LSI218 (2)":string[])
      }
    }
    "LSI218 Status" <- w847
    "error out (LSI218)" <- w830
    n647 = case shown="True" w759 {
      tunnel: [w1759 w1771] -> w817
      tunnel: [w1749 w1770] -> w825
      tunnel: [w1758 w1769] -> w818
      tunnel: [w1757 timestamp[] [] ("TimeArray")] -> w786
      tunnel: [w1756 dbl[][] [] ("DataArray")] -> w784
      tunnel: w827 -> [w1755 w1766]
      tunnel: w826 -> [w1754 w1765]
      tunnel: w767 -> [w1750 _]
      tunnel: w792 -> [_ w1761]
      frame False {
        n648 = local read "Record interval"() -> (w1747:i64)
        n649 = call-dynamic "LSI336Data_measure.vi"("LSI336Data in"=w1755, "MeasurementIndex"=w1750, "error in (no error)"=w1754, "save every ... measurements"=w1747) -> ("Active?"=→"Active?\n(LSI336)":bool[], "TimeMeasuremeent"=→"Time of Last Measurement (LSI336)":timestamp, "LSI336Data out"=w1758:refnum<class "LSI336Data.lvclass">, "LastData"=→"Last Data \nLSI336":dbl[], "LastMeasurementConfig"=→"LastMeasurementConfig (336)":T12, "DataArray"=w1756:dbl[][], "Status"=w1749:u16, "TimeArray"=w1757:timestamp[], "error out"=w1759:errorcluster)  [unwired: 3 in]
      }
      frame True {
        n650 = local read "RUN Identifier"() -> (w1760:string)
        n651 = call-dynamic "LSI336Data_initialize.vi"("LSI336Data in"=w1766, "RunIdentifier"=w1760, "InstName"="InstName (LSI336)", "FileFormat"="FileFormat (336)", "LSI336Settings(X, Y)"="LSI336Settings(X,Y)", "error in (no error)"=w1765, "base path"=w1761) -> ("LSI336Data out"=w1769:refnum<class "LSI336Data.lvclass">, "Status"=w1770:T7, "AllLabels"=→"Labels LSI336":string[], "error out"=w1771:errorcluster)  [unwired: 5 in]
      }
    }
    "LSI336 Status" <- w825
    "error out (LSI336)" <- w817
    "TimeArray (LSI336)" <- w786
    "DataArray (336)" <- w784
    n652 = local read "Last Data \n(USB6210)"() -> (w770:dbl[])
    n653 = local read "Last Data \n(USB6218)"() -> (w771:dbl[])
    n654 = local read "All Labels (USB6210)"() -> (w773:string[])
    n655 = local read "All Labels (USB6218)"() -> (w772:string[])
    n656 = flat-sequence {
      tunnel: w853 -> [w1355]
      tunnel: [w1350] -> w841
      tunnel: [w1348] -> w839
      tunnel: [w1347] -> w836
      tunnel: [w1346] -> w834
      tunnel: w805 -> [w1341]
      frame #0 {
        w1349 = T20 [] ("appended array")
        n657 = Unbundle By Name(w1341) -> ("TimeArray"=w1358:timestamp[], "DataArrayConv"=w1353:dbl[][], "LDArray"=w1352:dbl[])
        n658 = Unbundle By Name(w1355) -> ("ReadLeakDet?"=w1354:bool, "LabelLD"=w1357:string, "Labels"=w1351:string[])  [unwired: 1 out]
        n659 = case shown="True" w1354 {
          tunnel: w1357 -> [_ w1366]
          tunnel: w1353 -> [w1360 w1365]
          tunnel: w1352 -> [_ w1364]
          tunnel: [w1360 w1363] -> w1340
          tunnel: w1351 -> [w1359 w1362]
          tunnel: [w1359 w1361] -> w1343
          frame False {
          }
          frame True {
            n660 = Build Array (concatenate)(w1365, w1364) -> (w1363:dbl[][])
            n661 = Build Array (concatenate)(w1362, w1366) -> (w1361:string[])
          }
        }
        "All Labels (USB6210)" <- w1343
        "DataArrayConv (USB6210)" <- w1340
        n662 = control-ref of="Plot selecter (USB6210)\n    1      2     3     4"() -> (w1342:refnum<vi>)
        n663 = local read "Plot selecter (USB6210)\n    1      2     3     4"() -> (w1345:bool[][])
        n664 = Array Size(array=w1343) -> (size(s)=w1356:i32)
        n665 = Array Size(array=w1343) -> (size(s)=w1344:i32)
        n666 = Array Size(array=w1340) -> (size(s)=→"Data Array sizes (6210)":i32[])
        n667 = property on="Property Node" class="Arr (strict)"(reference=w1342, "Number of Rows"=w1344) -> ()  [unwired: 1 in, 2 out]
        n668 = for {
          N: w1356 -> [_]
          tunnel: w1340 -> [w1387]
          tunnel: w1358 -> [w1388]
          shift-right: [w1383] -> w1348
          shift-left: w1349 -> [w1386]
          shift-right: [w1381] -> w1346
          shift-left: w1349 -> [w1384]
          shift-right: [w1382] -> w1350
          shift-left: w1349 -> [w1380]
          shift-right: [w1379] -> w1347
          shift-left: w1349 -> [w1378]
          tunnel: w1345 -> [w1377]
          i -> [w1372]
          n669 = Index Array(array=w1387, index (col)=w1372) -> (element=w1367:dbl[])  [unwired: 1 in]
          n670 = Index Array(array=w1377, index (row) #1=w1372, index (col) #1=0 ("index (row)"), index (row) #2=w1372, index (col) #2=1 ("index (row)"), index (row) #3=w1372, index (col) #3=2 ("index (row)"), index (row) #4=w1372, index (col) #4=3 ("index (row)")) -> (element #1=w1371:bool, element #2=w1370:bool, element #3=w1369:bool, element #4=w1368:bool)
          n671 = Bundle("TimeArray"=w1388, "DataArrayConv"=w1367) -> (w1385:T23)  [unwired: 1 in]
          n672 = stacked-sequence {
            tunnel: w1371 -> [w1392 _ _ _]
            tunnel: w1386 -> [_ w1400 _ _]
            tunnel: w1369 -> [_ _ w1408 _]
            tunnel: w1385 -> [w1389 w1398 w1407 w1413]
            tunnel: w1368 -> [_ _ _ w1416]
            tunnel: w1384 -> [_ _ _ w1415]
            tunnel: [_ _ _ w1414] -> w1381
            tunnel: [_ w1399 _ _] -> w1383
            tunnel: [w1391 _ _ _] -> w1382
            tunnel: w1380 -> [w1390 _ _ _]
            tunnel: [_ _ w1406 _] -> w1379
            tunnel: w1378 -> [_ _ w1405 _]
            tunnel: w1370 -> [_ w1397 _ _]
            frame #0 {
              n673 = case shown="True" w1392 {
                tunnel: [w1393 w1396] -> w1391
                tunnel: w1389 -> [_ w1395]
                tunnel: w1390 -> [w1393 w1394]
                frame False {
                }
                frame True {
                  n674 = Build Array (concatenate)(w1394, w1395) -> (w1396:T20)
                }
              }
            }
            frame #1 {
              n675 = case shown="True" w1397 {
                tunnel: w1400 -> [w1401 w1404]
                tunnel: [w1401 w1403] -> w1399
                tunnel: w1398 -> [_ w1402]
                frame False {
                }
                frame True {
                  n676 = Build Array (concatenate)(w1404, w1402) -> (w1403:T20)
                }
              }
            }
            frame #2 {
              n677 = case shown="True" w1408 {
                tunnel: [w1409 w1412] -> w1406
                tunnel: w1407 -> [_ w1411]
                tunnel: w1405 -> [w1409 w1410]
                frame False {
                }
                frame True {
                  n678 = Build Array (concatenate)(w1410, w1411) -> (w1412:T20)
                }
              }
            }
            frame #3 {
              n679 = case shown="True" w1416 {
                tunnel: [w1417 w1420] -> w1414
                tunnel: w1413 -> [_ w1419]
                tunnel: w1415 -> [w1417 w1418]
                frame False {
                }
                frame True {
                  n680 = Build Array (concatenate)(w1418, w1419) -> (w1420:T20)
                }
              }
            }
          }
        }
      }
    }
    n681 = case shown="True" "Digital Out ON?" {
      tunnel: w759 -> [_ w1478]
      tunnel: w807 -> [w1471 w1477]
      tunnel: [w1471 w1476] -> w806
      tunnel: w805 -> [_ w1475]
      tunnel: w760 -> [_ w1474]
      tunnel: w792 -> [_ w1473]
      tunnel: w787 -> [_ w1472]
      frame False {
      }
      frame True {
        n682 = case shown="False" w1478 {
          tunnel: w1477 -> [w1493 w1653]
          tunnel: [w1493 w1674] -> w1476
          tunnel: w1475 -> [w1494 _]
          tunnel: w1474 -> [_ w1662]
          tunnel: w1473 -> [_ w1645]
          tunnel: w1472 -> [_ _]
          frame False {
            n683 = flat-sequence {
              frame #0 {
              }
            }
            n684 = local read "All Labels (USB6210)"() -> (w1482:string[])
            n685 = Multiply(x="N for sampling", y=i64 2) -> (x*y=w1488:i64)
            n686 = local read "Cycle #"() -> (w1492:u32)
            n687 = Search 1D Array(1D array=w1482, element="Auto Fll\nDewar P. label") -> (index of element=→"Target Index (P)":i32)  [unwired: 1 in]
            n688 = Search 1D Array(1D array=w1482, element="Auto Fll\nHe level label") -> (index of element=→"Target Index (L)":i32)  [unwired: 1 in]
            n689 = Add(x=w1488, y="Mov. Avg Interval") -> (x+y=w1490:i64)
            n690 = Greater?(x=w1492, y=w1490) -> (0:w1486:bool)
            n691 = And(x=w1486, y="Auto Fill ON?") -> (x .and. y?=w1484:bool)
            n692 = case shown="True" w1484 {
              tunnel: w1494 -> [_ w1525]
              tunnel: "Mov. Avg Interval" -> [_ w1509]
              tunnel: w1488 -> [_ w1495]
              tunnel: "N for sampling" -> [_ w1507]
              frame False {
              }
              frame True {
                n693 = local read "Pstd"() -> (→"Pstd history":dbl)
                n694 = local read "Lstd"() -> (→"Lstd history":dbl)
                n695 = local read "Pav (Pa)"() -> (→"Pav history":dbl)
                n696 = local read "Lav (%)"() -> (→"Lav history":dbl)
                n697 = local read "Target Index (P)"() -> (w1526:i32)
                n698 = local read "Target Index (L)"() -> (w1512:i32)
                n699 = Unbundle By Name(w1525) -> ("TimeArray"=w1523:timestamp[], "DataArrayConv"=w1524:dbl[][])
                n700 = Index Array(array=w1524, index (col) #1=w1526, index (col) #2=w1512) -> (element #1=w1511:dbl[], element #2=w1506:dbl[])  [unwired: 2 in]
                n701 = Delete From Array(array=w1511, length=w1495) -> (deleted portion=w1520:dbl[])  [unwired: 1 in, 1 out]
                n702 = Delete From Array(array=w1506, length=w1495) -> (deleted portion=w1505:dbl[])  [unwired: 1 in, 1 out]
                n703 = call "MovingAverage.vi"("Moving Average interval"=w1509, "Input Array"=w1506) -> ("M.A. Array"=w1508:dbl[])  [unwired: 9 in]
                n704 = call "MovingAverage.vi"("Moving Average interval"=w1509, "Input Array"=w1511) -> ("M.A. Array"=w1510:dbl[])  [unwired: 9 in]
                n705 = Delete From Array(array=w1510, length=w1495) -> (deleted portion=w1521:dbl[])  [unwired: 1 in, 1 out]
                n706 = Delete From Array(array=w1510, length=w1495) -> (deleted portion=w1517:dbl[])  [unwired: 1 in, 1 out]
                "Last N M.A. Pressures" <- w1517
                n707 = Delete From Array(array=w1508, length=w1495) -> (deleted portion=w1500:dbl[])  [unwired: 1 in, 1 out]
                "Last N M.A. Levels" <- w1500
                n708 = Delete From Array(array=w1523, length=w1495) -> (deleted portion=w1502:timestamp[])  [unwired: 1 in, 1 out]
                n709 = Bundle("TimeArray"=w1502, "DataArrayConv"=w1520) -> (w1519:T23)  [unwired: 1 in]
                n710 = Bundle("TimeArray"=w1502, "M.A. Array"=w1521) -> (w1522:T24)  [unwired: 1 in]
                n711 = Bundle("TimeArray"=w1502, "DataArrayConv"=w1505) -> (w1504:T23)  [unwired: 1 in]
                n712 = Bundle("TimeArray"=w1502, "M.A. Array"=w1500) -> (w1501:T24)  [unwired: 1 in]
                n713 = Array Size(array=w1517) -> (size(s)=w1516:i32)
                n714 = Greater Or Equal?(x=w1516, y=w1507) -> (x >= y?=w1515:bool)
                n715 = Build Array(w1519, w1522) -> (→"Dewar Pressure":T25)
                n716 = Build Array(w1504, w1501) -> (→"He Level":T25)
                n717 = case shown="True" w1515 {
                  tunnel: [w1630 w1635] -> w1499
                  tunnel: w1517 -> [_ w1636]
                  tunnel: w1500 -> [_ w1633]
                  tunnel: [w1630 w1631] -> w1498
                  frame False {
                    w1630 = nan ("mean")
                  }
                  frame True {
                    n718 = call <vilib>:"Std Deviation and Variance.vi"("X"=w1636) -> ("mean"=w1635:dbl, "standard deviation"=w1634:dbl)  [unwired: 1 in, 1 out]
                    n719 = call <vilib>:"Std Deviation and Variance.vi"("X"=w1633) -> ("mean"=w1631:dbl, "standard deviation"=w1632:dbl)  [unwired: 1 in, 1 out]
                    n720 = local write "Pstd"(w1634) -> ()
                    n721 = local write "Lstd"(w1632) -> ()
                    n722 = local write "Pav (Pa)"(w1635) -> ()
                    n723 = local write "Lav (%)"(w1631) -> ()
                  }
                }
                n724 = flat-sequence {
                  tunnel: w1499 -> [w1527]
                  tunnel: w1498 -> [w1528]
                  frame #0 {
                    n725 = flat-sequence {
                      tunnel: w1528 -> [w1530]
                      tunnel: w1527 -> [w1529]
                      tunnel: w1527 -> [w1598]
                      frame #0 {
                        n726 = stacked-sequence {
                          tunnel: w1530 -> [w1537 w1541 _ _ _ _]
                          tunnel: w1529 -> [_ _ w1555 w1564 w1573 w1582]
                          frame #0 {
                            n727 = local read "L_low (%)"() -> (w1536:dbl)
                            n728 = local read "Fill state"() -> (w1534:bool)
                            n729 = Less?(x=w1537, y=w1536) -> (x < y?=w1533:bool)
                            n730 = Equal?(x=w1534, y=FALSE) -> (x = y?=w1532:bool)
                            n731 = And(x=w1533, y=w1532) -> (x .and. y?=w1531:bool)
                            n732 = case shown="False" w1531 {
                              frame False {
                              }
                              frame True {
                                w1539 = TRUE ("Value (Signaling)")
                                n733 = property on="Fill state" class="Bool (strict)"("Val(Sgnl)"=w1539) -> ()  [unwired: 2 in, 2 out]
                                n734 = Not(x=w1539) -> (.not. x?=w1538:bool)
                                n735 = property on="Fill (false)" class="Bool (strict)"("Val(Sgnl)"=w1538) -> ()  [unwired: 2 in, 2 out]
                              }
                            }
                          }
                          frame #1 {
                            n736 = local read "L_high (%)"() -> (w1542:dbl)
                            n737 = local read "Fill state"() -> (w1545:bool)
                            n738 = Greater?(x=w1541, y=w1542) -> (0:w1540:bool)
                            n739 = Equal?(x=w1545, y=TRUE) -> (x = y?=w1544:bool)
                            n740 = And(x=w1540, y=w1544) -> (x .and. y?=w1543:bool)
                            n741 = case shown="True" w1543 {
                              frame False {
                              }
                              frame True {
                                w1547 = FALSE ("Value (Signaling)")
                                n742 = property on="Fill state" class="Bool (strict)"("Val(Sgnl)"=w1547) -> ()  [unwired: 2 in, 2 out]
                                n743 = Not(x=w1547) -> (.not. x?=w1548:bool)
                                n744 = property on="Fill (false)" class="Bool (strict)"("Val(Sgnl)"=w1548) -> ()  [unwired: 2 in, 2 out]
                              }
                            }
                          }
                          frame #2 {
                            n745 = local read "P_1_low (Pa)"() -> (w1554:dbl)
                            n746 = property on="state 1" class="Bool (strict)"() -> ("Value"=w1552:bool)  [unwired: 2 in, 2 out]
                            n747 = Less?(x=w1555, y=w1554) -> (x < y?=w1551:bool)
                            n748 = Equal?(x=w1552, y=FALSE) -> (x = y?=w1550:bool)
                            n749 = And(x=w1550, y=w1551) -> (x .and. y?=w1549:bool)
                            n750 = case shown="True" w1549 {
                              frame False {
                              }
                              frame True {
                                w1557 = TRUE ("Value (Signaling)")
                                n751 = property on="state 1" class="Bool (strict)"("Val(Sgnl)"=w1557) -> ()  [unwired: 2 in, 2 out]
                                n752 = Not(x=w1557) -> (.not. x?=w1556:bool)
                                n753 = property on="state 1 (false)" class="Bool (strict)"("Val(Sgnl)"=w1556) -> ()  [unwired: 2 in, 2 out]
                              }
                            }
                          }
                          frame #3 {
                            n754 = local read "P_1_high (Pa)"() -> (w1563:dbl)
                            n755 = property on="state 1" class="Bool (strict)"() -> ("Value"=w1561:bool)  [unwired: 2 in, 2 out]
                            n756 = Greater?(x=w1564, y=w1563) -> (0:w1560:bool)
                            n757 = Equal?(x=w1561, y=TRUE) -> (x = y?=w1559:bool)
                            n758 = And(x=w1559, y=w1560) -> (x .and. y?=w1558:bool)
                            n759 = case shown="True" w1558 {
                              frame False {
                              }
                              frame True {
                                w1566 = FALSE ("Value (Signaling)")
                                n760 = property on="state 1" class="Bool (strict)"("Val(Sgnl)"=w1566) -> ()  [unwired: 2 in, 2 out]
                                n761 = Not(x=w1566) -> (.not. x?=w1565:bool)
                                n762 = property on="state 1 (false)" class="Bool (strict)"("Val(Sgnl)"=w1565) -> ()  [unwired: 2 in, 2 out]
                              }
                            }
                          }
                          frame #4 {
                            n763 = local read "P_2_low (Pa)"() -> (w1572:dbl)
                            n764 = property on="state 2" class="Bool (strict)"() -> ("Value"=w1567:bool)  [unwired: 2 in, 2 out]
                            n765 = Less?(x=w1573, y=w1572) -> (x < y?=w1570:bool)
                            n766 = Equal?(x=w1567, y=FALSE) -> (x = y?=w1569:bool)
                            n767 = And(x=w1569, y=w1570) -> (x .and. y?=w1568:bool)
                            n768 = case shown="True" w1568 {
                              frame False {
                              }
                              frame True {
                                w1574 = TRUE ("Value (Signaling)")
                                n769 = property on="state 2" class="Bool (strict)"("Val(Sgnl)"=w1574) -> ()  [unwired: 2 in, 2 out]
                                n770 = Not(x=w1574) -> (.not. x?=w1575:bool)
                                n771 = property on="state 2 (false)" class="Bool (strict)"("Val(Sgnl)"=w1575) -> ()  [unwired: 2 in, 2 out]
                              }
                            }
                          }
                          frame #5 {
                            n772 = local read "P_2_high (Pa)"() -> (w1581:dbl)
                            n773 = property on="state 2" class="Bool (strict)"() -> ("Value"=w1576:bool)  [unwired: 2 in, 2 out]
                            n774 = Greater?(x=w1582, y=w1581) -> (0:w1579:bool)
                            n775 = Equal?(x=w1576, y=TRUE) -> (x = y?=w1578:bool)
                            n776 = And(x=w1578, y=w1579) -> (x .and. y?=w1577:bool)
                            n777 = case shown="True" w1577 {
                              frame False {
                              }
                              frame True {
                                w1583 = FALSE ("Value (Signaling)")
                                n778 = property on="state 2" class="Bool (strict)"("Val(Sgnl)"=w1583) -> ()  [unwired: 2 in, 2 out]
                                n779 = Not(x=w1583) -> (.not. x?=w1584:bool)
                                n780 = property on="state 2 (false)" class="Bool (strict)"("Val(Sgnl)"=w1584) -> ()  [unwired: 2 in, 2 out]
                              }
                            }
                          }
                        }
                      }
                      frame #1 {
                        n781 = property on="Fill state" class="Bool (strict)"() -> ("Value"=w1585:bool)  [unwired: 2 in, 2 out]
                        n782 = case shown="True" w1585 {
                          frame False {
                            n783 = property on="V1 (N.O.)" class="Bool (strict)"("Val(Sgnl)"=TRUE ("V1 (N.O.)")) -> ()  [unwired: 2 in, 2 out]
                            n784 = property on="V2 (N.C.)" class="Bool (strict)"("Val(Sgnl)"=FALSE ("Value (Signaling)")) -> ()  [unwired: 2 in, 2 out]
                          }
                          frame True {
                            n785 = property on="state 1" class="Bool (strict)"() -> ("Value"=w1589:bool)  [unwired: 2 in, 2 out]
                            n786 = property on="state 2" class="Bool (strict)"() -> ("Value"=w1588:bool)  [unwired: 2 in, 2 out]
                            n787 = case shown="True" w1589 {
                              frame False {
                                n788 = property on="V1 (N.O.)" class="Bool (strict)"("Val(Sgnl)"=TRUE ("Value (Signaling)")) -> ()  [unwired: 2 in, 2 out]
                                n789 = local write "Status V1 CTRL"(enum16{"Pressurize", "Release"}."Release" ("Status V1 CTRL")) -> ()
                              }
                              frame True {
                                n790 = property on="V1 (N.O.)" class="Bool (strict)"("Val(Sgnl)"=FALSE ("V1 (N.O.)")) -> ()  [unwired: 2 in, 2 out]
                                n791 = local write "Status V1 CTRL"(enum16{"Pressurize", "Release"}."Pressurize" ("Status V1 CTRL")) -> ()
                              }
                            }
                            n792 = case shown="True" w1588 {
                              frame False {
                                n793 = property on="V2 (N.C.)" class="Bool (strict)"("Val(Sgnl)"=FALSE ("Value (Signaling)")) -> ()  [unwired: 2 in, 2 out]
                                n794 = local write "Status V2 CTRL"(enum16{"Pressurize", "Release"}."Release" ("Status V2 CTRL")) -> ()
                              }
                              frame True {
                                n795 = property on="V2 (N.C.)" class="Bool (strict)"("Val(Sgnl)"=TRUE ("Value (Signaling)")) -> ()  [unwired: 2 in, 2 out]
                                n796 = local write "Status V2 CTRL"(enum16{"Pressurize", "Release"}."Pressurize" ("Status V2 CTRL")) -> ()
                              }
                            }
                          }
                        }
                      }
                      frame #2 {
                        n797 = Greater?(x=w1598, y="P_safelimit_high (Pa)") -> (0:w1600:bool)
                        n798 = Less?(x=w1598, y="P_safelimit_low (Pa)") -> (x < y?=w1602:bool)
                        n799 = Or(x=w1600, y=w1602) -> (x .or. y?=w1603:bool)
                        n800 = case shown="False" w1603 {
                          frame False {
                          }
                          frame True {
                            w1604 = FALSE ("Value (Signaling)")
                            w1606 = FALSE ("Value (Signaling)")
                            n801 = property on="V2 (N.C.)" class="Bool (strict)"("Val(Sgnl)"=FALSE ("V1 (N.O.)")) -> ()  [unwired: 2 in, 2 out]
                            n802 = property on="state 1" class="Bool (strict)"("Val(Sgnl)"=w1604) -> ()  [unwired: 2 in, 2 out]
                            n803 = property on="V1 (N.O.)" class="Bool (strict)"("Val(Sgnl)"=TRUE ("V1 (N.O.)")) -> ()  [unwired: 2 in, 2 out]
                            n804 = property on="state 2" class="Bool (strict)"("Val(Sgnl)"=w1606) -> ()  [unwired: 2 in, 2 out]
                            n805 = Not(x=w1604) -> (.not. x?=w1605:bool)
                            n806 = Not(x=w1606) -> (.not. x?=w1607:bool)
                            n807 = property on="state 1 (false)" class="Bool (strict)"("Val(Sgnl)"=w1605) -> ()  [unwired: 2 in, 2 out]
                            n808 = property on="state 2 (false)" class="Bool (strict)"("Val(Sgnl)"=w1607) -> ()  [unwired: 2 in, 2 out]
                          }
                        }
                      }
                    }
                  }
                  frame #1 {
                    n809 = property on="V2 (N.C.)" class="Bool (strict)"() -> ("Value"=w1617:bool)  [unwired: 2 in, 2 out]
                    n810 = property on="V1 (N.O.)" class="Bool (strict)"() -> ("Value"=w1628:bool)  [unwired: 2 in, 2 out]
                    n811 = local read "P_1_high (Pa)"() -> (w1622:dbl)
                    n812 = local read "P_2_high (Pa)"() -> (w1620:dbl)
                    n813 = local read "P_1_low (Pa)"() -> (w1623:dbl)
                    n814 = local read "P_2_low (Pa)"() -> (w1621:dbl)
                    n815 = local read "L_high (%)"() -> (w1618:dbl)
                    n816 = local read "L_low (%)"() -> (w1619:dbl)
                    n817 = local read "Pav (Pa)"() -> (w1611:dbl)
                    n818 = local read "Lav (%)"() -> (w1610:dbl)
                    n819 = Boolean To (0,1)(Boolean=w1617) -> (0, 1=w1616:i16)
                    n820 = Boolean To (0,1)(Boolean=w1628) -> (0, 1=w1629:i16)
                    n821 = local read "File Refn DewarCTRL"() -> (w1624:refnum<file>)
                    n822 = local read "Cycle #"() -> (w1627:u32)
                    n823 = Build Array(w1611, w1610, w1623, w1622, w1621, w1620, w1619, w1618, w1629, w1616) -> (w1615:dbl[])
                    n824 = Get Date/Time In Seconds() -> (seconds since 1Jan1904=w1625:timestamp)
                    n825 = call "FileWrite.vi"("DataArray"=w1615, "Time Stamp"=w1625, "Error In"=errorcluster {"status"=FALSE, "code"=0, "source"=""}, "FileFormat"=string[] ["%4.5e", "%4.2f", "%4.4e", "%4.4e", "%4.4e", "%4.4e", "%4.4e", "%d", "%d"] ("Array"), "Index"=w1627, "refnum in"=w1624) -> ("Error Out"=→"Error Out (Dewar CTRL":errorcluster, "Byte Stream File Refnum"=w1614:refnum<file>)  [unwired: 4 in]
                    n826 = local write "File Refn DewarCTRL"(w1614) -> ()
                  }
                }
              }
            }
          }
          frame True {
            w1668 = "_"
            w1637 = FALSE ("auto cleanup")
            w1673 = 1 items=["one channel for each line", "one channel for all lines"] ("line grouping")
            n827 = flat-sequence {
              frame #0 {
                w1688 = FALSE ("V1 (N.O.)")
                n828 = local write "V2 (N.C.)"(FALSE ("V1 (N.O.)")) -> ()
                n829 = local write "V1 (N.O.)"(TRUE ("V1 (N.O.)")) -> ()
                n830 = local write "state 2"(w1688) -> ()
                n831 = local write "state 1"(w1688) -> ()
                n832 = local write "Fill state"(w1688) -> ()
                n833 = Not(x=w1688) -> (.not. x?=w1690:bool)
                n834 = Not(x=w1688) -> (.not. x?=w1689:bool)
                n835 = local write "state 1 (false)"(w1689) -> ()
                n836 = local write "state 2 (false)"(w1689) -> ()
                n837 = local write "Fill (false)"(w1690) -> ()
              }
            }
            n838 = Get Date/Time In Seconds() -> (seconds since 1Jan1904=w1685:timestamp)
            n839 = call "LV_UNIXTIME.vi"("current time"=w1685) -> ("date/time string"=w1663:string)  [unwired: 9 in, 1 out]
            n840 = Concatenate Strings(w1663, "_DO" ("new task name")) -> (w1682:string)
            n841 = Concatenate Strings(w1662, w1668, w1663, w1668) -> (w1644:string)
            n842 = Concatenate Strings(w1644, "DEWAR.csv" ("string")) -> (w1643:string)
            n843 = Concatenate Strings(w1644, "USB_DOUT.csv" ("string")) -> (w1647:string)
            n844 = Build Path(base path=w1645, name or relative path=w1643) -> (appended path=w1642:path)
            n845 = Build Path(base path=w1645, name or relative path=w1647) -> (appended path=w1667:path)
            n846 = Open/Create/Replace File(file path (use dialog)=w1667, error in=w1653, operation (0:open)=T19."open or create") -> (refnum out=w1665:refnum<file>, error out=w1652:errorcluster)  [unwired: 3 in, 1 out]
            n847 = call "FileIntialize.vi"("Error In"=w1652, "Labels"="DOUT Labels", "refnum in"=w1665) -> ("Error Out"=w1639:errorcluster, "File Refnum"=→"File Refn USB DO":refnum<file>)  [unwired: 7 in]
            n848 = Open/Create/Replace File(file path (use dialog)=w1642, error in=w1639, operation (0:open)=T19."open or create") -> (refnum out=w1650:refnum<file>, error out=w1651:errorcluster)  [unwired: 3 in, 1 out]
            n849 = call "FileIntialize.vi"("Error In"=w1651, "Labels"=string[] ["P_av", "L_av", "P_1_low", "P_1_high", "P_2_low", "P_2_high", "L_low", "L_high", "V1(NO)", "V2(NC)"], "refnum in"=w1650) -> ("Error Out"=w1638:errorcluster, "File Refnum"=→"File Refn DewarCTRL":refnum<file>)  [unwired: 7 in]
            n850 = Index Array(array="DOUT Physical CH", index=2) -> (element=w1655:tag)
            n851 = Index Array(array="DOUT Physical CH", index=1) -> (element=w1658:tag)
            n852 = Index Array(array="DOUT Physical CH", index=0) -> (element=w1660:tag)
            n853 = call <vilib>:"DAQmx Create Task.vi"("new task name"=w1682, "auto cleanup"=FALSE, "error in"=w1638) -> ("task out"=w1683:refnum<k21>, "error out"=w1684:errorcluster)  [unwired: 11 in]
            n854 = call-poly <vilib>:"DAQmx Create Virtual Channel.vi"("task in"=w1683, "lines"=w1660, "line grouping"=w1673, "error in"=w1684) -> ("task out"=w1686:refnum<k21>, "error out"=w1687:errorcluster)  [unwired: 10 in]
            n855 = call-poly <vilib>:"DAQmx Create Virtual Channel.vi"("task in"=w1686, "lines"=w1658, "line grouping"=w1673, "error in"=w1687) -> ("task out"=w1672:refnum<k21>, "error out"=w1670:errorcluster)  [unwired: 10 in]
            n856 = call-poly <vilib>:"DAQmx Create Virtual Channel.vi"("task in"=w1672, "lines"=w1655, "line grouping"=w1673, "error in"=w1670) -> ("task out"=w1671:refnum<k21>, "error out"=w1669:errorcluster)  [unwired: 10 in]
            n857 = call <vilib>:"DAQmx Start Task.vi"("task/channels in"=w1671, "error in"=w1669) -> ("task out"=w1677:refnum<k21>, "error out"=w1675:errorcluster)  [unwired: 12 in]
            n858 = Build Array(w1637, w1637, w1637) -> (w1678:bool[])
            n859 = call <vilib>:"DAQmx Write (Digital 1D Bool NChan 1Samp 1Line).vi"("task/channels in"=w1677, "data"=w1678, "timeout"=10.0, "error in"=w1675) -> ("task out"=→"DOUT task out":refnum<k21>, "error out"=w1674:errorcluster)  [unwired: 9 in, 1 out]
          }
        }
      }
    }
    "error out (USB6210/6218 DOUT)" <- w806
    n860 = flat-sequence {
      tunnel: w801 -> [w1274]
      tunnel: [w1269] -> w800
      tunnel: [w1267] -> w799
      tunnel: [w1266] -> w798
      tunnel: [w1265] -> w797
      tunnel: w802 -> [w1261]
      frame #0 {
        w1268 = T20 [] ("appended array")
        n861 = Unbundle By Name(w1261) -> ("TimeArray"=w1257:timestamp[], "DataArrayConv"=w1272:dbl[][], "LDArray"=w1271:dbl[])
        "TimeArray (USB6218)" <- w1257
        n862 = Unbundle By Name(w1274) -> ("ReadLeakDet?"=w1273:bool, "LabelLD"=w1276:string, "Labels"=w1270:string[])  [unwired: 1 out]
        n863 = case shown="True" w1273 {
          tunnel: w1276 -> [_ w1284]
          tunnel: w1272 -> [w1278 w1283]
          tunnel: w1271 -> [_ w1282]
          tunnel: [w1278 w1281] -> w1259
          tunnel: w1270 -> [w1277 w1280]
          tunnel: [w1277 w1279] -> w1262
          frame False {
          }
          frame True {
            n864 = Build Array (concatenate)(w1283, w1282) -> (w1281:dbl[][])
            n865 = Build Array (concatenate)(w1280, w1284) -> (w1279:string[])
          }
        }
        "All Labels (USB6218)" <- w1262
        "DataArrayConv (USB6218)" <- w1259
        n866 = Array Size(array=w1257) -> (size(s)=→"TimeArray size (6218)":i32)
        n867 = local read "Plot selecter (USB6218)\n    1      2     3     4"() -> (w1264:bool[][])
        n868 = control-ref of="Plot selecter (USB6218)\n    1      2     3     4"() -> (w1260:refnum<vi>)
        n869 = Array Size(array=w1262) -> (size(s)=w1263:i32)
        n870 = Array Size(array=w1262) -> (size(s)=w1275:i32)
        n871 = Array Size(array=w1259) -> (size(s)=→"DataArraySize (6218)":i32[])
        n872 = property on="Property Node" class="Arr (strict)"(reference=w1260, "Number of Rows"=w1263) -> ()  [unwired: 1 in, 2 out]
        n873 = for {
          N: w1275 -> [_]
          tunnel: w1259 -> [w1305]
          tunnel: w1257 -> [w1306]
          shift-right: [w1300] -> w1267
          shift-left: w1268 -> [w1303]
          shift-right: [w1298] -> w1265
          shift-left: w1268 -> [w1301]
          shift-right: [w1299] -> w1269
          shift-left: w1268 -> [w1297]
          shift-right: [w1296] -> w1266
          shift-left: w1268 -> [w1295]
          tunnel: w1264 -> [w1294]
          i -> [w1289]
          n874 = Index Array(array=w1305, index (col)=w1289) -> (element=w1304:dbl[])  [unwired: 1 in]
          n875 = Index Array(array=w1294, index (row) #1=w1289, index (col) #1=0 ("index (row)"), index (row) #2=w1289, index (col) #2=1 ("index (row)"), index (row) #3=w1289, index (col) #3=2 ("index (row)"), index (row) #4=w1289, index (col) #4=3 ("index (row)")) -> (element #1=w1288:bool, element #2=w1287:bool, element #3=w1286:bool, element #4=w1285:bool)
          n876 = Bundle("TimeArray"=w1306, "DataArrayConv"=w1304) -> (w1302:T23)  [unwired: 1 in]
          n877 = stacked-sequence {
            tunnel: w1288 -> [w1310 _ _ _]
            tunnel: w1303 -> [_ w1318 _ _]
            tunnel: w1286 -> [_ _ w1326 _]
            tunnel: w1302 -> [w1307 w1316 w1325 w1331]
            tunnel: w1285 -> [_ _ _ w1334]
            tunnel: w1301 -> [_ _ _ w1333]
            tunnel: [_ _ _ w1332] -> w1298
            tunnel: [_ w1317 _ _] -> w1300
            tunnel: [w1309 _ _ _] -> w1299
            tunnel: w1297 -> [w1308 _ _ _]
            tunnel: [_ _ w1324 _] -> w1296
            tunnel: w1295 -> [_ _ w1323 _]
            tunnel: w1287 -> [_ w1315 _ _]
            frame #0 {
              n878 = case shown="True" w1310 {
                tunnel: [w1311 w1314] -> w1309
                tunnel: w1307 -> [_ w1313]
                tunnel: w1308 -> [w1311 w1312]
                frame False {
                }
                frame True {
                  n879 = Build Array (concatenate)(w1312, w1313) -> (w1314:T20)
                }
              }
            }
            frame #1 {
              n880 = case shown="True" w1315 {
                tunnel: w1318 -> [w1319 w1322]
                tunnel: [w1319 w1321] -> w1317
                tunnel: w1316 -> [_ w1320]
                frame False {
                }
                frame True {
                  n881 = Build Array (concatenate)(w1322, w1320) -> (w1321:T20)
                }
              }
            }
            frame #2 {
              n882 = case shown="True" w1326 {
                tunnel: [w1327 w1330] -> w1324
                tunnel: w1325 -> [_ w1329]
                tunnel: w1323 -> [w1327 w1328]
                frame False {
                }
                frame True {
                  n883 = Build Array (concatenate)(w1328, w1329) -> (w1330:T20)
                }
              }
            }
            frame #3 {
              n884 = case shown="True" w1334 {
                tunnel: [w1335 w1338] -> w1332
                tunnel: w1331 -> [_ w1337]
                tunnel: w1333 -> [w1335 w1336]
                frame False {
                }
                frame True {
                  n885 = Build Array (concatenate)(w1336, w1337) -> (w1338:T20)
                }
              }
            }
          }
        }
      }
    }
    n886 = Build Array (concatenate)(w770, w771) -> (w768:dbl[])
    n887 = Build Array (concatenate)(w773, w772) -> (w769:string[])
    n888 = local read "Plot selecter LSI218(2)\n    1      2     3     4"() -> (w828:bool[][])
    n889 = local read "Plot selecter LSI218(1)\n    1      2     3     4"() -> (w829:bool[][])
    n890 = for {
      N: 48 -> [_]
      tunnel: w844 -> [w1792]
      tunnel: w843 -> [w1789]
      tunnel: w829 -> [w1773]
      tunnel: w828 -> [w1774]
      shift-right: [w1790] -> w842
      shift-left: w840 -> [w1791]
      shift-right: [w1785] -> w837
      shift-left: w840 -> [w1786]
      shift-right: [w1784] -> w835
      shift-left: w840 -> [w1783]
      shift-right: [w1782] -> w833
      shift-left: w840 -> [w1781]
      i -> [w1779]
      n891 = Index Array(array=w1789, index (col)=w1779) -> (element=w1788:dbl[])  [unwired: 1 in]
      n892 = Less?(x=w1779, y=24) -> (x < y?=w1780:bool)
      n893 = case shown="True" w1780 {
        tunnel: [w1797 w1815] -> w1778
        tunnel: [w1796 w1814] -> w1777
        tunnel: [w1795 w1812] -> w1776
        tunnel: [w1794 w1811] -> w1775
        tunnel: w1773 -> [_ w1810]
        tunnel: w1774 -> [w1804 _]
        tunnel: w1779 -> [w1799 w1807]
        frame False {
          n894 = Subtract(x=w1799, y=24) -> (x-y=w1803:i32)
          n895 = Index Array(array=w1804, index (row) #1=w1803, index (col) #1=0 ("index (row)"), index (row) #2=w1803, index (col) #2=1 ("index (row)"), index (row) #3=w1803, index (col) #3=2 ("index (row)"), index (row) #4=w1803, index (col) #4=3 ("index (row)")) -> (element #1=w1797:bool, element #2=w1796:bool, element #3=w1795:bool, element #4=w1794:bool)
        }
        frame True {
          n896 = Index Array(array=w1810, index (row) #1=w1807, index (col) #1=0 ("index (row)"), index (row) #2=w1807, index (col) #2=1 ("index (row)"), index (row) #3=w1807, index (col) #3=2 ("index (row)"), index (row) #4=w1807, index (col) #4=3 ("index (row)")) -> (element #1=w1815:bool, element #2=w1814:bool, element #3=w1812:bool, element #4=w1811:bool)
        }
      }
      n897 = Bundle("TimeArray"=w1792, "DataArray"=w1788) -> (w1787:T26)  [unwired: 1 in]
      n898 = stacked-sequence {
        tunnel: w1791 -> [w1819 _ _ _]
        tunnel: [w1818 _ _ _] -> w1790
        tunnel: w1787 -> [w1817 w1827 w1835 w1843]
        tunnel: w1786 -> [_ w1826 _ _]
        tunnel: [_ w1825 _ _] -> w1785
        tunnel: [_ _ w1834 _] -> w1784
        tunnel: w1783 -> [_ _ w1833 _]
        tunnel: [_ _ _ w1842] -> w1782
        tunnel: w1781 -> [_ _ _ w1841]
        tunnel: w1778 -> [w1816 _ _ _]
        tunnel: w1777 -> [_ w1824 _ _]
        tunnel: w1776 -> [_ _ w1832 _]
        tunnel: w1775 -> [_ _ _ w1840]
        frame #0 {
          n899 = case shown="False" w1816 {
            tunnel: w1817 -> [_ w1821]
            tunnel: w1819 -> [w1820 w1823]
            tunnel: [w1820 w1822] -> w1818
            frame False {
            }
            frame True {
              n900 = Build Array (concatenate)(w1823, w1821) -> (w1822:T1)
            }
          }
        }
        frame #1 {
          n901 = case shown="True" w1824 {
            tunnel: [w1828 w1831] -> w1825
            tunnel: w1827 -> [_ w1830]
            tunnel: w1826 -> [w1828 w1829]
            frame False {
            }
            frame True {
              n902 = Build Array (concatenate)(w1829, w1830) -> (w1831:T1)
            }
          }
        }
        frame #2 {
          n903 = case shown="True" w1832 {
            tunnel: [w1836 w1839] -> w1834
            tunnel: w1835 -> [_ w1838]
            tunnel: w1833 -> [w1836 w1837]
            frame False {
            }
            frame True {
              n904 = Build Array (concatenate)(w1837, w1838) -> (w1839:T1)
            }
          }
        }
        frame #3 {
          n905 = case shown="True" w1840 {
            tunnel: [w1844 w1847] -> w1842
            tunnel: w1843 -> [_ w1846]
            tunnel: w1841 -> [w1844 w1845]
            frame False {
            }
            frame True {
              n906 = Build Array (concatenate)(w1845, w1846) -> (w1847:T1)
            }
          }
        }
      }
    }
    n907 = local read "Labels LSI336"() -> (w816:string[])
    n908 = Array Size(array=w816) -> (size(s)=w815:i32)
    n909 = local read "Plot selecter LSI336 \n     1      2     3     4"() -> (w824:bool[][])
    n910 = for {
      N: w815 -> [_]
      tunnel: w824 -> [w1705]
      shift-right: [w1699] -> w822
      shift-left: w823 -> [w1714]
      shift-right: [w1695] -> w821
      shift-left: w823 -> [w1712]
      shift-right: [w1696] -> w820
      shift-left: w823 -> [w1711]
      shift-right: [w1694] -> w819
      shift-left: w823 -> [w1710]
      tunnel: w784 -> [w1702]
      tunnel: w786 -> [w1700]
      i -> [w1703]
      n911 = Index Array(array=w1702, index (col)=w1703) -> (element=w1701:dbl[])  [unwired: 1 in]
      n912 = Index Array(array=w1705, index (row) #1=w1703, index (col) #1=0 ("index (row)"), index (row) #2=w1703, index (col) #2=1 ("index (row)"), index (row) #3=w1703, index (col) #3=2 ("index (row)"), index (row) #4=w1703, index (col) #4=3 ("index (row)")) -> (element #1=w1704:bool, element #2=w1698:bool, element #3=w1697:bool, element #4=w1693:bool)
      n913 = Bundle("TimeArray"=w1700, "DataArray"=w1701) -> (w1713:T26)  [unwired: 1 in]
      n914 = stacked-sequence {
        tunnel: w1714 -> [w1718 _ _ _]
        tunnel: [w1717 _ _ _] -> w1699
        tunnel: w1713 -> [w1716 w1726 w1734 w1742]
        tunnel: w1712 -> [_ w1725 _ _]
        tunnel: [_ w1724 _ _] -> w1695
        tunnel: [_ _ w1733 _] -> w1696
        tunnel: w1711 -> [_ _ w1732 _]
        tunnel: [_ _ _ w1741] -> w1694
        tunnel: w1710 -> [_ _ _ w1740]
        tunnel: w1704 -> [w1715 _ _ _]
        tunnel: w1698 -> [_ w1723 _ _]
        tunnel: w1697 -> [_ _ w1731 _]
        tunnel: w1693 -> [_ _ _ w1739]
        frame #0 {
          n915 = case shown="False" w1715 {
            tunnel: w1716 -> [_ w1720]
            tunnel: w1718 -> [w1719 w1722]
            tunnel: [w1719 w1721] -> w1717
            frame False {
            }
            frame True {
              n916 = Build Array (concatenate)(w1722, w1720) -> (w1721:T1)
            }
          }
        }
        frame #1 {
          n917 = case shown="True" w1723 {
            tunnel: [w1727 w1730] -> w1724
            tunnel: w1726 -> [_ w1728]
            tunnel: w1725 -> [w1727 w1729]
            frame False {
            }
            frame True {
              n918 = Build Array (concatenate)(w1729, w1728) -> (w1730:T1)
            }
          }
        }
        frame #2 {
          n919 = case shown="True" w1731 {
            tunnel: [w1735 w1738] -> w1733
            tunnel: w1734 -> [_ w1736]
            tunnel: w1732 -> [w1735 w1737]
            frame False {
            }
            frame True {
              n920 = Build Array (concatenate)(w1737, w1736) -> (w1738:T1)
            }
          }
        }
        frame #3 {
          n921 = case shown="True" w1739 {
            tunnel: [w1743 w1746] -> w1741
            tunnel: w1742 -> [_ w1744]
            tunnel: w1740 -> [w1743 w1745]
            frame False {
            }
            frame True {
              n922 = Build Array (concatenate)(w1745, w1744) -> (w1746:T1)
            }
          }
        }
      }
    }
    n923 = Array Size(array=w786) -> (size(s)=→"TimeArray Size (336)":i32)
    n924 = Array Size(array=w784) -> (size(s)=→"DataArray size (336)":i32[])
    n925 = Build Array (concatenate)(w836, w835, w820, w798) -> (→"Graph 3":T20)
    n926 = Build Array (concatenate)(w841, w842, w822, w800) -> (→"Graph 1":T20)
    n927 = Build Array (concatenate)(w839, w837, w821, w799) -> (→"Graph 2":T20)
    n928 = Build Array (concatenate)(w834, w833, w819, w797) -> (→"Graph 4":T20)
    n929 = Send Notification(notification="Stop Button", notifier=w758, error in (no error)=w757) -> (notifier out=w754:refnum<notifier>, error out=w755:errorcluster)
    "Cycle #" <- w767
  }
  n930 = while {
    shift-right: [w1941] -> _
    shift-left: refnum<class "DMMsData.lvclass"> refnum ("DMMsData in") -> [w1940]
    tunnel: errorcluster {"status"=FALSE, "code"=0, "source"=""} ("error in (no error)") -> [w1939]
    shift-right: [w1938] -> _
    shift-left: _ -> [_]
    tunnel: w3 -> [w1936]
    tunnel: w2 -> [w1935]
    tunnel: [w1934] -> w1
    i -> [w1937]
    stop <- w1933 stop-if-true
    n931 = Wait (ms)(milliseconds to wait="Measurement Interval DMMs (ms)") -> ()  [unwired: 1 out]
    n932 = Equal?(x=w1937, y=0) -> (x = y?=w1942:bool)
    n933 = case shown="True" "Measure DMMs?" {
      tunnel: w1942 -> [_ w1953]
      tunnel: [w1946 w1951] -> w1941
      tunnel: w1940 -> [w1946 w1950]
      tunnel: w1939 -> [w1945 w1949]
      tunnel: [w1945 w1948] -> w1938
      tunnel: w1937 -> [_ w1947]
      frame False {
      }
      frame True {
        n934 = Or(x="Initialize (DMMs)", y=w1953) -> (x .or. y?=w1952:bool)
        n935 = case shown="False" w1952 {
          tunnel: w1950 -> [w1968 w1985]
          tunnel: [w1965 w1984] -> w1951
          tunnel: w1949 -> [w1967 w1980]
          tunnel: [w1966 w1976] -> w1948
          tunnel: w1947 -> [w1964 _]
          frame False {
            n936 = local read "DMMsConfig"() -> (w1960:T10)
            n937 = call-dynamic "DMMs_measure.vi"("Sample #"="Sample #", "error in (no error)"=w1967, "MeasurementIndex"=w1964, "DMMsData in"=w1968) -> ("error out"=w1966:errorcluster, "DataArray"=w1958:dbl[][], "LastData"=→"DMM LastMeasurements":dbl[], "DMMsData out"=w1965:refnum<class "DMMsData.lvclass">, "DeviceActive?"=→"Active?":bool[], "TimeArray"=w1963:timestamp[])  [unwired: 2 in]
            n938 = Array Size(array=w1960) -> (size(s)=w1959:i32)
            n939 = for {
              N: w1959 -> [_]
              tunnel: w1963 -> [w1971]
              tunnel: w1958 -> [w1975]
              shift-right: [w1969] -> w1956
              shift-left: T1 [] -> [w1970]
              i -> [w1974]
              n940 = Index Array(array=w1975, index (col)=w1974) -> (element=w1973:dbl[])  [unwired: 1 in]
              n941 = Bundle("TimeArray"=w1971, "DataArray"=w1973) -> (w1972:T26)  [unwired: 1 in]
              n942 = Build Array (concatenate)(w1970, w1972) -> (w1969:T1)
            }
            "Graph DMMs 2" <- w1956
            "Graph DMMs 1" <- w1956
          }
          frame True {
            n943 = local write "Initialize (DMMs)"(FALSE ("Initialize 2")) -> ()
            n944 = local read "RUN Identifier"() -> (w1979:string)
            n945 = local read "Base Path"() -> (w1981:path)
            n946 = call-dynamic "DMMs_initialize.vi"("DMMsConfig"=w1979, "InstName"="InstName DMMs", "error in (no error)"=w1980, "base path"=w1981, "RunIdentifier"="DMMsConfig", "DMMsData in"=w1985) -> ("error out"=w1976:errorcluster, "DMMsLabels"=w1977:string[], "FileName"=→"DMMFileName":string, "DMMsData out"=w1984:refnum<class "DMMsData.lvclass">)  [unwired: 1 in, 1 out]
            "DMMsLabels" <- w1977
            n947 = stacked-sequence {
              tunnel: w1977 -> [w1987 w2010]
              frame #0 {
                n948 = Array Size(array=w1987) -> (size(s)=w1996:i32)
                n949 = control-ref of="Graph DMMs 1"() -> (w1993:refnum<vi>)
                n950 = property class="XYGraph (strict)"(reference=w1993, error in=errorcluster {"status"=FALSE, "code"=0, "source"=""} ("error in (no error)")) -> (reference out=w1989:refnum<vi>, error out=w1992:errorcluster, "LegNumRows"=w1994:u32)
                n951 = for {
                  N: w1994 -> [_]
                  shift-right: [w2005] -> w1995
                  shift-left: w1992 -> [w2006]
                  tunnel: w1989 -> [w2004]
                  tunnel: [w2003] -> w1988 mode=indexing
                  i -> [w2008]
                  n952 = property class="XYGraph (strict)"(reference=w2004, error in=w2006, "Active Plot"=w2008, "Plot.Plot Name"="") -> (reference out=w2003:refnum<vi>, error out=w2005:errorcluster)
                }
                n953 = for {
                  N: w1996 -> [_]
                  shift-right: [w2000] -> w1990
                  shift-left: w1995 -> [w2001]
                  tunnel: w1988 -> [w1998] mode=indexing
                  tunnel: w1987 -> [w1997] mode=indexing
                  i -> [w2002]
                  n954 = property class="XYGraph (strict)"(reference=w1998, error in=w2001, "Active Plot"=w2002, "Plot.Plot Name"=w1997, "Plot.Visible?"=TRUE ("Plot.Visible")) -> (error out=w2000:errorcluster)  [unwired: 1 out]
                }
                "error out (DMM graphs)" <- w1990
              }
              frame #1 {
                n955 = Array Size(array=w2010) -> (size(s)=w2018:i32)
                n956 = control-ref of="Graph DMMs 2"() -> (w2013:refnum<vi>)
                n957 = property class="XYGraph (strict)"(reference=w2013, error in=errorcluster {"status"=FALSE, "code"=0, "source"=""} ("error in (no error)")) -> (reference out=w2012:refnum<vi>, error out=w2015:errorcluster, "LegNumRows"=w2016:u32)
                n958 = for {
                  N: w2016 -> [_]
                  shift-right: [w2027] -> w2017
                  shift-left: w2015 -> [w2028]
                  tunnel: w2012 -> [w2026]
                  tunnel: [w2025] -> w2011 mode=indexing
                  i -> [w2030]
                  n959 = property class="XYGraph (strict)"(reference=w2026, error in=w2028, "Active Plot"=w2030, "Plot.Plot Name"="") -> (reference out=w2025:refnum<vi>, error out=w2027:errorcluster)
                }
                n960 = for {
                  N: w2018 -> [_]
                  shift-right: [w2022] -> w2009
                  shift-left: w2017 -> [w2023]
                  tunnel: w2011 -> [w2020] mode=indexing
                  tunnel: w2010 -> [w2019] mode=indexing
                  i -> [w2024]
                  n961 = property class="XYGraph (strict)"(reference=w2020, error in=w2023, "Active Plot"=w2024, "Plot.Plot Name"=w2019, "Plot.Visible?"=TRUE ("Plot.Visible")) -> (error out=w2022:errorcluster)  [unwired: 1 out]
                }
                n962 = local write "error out (DMM graphs)"(w2009) -> ()
              }
            }
          }
        }
        "error out (DMMs)" <- w1948
      }
    }
    n963 = Get Notifier Status(notifier=w1936, error in (no error)=w1935) -> (current notification=w1933:bool, error out=w1934:errorcluster)  [unwired: 3 out]
    "cycle # (DMMs)" <- w1937
  }
  n964 = Merge Errors(w1, w5) -> (w6:errorcluster)
  n965 = Release Notifier(notifier=w4, error in (no error)=w6) -> (error out=→"error out (notifier)":errorcluster)  [unwired: 1 in, 2 out]
  n966 = call-dynamic "USBData_terminate.vi"("error in (no error)"=w35, "USBData in"=w36) -> ("error out"=w37:errorcluster)  [unwired: 8 in, 1 out]
  n967 = call-dynamic "LSI336Data_terminate.vi"("error in (no error)"=w25, "LSI336Data in"=w26) -> ("error out"=w24:errorcluster)  [unwired: 8 in, 1 out]
  n968 = call-dynamic "USBData_terminate.vi"("error in (no error)"=w18, "USBData in"=w19) -> ("error out"=w20:errorcluster)  [unwired: 8 in, 1 out]
  n969 = call "LSI218Data_terminate.vi"("error in (no error)"=w29, "LSI218Data in"=w30) -> ("error out"=w28:errorcluster)  [unwired: 8 in, 1 out]
  n970 = local write "error out (USB6210)"(w37) -> ()
  n971 = local write "error out (LSI336)"(w24) -> ()
  n972 = local write "error out (USB6210)"(w20) -> ()
  n973 = local write "error out (LSI218)"(w28) -> ()
